vi "all signals list_search worksheet.vi"() -> ()   [LabVIEW 2020]
panel:
  out "path not found":bool
  in  "signal/tag name":string="RX_deltatime"
  out "full path name":string
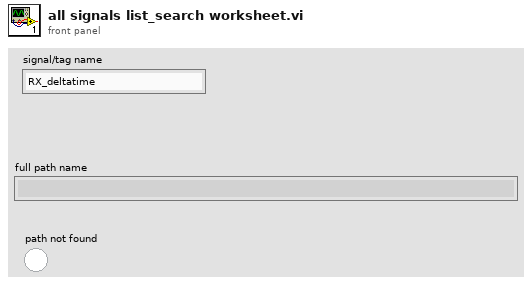
[diagram p1: front panel]
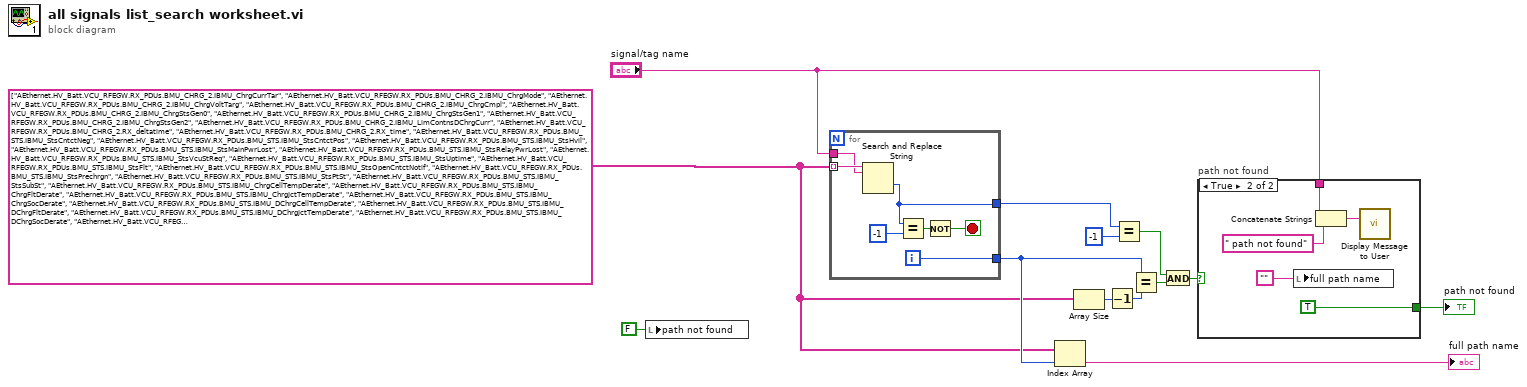
[diagram p0: block diagram]
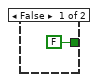
[diagram p2: hidden frame]
diagram:
  w1 = string[] ["AEthernet.HV_Batt.VCU_RFEGW.RX_PDUs.BMU_CHRG_2.IBMU_ChrgCurrTar", "AEthernet.HV_Batt.VCU_RFEGW.RX_PDUs.BMU_CHRG_2.IBMU_ChrgMode", "AEthernet.HV_Batt.VCU_RFEGW.RX_PDUs.BMU_CHRG_2.IBMU_ChrgVoltTarg", "AEthernet.HV_Batt.VCU_RFEGW.RX_PDUs.BMU_CHRG_2.IBMU_ChrgCmpl", "AEthernet.HV_Batt.VCU_RFEGW.RX_PDUs.BMU_CHRG_2.IBMU_ChrgStsGen0", "AEthernet.HV_Batt.VCU_RFEGW.RX_PDUs.BMU_CHRG_2.IBMU_ChrgStsGen1", "AEthernet.HV_Batt.VCU_RFEGW.RX_PDUs.BMU_CHRG_2.IBMU_ChrgStsGen2", "AEthernet.HV_Batt.VCU_RFEGW.RX_PDUs.BMU_CHRG_2.IBMU_LimContnsDChrgCurr", "AEthernet.HV_Batt.VCU_RFEGW.RX_PDUs.BMU_CHRG_2.RX_deltatime", "AEthernet.HV_Batt.VCU_RFEGW.RX_PDUs.BMU_CHRG_2.RX_time", "AEthernet.HV_Batt.VCU_RFEGW.RX_PDUs.BMU_STS.IBMU_StsCntctNeg", "AEthernet.HV_Batt.VCU_RFEGW.RX_PDUs.BMU_STS.IBMU_StsCntctPos", "AEthernet.HV_Batt.VCU_RFEGW.RX_PDUs.BMU_STS.IBMU_StsHvil", "AEthernet.HV_Batt.VCU_RFEGW.RX_PDUs.BMU_STS.IBMU_StsMainPwrLost", "AEthernet.HV_Batt.VCU_RFEGW.RX_PDUs.BMU_STS.IBMU_StsRelayPwrLost", "AEthernet.HV_Batt.VCU_RFEGW.RX_PDUs.BMU_STS.IBMU_StsVcuStReq", "AEthernet.HV_Batt.VCU_RFEGW.RX_PDUs.BMU_STS.IBMU_StsUptime", "AEthernet.HV_Batt.VCU_RFEGW.RX_PDUs.BMU_STS.IBMU_StsFlt", "AEthernet.HV_Batt.VCU_RFEGW.RX_PDUs.BMU_STS.IBMU_StsOpenCntctNotif", "AEthernet.HV_Batt.VCU_RFEGW.RX_PDUs.BMU_STS.IBMU_StsPrechrgn", "AEthernet.HV_Batt.VCU_RFEGW.RX_PDUs.BMU_STS.IBMU_StsPtSt", "AEthernet.HV_Batt.VCU_RFEGW.RX_PDUs.BMU_STS.IBMU_StsSubSt", "AEthernet.HV_Batt.VCU_RFEGW.RX_PDUs.BMU_STS.IBMU_ChrgCellTempDerate", "AEthernet.HV_Batt.VCU_RFEGW.RX_PDUs.BMU_STS.IBMU_ChrgFltDerate", "AEthernet.HV_Batt.VCU_RFEGW.RX_PDUs.BMU_STS.IBMU_ChrgJctTempDerate", "AEthernet.HV_Batt.VCU_RFEGW.RX_PDUs.BMU_STS.IBMU_ChrgSocDerate", "AEthernet.HV_Batt.VCU_RFEGW.RX_PDUs.BMU_STS.IBMU_DChrgCellTempDerate", "AEthernet.HV_Batt.VCU_RFEGW.RX_PDUs.BMU_STS.IBMU_DChrgFltDerate", "AEthernet.HV_Batt.VCU_RFEGW.RX_PDUs.BMU_STS.IBMU_DChrgJctTempDerate", "AEthernet.HV_Batt.VCU_RFEGW.RX_PDUs.BMU_STS.IBMU_DChrgSocDerate", "AEthernet.HV_Batt.VCU_RFEGW.RX_PDUs.BMU_STS.RX_deltatime", "AEthernet.HV_Batt.VCU_RFEGW.RX_PDUs.BMU_STS.RX_time", "AEthernet.HV_Batt.TCU.RX_PDUs.BMU_CHRG_2.IBMU_ChrgCurrTar", "AEthernet.HV_Batt.TCU.RX_PDUs.BMU_CHRG_2.IBMU_ChrgMode", "AEthernet.HV_Batt.TCU.RX_PDUs.BMU_CHRG_2.IBMU_ChrgVoltTarg", "AEthernet.HV_Batt.TCU.RX_PDUs.BMU_CHRG_2.IBMU_ChrgCmpl", "AEthernet.HV_Batt.TCU.RX_PDUs.BMU_CHRG_2.IBMU_ChrgStsGen0", "AEthernet.HV_Batt.TCU.RX_PDUs.BMU_CHRG_2.IBMU_ChrgStsGen1", "AEthernet.HV_Batt.TCU.RX_PDUs.BMU_CHRG_2.IBMU_ChrgStsGen2", "AEthernet.HV_Batt.TCU.RX_PDUs.BMU_CHRG_2.IBMU_LimContnsDChrgCurr", "AEthernet.HV_Batt.TCU.RX_PDUs.BMU_CHRG_2.RX_deltatime", "AEthernet.HV_Batt.TCU.RX_PDUs.BMU_CHRG_2.RX_time", "AEthernet.HV_Batt.TCU.RX_PDUs.BMU_CHRG_3.IBMU_LimMaxChrgCurr", "AEthernet.HV_Batt.TCU.RX_PDUs.BMU_CHRG_3.IBMU_LimMaxChrgPwr", "AEthernet.HV_Batt.TCU.RX_PDUs.BMU_CHRG_3.IBMU_LimMaxChrgVolt", "AEthernet.HV_Batt.TCU.RX_PDUs.BMU_CHRG_3.IBMU_LimMinChrgCurr", "AEthernet.HV_Batt.TCU.RX_PDUs.BMU_CHRG_3.RX_deltatime", "AEthernet.HV_Batt.TCU.RX_PDUs.BMU_CHRG_3.RX_time", "AEthernet.HV_Batt.TCU.RX_PDUs.BMU_DIAG_RESP.IDiagRspRes1", "AEthernet.HV_Batt.TCU.RX_PDUs.BMU_DIAG_RESP.IDiagRspRes2", "AEthernet.HV_Batt.TCU.RX_PDUs.BMU_DIAG_RESP.IDiagRspRes3", "AEthernet.HV_Batt.TCU.RX_PDUs.BMU_DIAG_RESP.IDiagRspRes4", "AEthernet.HV_Batt.TCU.RX_PDUs.BMU_DIAG_RESP.IDiagRspRes5", "AEthernet.HV_Batt.TCU.RX_PDUs.BMU_DIAG_RESP.IDiagRspRes6", "AEthernet.HV_Batt.TCU.RX_PDUs.BMU_DIAG_RESP.IDiagRspRes7", "AEthernet.HV_Batt.TCU.RX_PDUs.BMU_DIAG_RESP.IDiagRspRoutId", "AEthernet.HV_Batt.TCU.RX_PDUs.BMU_DIAG_RESP.IDiagRspSts", "AEthernet.HV_Batt.TCU.RX_PDUs.BMU_DIAG_RESP.RX_deltatime", "AEthernet.HV_Batt.TCU.RX_PDUs.BMU_DIAG_RESP.RX_time", "AEthernet.HV_Batt.TCU.RX_PDUs.BMU_DbgGen_1.IBMU_DbgGen_B0", "AEthernet.HV_Batt.TCU.RX_PDUs.BMU_DbgGen_1.IBMU_DbgGen_B1", "AEthernet.HV_Batt.TCU.RX_PDUs.BMU_DbgGen_1.IBMU_DbgGen_B2", "AEthernet.HV_Batt.TCU.RX_PDUs.BMU_DbgGen_1.IBMU_DbgGen_B3", "AEthernet.HV_Batt.TCU.RX_PDUs.BMU_DbgGen_1.IBMU_DbgGen_B4", "AEthernet.HV_Batt.TCU.RX_PDUs.BMU_DbgGen_1.IBMU_DbgGen_B5", "AEthernet.HV_Batt.TCU.RX_PDUs.BMU_DbgGen_1.IBMU_DbgGen_B6", "AEthernet.HV_Batt.TCU.RX_PDUs.BMU_DbgGen_1.IBMU_DbgGen_B7", "AEthernet.HV_Batt.TCU.RX_PDUs.BMU_DbgGen_1.IBMU_DbgGen_B8", "AEthernet.HV_Batt.TCU.RX_PDUs.BMU_DbgGen_1.IBMU_DbgGen_B9", "AEthernet.HV_Batt.TCU.RX_PDUs.BMU_DbgGen_1.IBMU_DbgGen_L0", "AEthernet.HV_Batt.TCU.RX_PDUs.BMU_DbgGen_1.IBMU_DbgGen_L1", "AEthernet.HV_Batt.TCU.RX_PDUs.BMU_DbgGen_1.IBMU_DbgGen_L2", "AEthernet.HV_Batt.TCU.RX_PDUs.BMU_DbgGen_1.IBMU_DbgGen_L3", "AEthernet.HV_Batt.TCU.RX_PDUs.BMU_DbgGen_1.IBMU_DbgGen_S0", "AEthernet.HV_Batt.TCU.RX_PDUs.BMU_DbgGen_1.IBMU_DbgGen_S1", "AEthernet.HV_Batt.TCU.RX_PDUs.BMU_DbgGen_1.IBMU_DbgGen_S2", "AEthernet.HV_Batt.TCU.RX_PDUs.BMU_DbgGen_1.IBMU_DbgGen_S3", "AEthernet.HV_Batt.TCU.RX_PDUs.BMU_DbgGen_1.IBMU_DbgGen_S4", "AEthernet.HV_Batt.TCU.RX_PDUs.BMU_DbgGen_1.IBMU_DbgGen_S5", "AEthernet.HV_Batt.TCU.RX_PDUs.BMU_DbgGen_1.IBMU_DbgGen_S6", "AEthernet.HV_Batt.TCU.RX_PDUs.BMU_DbgGen_1.IBMU_DbgGen_S7", "AEthernet.HV_Batt.TCU.RX_PDUs.BMU_DbgGen_1.IBMU_DbgGen_S8", "AEthernet.HV_Batt.TCU.RX_PDUs.BMU_DbgGen_1.IBMU_DbgGen_S9", "AEthernet.HV_Batt.TCU.RX_PDUs.BMU_DbgGen_1.IBMU_DbgGen_W00", "AEthernet.HV_Batt.TCU.RX_PDUs.BMU_DbgGen_1.IBMU_DbgGen_W01", "AEthernet.HV_Batt.TCU.RX_PDUs.BMU_DbgGen_1.IBMU_DbgGen_W02", "AEthernet.HV_Batt.TCU.RX_PDUs.BMU_DbgGen_1.IBMU_DbgGen_W03", "AEthernet.HV_Batt.TCU.RX_PDUs.BMU_DbgGen_1.IBMU_DbgGen_W04", "AEthernet.HV_Batt.TCU.RX_PDUs.BMU_DbgGen_1.IBMU_DbgGen_W05", "AEthernet.HV_Batt.TCU.RX_PDUs.BMU_DbgGen_1.IBMU_DbgGen_W06", "AEthernet.HV_Batt.TCU.RX_PDUs.BMU_DbgGen_1.IBMU_DbgGen_W07", "AEthernet.HV_Batt.TCU.RX_PDUs.BMU_DbgGen_1.IBMU_DbgGen_W08", "AEthernet.HV_Batt.TCU.RX_PDUs.BMU_DbgGen_1.IBMU_DbgGen_W09", "AEthernet.HV_Batt.TCU.RX_PDUs.BMU_DbgGen_1.IBMU_DbgGen_W10", "AEthernet.HV_Batt.TCU.RX_PDUs.BMU_DbgGen_1.IBMU_DbgGen_W11", "AEthernet.HV_Batt.TCU.RX_PDUs.BMU_DbgGen_1.IBMU_DbgGen_W12", "AEthernet.HV_Batt.TCU.RX_PDUs.BMU_DbgGen_1.IBMU_DbgGen_W13", "AEthernet.HV_Batt.TCU.RX_PDUs.BMU_DbgGen_1.IBMU_DbgGen_W14", "AEthernet.HV_Batt.TCU.RX_PDUs.BMU_DbgGen_1.IBMU_DbgGen_W15", "AEthernet.HV_Batt.TCU.RX_PDUs.BMU_DbgGen_1.RX_deltatime", "AEthernet.HV_Batt.TCU.RX_PDUs.BMU_DbgGen_1.RX_time", "AEthernet.HV_Batt.TCU.RX_PDUs.BMU_DbgGen_2.IBMU_DbgIsoSampleVneg", "AEthernet.HV_Batt.TCU.RX_PDUs.BMU_DbgGen_2.IBMU_DbgIsoSampleVpos", "AEthernet.HV_Batt.TCU.RX_PDUs.BMU_DbgGen_2.IBMU_DbgIsoSampleVsum", "AEthernet.HV_Batt.TCU.RX_PDUs.BMU_DbgGen_2.IBMU_DbgGen_W16", "AEthernet.HV_Batt.TCU.RX_PDUs.BMU_DbgGen_2.IBMU_DbgGen_W17", "AEthernet.HV_Batt.TCU.RX_PDUs.BMU_DbgGen_2.IBMU_DbgGen_W18", "AEthernet.HV_Batt.TCU.RX_PDUs.BMU_DbgGen_2.IBMU_DbgGen_W19", "AEthernet.HV_Batt.TCU.RX_PDUs.BMU_DbgGen_2.IBMU_DbgPktRetryCnt", "AEthernet.HV_Batt.TCU.RX_PDUs.BMU_DbgGen_2.RX_deltatime", "AEthernet.HV_Batt.TCU.RX_PDUs.BMU_DbgGen_2.RX_time", "AEthernet.HV_Batt.TCU.RX_PDUs.BMU_DbgVers.IBMU_DbgHw", "AEthernet.HV_Batt.TCU.RX_PDUs.BMU_DbgVers.IBMU_DbgSwMajor", "AEthernet.HV_Batt.TCU.RX_PDUs.BMU_DbgVers.IBMU_DbgSwMicro", "AEthernet.HV_Batt.TCU.RX_PDUs.BMU_DbgVers.IBMU_DbgSwMinor", "AEthernet.HV_Batt.TCU.RX_PDUs.BMU_DbgVers.IBMU_DbgFpgaMajor", "AEthernet.HV_Batt.TCU.RX_PDUs.BMU_DbgVers.IBMU_DbgFpgaMinor", "AEthernet.HV_Batt.TCU.RX_PDUs.BMU_DbgVers.IBMU_StatsPkSrlNum", "AEthernet.HV_Batt.TCU.RX_PDUs.BMU_DbgVers.IBMU_DbgTsuMaxMajor", "AEthernet.HV_Batt.TCU.RX_PDUs.BMU_DbgVers.IBMU_DbgTsuMaxMicro", "AEthernet.HV_Batt.TCU.RX_PDUs.BMU_DbgVers.IBMU_DbgTsuMaxMinor", "AEthernet.HV_Batt.TCU.RX_PDUs.BMU_DbgVers.IBMU_DbgTsuMaxRels", "AEthernet.HV_Batt.TCU.RX_PDUs.BMU_DbgVers.IBMU_DbgTsuMinMajor", "AEthernet.HV_Batt.TCU.RX_PDUs.BMU_DbgVers.IBMU_DbgTsuMinMicro", "AEthernet.HV_Batt.TCU.RX_PDUs.BMU_DbgVers.IBMU_DbgTsuMinMinor", "AEthernet.HV_Batt.TCU.RX_PDUs.BMU_DbgVers.IBMU_DbgTsuMinRels", "AEthernet.HV_Batt.TCU.RX_PDUs.BMU_DbgVers.RX_deltatime", "AEthernet.HV_Batt.TCU.RX_PDUs.BMU_DbgVers.RX_time", "AEthernet.HV_Batt.TCU.RX_PDUs.BMU_FLT_1.IBMU_FltAcb", "AEthernet.HV_Batt.TCU.RX_PDUs.BMU_FLT_1.IBMU_FltBlkVoltOver", "AEthernet.HV_Batt.TCU.RX_PDUs.BMU_FLT_1.IBMU_FltBlkVoltUnder", "AEthernet.HV_Batt.TCU.RX_PDUs.BMU_FLT_1.IBMU_FltConds", "AEthernet.HV_Batt.TCU.RX_PDUs.BMU_FLT_1.IBMU_FltHvil", "AEthernet.HV_Batt.TCU.RX_PDUs.BMU_FLT_1.IBMU_FltIso", "AEthernet.HV_Batt.TCU.RX_PDUs.BMU_FLT_1.IBMU_FltModCnt", "AEthernet.HV_Batt.TCU.RX_PDUs.BMU_FLT_1.IBMU_FltPkCurrOver", "AEthernet.HV_Batt.TCU.RX_PDUs.BMU_FLT_1.IBMU_FltPkCurrUnder", "AEthernet.HV_Batt.TCU.RX_PDUs.BMU_FLT_1.IBMU_FltPkVoltOver", "AEthernet.HV_Batt.TCU.RX_PDUs.BMU_FLT_1.IBMU_FltPkVoltUnder", "AEthernet.HV_Batt.TCU.RX_PDUs.BMU_FLT_1.IBMU_FltPrechrg", "AEthernet.HV_Batt.TCU.RX_PDUs.BMU_FLT_1.IBMU_FltStSenClsd", "AEthernet.HV_Batt.TCU.RX_PDUs.BMU_FLT_1.IBMU_FltTempCellOver", "AEthernet.HV_Batt.TCU.RX_PDUs.BMU_FLT_1.IBMU_FltTempCellUnder", "AEthernet.HV_Batt.TCU.RX_PDUs.BMU_FLT_1.IBMU_FltTempInterconOver", "AEthernet.HV_Batt.TCU.RX_PDUs.BMU_FLT_1.IBMU_FltBlkVoltDelta", "AEthernet.HV_Batt.TCU.RX_PDUs.BMU_FLT_1.IBMU_FltStSenOpen", "AEthernet.HV_Batt.TCU.RX_PDUs.BMU_FLT_1.IBMU_StsFltHist1", "AEthernet.HV_Batt.TCU.RX_PDUs.BMU_FLT_1.IBMU_StsFltHist2", "AEthernet.HV_Batt.TCU.RX_PDUs.BMU_FLT_1.IBMU_StsFltHist3", "AEthernet.HV_Batt.TCU.RX_PDUs.BMU_FLT_1.IBMU_DbgRstSrc", "AEthernet.HV_Batt.TCU.RX_PDUs.BMU_FLT_1.IBMU_FltCntctHlth", "AEthernet.HV_Batt.TCU.RX_PDUs.BMU_FLT_1.IBMU_FltCrash", "AEthernet.HV_Batt.TCU.RX_PDUs.BMU_FLT_1.IBMU_FltPOver", "AEthernet.HV_Batt.TCU.RX_PDUs.BMU_FLT_1.IBMU_FltPyro", "AEthernet.HV_Batt.TCU.RX_PDUs.BMU_FLT_1.IBMU_FltShunt", "AEthernet.HV_Batt.TCU.RX_PDUs.BMU_FLT_1.IBMU_FltSpi", "AEthernet.HV_Batt.TCU.RX_PDUs.BMU_FLT_1.RX_deltatime", "AEthernet.HV_Batt.TCU.RX_PDUs.BMU_FLT_1.RX_time", "AEthernet.HV_Batt.TCU.RX_PDUs.BMU_FLT_2.IBMU_HsFltLogEstopTrckrSt", "AEthernet.HV_Batt.TCU.RX_PDUs.BMU_FLT_2.IBMU_HsFltLogPyroFired", "AEthernet.HV_Batt.TCU.RX_PDUs.BMU_FLT_2.IBMU_HsFltLogPyroStsBad", "AEthernet.HV_Batt.TCU.RX_PDUs.BMU_FLT_2.IBMU_HsFltLogRawEstop", "AEthernet.HV_Batt.TCU.RX_PDUs.BMU_FLT_2.IBMU_HsFltLogRawCurr", "AEthernet.HV_Batt.TCU.RX_PDUs.BMU_FLT_2.IBMU_HsFltLogReserved1", "AEthernet.HV_Batt.TCU.RX_PDUs.BMU_FLT_2.IBMU_HsFltLogReserved2", "AEthernet.HV_Batt.TCU.RX_PDUs.BMU_FLT_2.RX_deltatime", "AEthernet.HV_Batt.TCU.RX_PDUs.BMU_FLT_2.RX_time", "AEthernet.HV_Batt.TCU.RX_PDUs.BMU_MODBLKVOLT.IBMU_ModBlkVolt_M00B00", "AEthernet.HV_Batt.TCU.RX_PDUs.BMU_MODBLKVOLT.IBMU_ModBlkVolt_M00B01", "AEthernet.HV_Batt.TCU.RX_PDUs.BMU_MODBLKVOLT.IBMU_ModBlkVolt_M00B02", "AEthernet.HV_Batt.TCU.RX_PDUs.BMU_MODBLKVOLT.IBMU_ModBlkVolt_M00B03", "AEthernet.HV_Batt.TCU.RX_PDUs.BMU_MODBLKVOLT.IBMU_ModBlkVolt_M00B04", "AEthernet.HV_Batt.TCU.RX_PDUs.BMU_MODBLKVOLT.IBMU_ModBlkVolt_M00B05", "AEthernet.HV_Batt.TCU.RX_PDUs.BMU_MODBLKVOLT.IBMU_ModBlkVolt_M00B06", "AEthernet.HV_Batt.TCU.RX_PDUs.BMU_MODBLKVOLT.IBMU_ModBlkVolt_M00B07", "AEthernet.HV_Batt.TCU.RX_PDUs.BMU_MODBLKVOLT.IBMU_ModBlkVolt_M00B08", "AEthernet.HV_Batt.TCU.RX_PDUs.BMU_MODBLKVOLT.IBMU_ModBlkVolt_M00B09", "AEthernet.HV_Batt.TCU.RX_PDUs.BMU_MODBLKVOLT.IBMU_ModBlkVolt_M01B00", "AEthernet.HV_Batt.TCU.RX_PDUs.BMU_MODBLKVOLT.IBMU_ModBlkVolt_M01B01", "AEthernet.HV_Batt.TCU.RX_PDUs.BMU_MODBLKVOLT.IBMU_ModBlkVolt_M01B02", "AEthernet.HV_Batt.TCU.RX_PDUs.BMU_MODBLKVOLT.IBMU_ModBlkVolt_M01B03", "AEthernet.HV_Batt.TCU.RX_PDUs.BMU_MODBLKVOLT.IBMU_ModBlkVolt_M01B04", "AEthernet.HV_Batt.TCU.RX_PDUs.BMU_MODBLKVOLT.IBMU_ModBlkVolt_M01B05", "AEthernet.HV_Batt.TCU.RX_PDUs.BMU_MODBLKVOLT.IBMU_ModBlkVolt_M01B06", "AEthernet.HV_Batt.TCU.RX_PDUs.BMU_MODBLKVOLT.IBMU_ModBlkVolt_M01B07", "AEthernet.HV_Batt.TCU.RX_PDUs.BMU_MODBLKVOLT.IBMU_ModBlkVolt_M01B08", "AEthernet.HV_Batt.TCU.RX_PDUs.BMU_MODBLKVOLT.IBMU_ModBlkVolt_M01B09", "AEthernet.HV_Batt.TCU.RX_PDUs.BMU_MODBLKVOLT.IBMU_ModBlkVolt_M02B00", "AEthernet.HV_Batt.TCU.RX_PDUs.BMU_MODBLKVOLT.IBMU_ModBlkVolt_M02B01", "AEthernet.HV_Batt.TCU.RX_PDUs.BMU_MODBLKVOLT.IBMU_ModBlkVolt_M02B02", "AEthernet.HV_Batt.TCU.RX_PDUs.BMU_MODBLKVOLT.IBMU_ModBlkVolt_M02B03", "AEthernet.HV_Batt.TCU.RX_PDUs.BMU_MODBLKVOLT.IBMU_ModBlkVolt_M02B04", "AEthernet.HV_Batt.TCU.RX_PDUs.BMU_MODBLKVOLT.IBMU_ModBlkVolt_M02B05", "AEthernet.HV_Batt.TCU.RX_PDUs.BMU_MODBLKVOLT.IBMU_ModBlkVolt_M02B06", "AEthernet.HV_Batt.TCU.RX_PDUs.BMU_MODBLKVOLT.IBMU_ModBlkVolt_M02B07", "AEthernet.HV_Batt.TCU.RX_PDUs.BMU_MODBLKVOLT.IBMU_ModBlkVolt_M02B08", "AEthernet.HV_Batt.TCU.RX_PDUs.BMU_MODBLKVOLT.IBMU_ModBlkVolt_M02B09", "AEthernet.HV_Batt.TCU.RX_PDUs.BMU_MODBLKVOLT.IBMU_ModBlkVolt_M03B00", "AEthernet.HV_Batt.TCU.RX_PDUs.BMU_MODBLKVOLT.IBMU_ModBlkVolt_M03B01", "AEthernet.HV_Batt.TCU.RX_PDUs.BMU_MODBLKVOLT.IBMU_ModBlkVolt_M03B02", "AEthernet.HV_Batt.TCU.RX_PDUs.BMU_MODBLKVOLT.IBMU_ModBlkVolt_M03B03", "AEthernet.HV_Batt.TCU.RX_PDUs.BMU_MODBLKVOLT.IBMU_ModBlkVolt_M03B04", "AEthernet.HV_Batt.TCU.RX_PDUs.BMU_MODBLKVOLT.IBMU_ModBlkVolt_M03B05", "AEthernet.HV_Batt.TCU.RX_PDUs.BMU_MODBLKVOLT.IBMU_ModBlkVolt_M03B06", "AEthernet.HV_Batt.TCU.RX_PDUs.BMU_MODBLKVOLT.IBMU_ModBlkVolt_M03B07", "AEthernet.HV_Batt.TCU.RX_PDUs.BMU_MODBLKVOLT.IBMU_ModBlkVolt_M03B08", "AEthernet.HV_Batt.TCU.RX_PDUs.BMU_MODBLKVOLT.IBMU_ModBlkVolt_M03B09", "AEthernet.HV_Batt.TCU.RX_PDUs.BMU_MODBLKVOLT.IBMU_ModBlkVolt_M04B00", "AEthernet.HV_Batt.TCU.RX_PDUs.BMU_MODBLKVOLT.IBMU_ModBlkVolt_M04B01", "AEthernet.HV_Batt.TCU.RX_PDUs.BMU_MODBLKVOLT.IBMU_ModBlkVolt_M04B02", "AEthernet.HV_Batt.TCU.RX_PDUs.BMU_MODBLKVOLT.IBMU_ModBlkVolt_M04B03", "AEthernet.HV_Batt.TCU.RX_PDUs.BMU_MODBLKVOLT.IBMU_ModBlkVolt_M04B04", "AEthernet.HV_Batt.TCU.RX_PDUs.BMU_MODBLKVOLT.IBMU_ModBlkVolt_M04B05", "AEthernet.HV_Batt.TCU.RX_PDUs.BMU_MODBLKVOLT.IBMU_ModBlkVolt_M04B06", "AEthernet.HV_Batt.TCU.RX_PDUs.BMU_MODBLKVOLT.IBMU_ModBlkVolt_M04B07", "AEthernet.HV_Batt.TCU.RX_PDUs.BMU_MODBLKVOLT.IBMU_ModBlkVolt_M04B08", "AEthernet.HV_Batt.TCU.RX_PDUs.BMU_MODBLKVOLT.IBMU_ModBlkVolt_M04B09", "AEthernet.HV_Batt.TCU.RX_PDUs.BMU_MODBLKVOLT.IBMU_ModBlkVolt_M05B00", "AEthernet.HV_Batt.TCU.RX_PDUs.BMU_MODBLKVOLT.IBMU_ModBlkVolt_M05B01", "AEthernet.HV_Batt.TCU.RX_PDUs.BMU_MODBLKVOLT.IBMU_ModBlkVolt_M05B02", "AEthernet.HV_Batt.TCU.RX_PDUs.BMU_MODBLKVOLT.IBMU_ModBlkVolt_M05B03", "AEthernet.HV_Batt.TCU.RX_PDUs.BMU_MODBLKVOLT.IBMU_ModBlkVolt_M05B04", "AEthernet.HV_Batt.TCU.RX_PDUs.BMU_MODBLKVOLT.IBMU_ModBlkVolt_M05B05", "AEthernet.HV_Batt.TCU.RX_PDUs.BMU_MODBLKVOLT.IBMU_ModBlkVolt_M05B06", "AEthernet.HV_Batt.TCU.RX_PDUs.BMU_MODBLKVOLT.IBMU_ModBlkVolt_M05B07", "AEthernet.HV_Batt.TCU.RX_PDUs.BMU_MODBLKVOLT.IBMU_ModBlkVolt_M05B08", "AEthernet.HV_Batt.TCU.RX_PDUs.BMU_MODBLKVOLT.IBMU_ModBlkVolt_M05B09", "AEthernet.HV_Batt.TCU.RX_PDUs.BMU_MODBLKVOLT.IBMU_ModBlkVolt_M06B00", "AEthernet.HV_Batt.TCU.RX_PDUs.BMU_MODBLKVOLT.IBMU_ModBlkVolt_M06B01", "AEthernet.HV_Batt.TCU.RX_PDUs.BMU_MODBLKVOLT.IBMU_ModBlkVolt_M06B02", "AEthernet.HV_Batt.TCU.RX_PDUs.BMU_MODBLKVOLT.IBMU_ModBlkVolt_M06B03", "AEthernet.HV_Batt.TCU.RX_PDUs.BMU_MODBLKVOLT.IBMU_ModBlkVolt_M06B04", "AEthernet.HV_Batt.TCU.RX_PDUs.BMU_MODBLKVOLT.IBMU_ModBlkVolt_M06B05", "AEthernet.HV_Batt.TCU.RX_PDUs.BMU_MODBLKVOLT.IBMU_ModBlkVolt_M06B06", "AEthernet.HV_Batt.TCU.RX_PDUs.BMU_MODBLKVOLT.IBMU_ModBlkVolt_M06B07", "AEthernet.HV_Batt.TCU.RX_PDUs.BMU_MODBLKVOLT.IBMU_ModBlkVolt_M06B08", "AEthernet.HV_Batt.TCU.RX_PDUs.BMU_MODBLKVOLT.IBMU_ModBlkVolt_M06B09", "AEthernet.HV_Batt.TCU.RX_PDUs.BMU_MODBLKVOLT.IBMU_ModBlkVolt_M07B00", "AEthernet.HV_Batt.TCU.RX_PDUs.BMU_MODBLKVOLT.IBMU_ModBlkVolt_M07B01", "AEthernet.HV_Batt.TCU.RX_PDUs.BMU_MODBLKVOLT.IBMU_ModBlkVolt_M07B02", "AEthernet.HV_Batt.TCU.RX_PDUs.BMU_MODBLKVOLT.IBMU_ModBlkVolt_M07B03", "AEthernet.HV_Batt.TCU.RX_PDUs.BMU_MODBLKVOLT.IBMU_ModBlkVolt_M07B04", "AEthernet.HV_Batt.TCU.RX_PDUs.BMU_MODBLKVOLT.IBMU_ModBlkVolt_M07B05", "AEthernet.HV_Batt.TCU.RX_PDUs.BMU_MODBLKVOLT.IBMU_ModBlkVolt_M07B06", "AEthernet.HV_Batt.TCU.RX_PDUs.BMU_MODBLKVOLT.IBMU_ModBlkVolt_M07B07", "AEthernet.HV_Batt.TCU.RX_PDUs.BMU_MODBLKVOLT.IBMU_ModBlkVolt_M07B08", "AEthernet.HV_Batt.TCU.RX_PDUs.BMU_MODBLKVOLT.IBMU_ModBlkVolt_M07B09", "AEthernet.HV_Batt.TCU.RX_PDUs.BMU_MODBLKVOLT.IBMU_ModBlkVolt_M08B00", "AEthernet.HV_Batt.TCU.RX_PDUs.BMU_MODBLKVOLT.IBMU_ModBlkVolt_M08B01", "AEthernet.HV_Batt.TCU.RX_PDUs.BMU_MODBLKVOLT.IBMU_ModBlkVolt_M08B02", "AEthernet.HV_Batt.TCU.RX_PDUs.BMU_MODBLKVOLT.IBMU_ModBlkVolt_M08B03", "AEthernet.HV_Batt.TCU.RX_PDUs.BMU_MODBLKVOLT.IBMU_ModBlkVolt_M08B04", "AEthernet.HV_Batt.TCU.RX_PDUs.BMU_MODBLKVOLT.IBMU_ModBlkVolt_M08B05", "AEthernet.HV_Batt.TCU.RX_PDUs.BMU_MODBLKVOLT.IBMU_ModBlkVolt_M08B06", "AEthernet.HV_Batt.TCU.RX_PDUs.BMU_MODBLKVOLT.IBMU_ModBlkVolt_M08B07", "AEthernet.HV_Batt.TCU.RX_PDUs.BMU_MODBLKVOLT.IBMU_ModBlkVolt_M08B08", "AEthernet.HV_Batt.TCU.RX_PDUs.BMU_MODBLKVOLT.IBMU_ModBlkVolt_M08B09", "AEthernet.HV_Batt.TCU.RX_PDUs.BMU_MODBLKVOLT.IBMU_ModBlkVolt_M09B00", "AEthernet.HV_Batt.TCU.RX_PDUs.BMU_MODBLKVOLT.IBMU_ModBlkVolt_M09B01", "AEthernet.HV_Batt.TCU.RX_PDUs.BMU_MODBLKVOLT.IBMU_ModBlkVolt_M09B02", "AEthernet.HV_Batt.TCU.RX_PDUs.BMU_MODBLKVOLT.IBMU_ModBlkVolt_M09B03", "AEthernet.HV_Batt.TCU.RX_PDUs.BMU_MODBLKVOLT.IBMU_ModBlkVolt_M09B04", "AEthernet.HV_Batt.TCU.RX_PDUs.BMU_MODBLKVOLT.IBMU_ModBlkVolt_M09B05", "AEthernet.HV_Batt.TCU.RX_PDUs.BMU_MODBLKVOLT.IBMU_ModBlkVolt_M09B06", "AEthernet.HV_Batt.TCU.RX_PDUs.BMU_MODBLKVOLT.IBMU_ModBlkVolt_M09B07", "AEthernet.HV_Batt.TCU.RX_PDUs.BMU_MODBLKVOLT.IBMU_ModBlkVolt_M09B08", "AEthernet.HV_Batt.TCU.RX_PDUs.BMU_MODBLKVOLT.IBMU_ModBlkVolt_M09B09", "AEthernet.HV_Batt.TCU.RX_PDUs.BMU_MODBLKVOLT.IBMU_ModBlkVolt_M10B00", "AEthernet.HV_Batt.TCU.RX_PDUs.BMU_MODBLKVOLT.IBMU_ModBlkVolt_M10B01", "AEthernet.HV_Batt.TCU.RX_PDUs.BMU_MODBLKVOLT.IBMU_ModBlkVolt_M10B02", "AEthernet.HV_Batt.TCU.RX_PDUs.BMU_MODBLKVOLT.IBMU_ModBlkVolt_M10B03", "AEthernet.HV_Batt.TCU.RX_PDUs.BMU_MODBLKVOLT.IBMU_ModBlkVolt_M10B04", "AEthernet.HV_Batt.TCU.RX_PDUs.BMU_MODBLKVOLT.IBMU_ModBlkVolt_M10B05", "AEthernet.HV_Batt.TCU.RX_PDUs.BMU_MODBLKVOLT.IBMU_ModBlkVolt_M10B06", "AEthernet.HV_Batt.TCU.RX_PDUs.BMU_MODBLKVOLT.IBMU_ModBlkVolt_M10B07", "AEthernet.HV_Batt.TCU.RX_PDUs.BMU_MODBLKVOLT.IBMU_ModBlkVolt_M10B08", "AEthernet.HV_Batt.TCU.RX_PDUs.BMU_MODBLKVOLT.IBMU_ModBlkVolt_M10B09", "AEthernet.HV_Batt.TCU.RX_PDUs.BMU_MODBLKVOLT.IBMU_ModBlkVolt_M11B00", "AEthernet.HV_Batt.TCU.RX_PDUs.BMU_MODBLKVOLT.IBMU_ModBlkVolt_M11B01", "AEthernet.HV_Batt.TCU.RX_PDUs.BMU_MODBLKVOLT.IBMU_ModBlkVolt_M11B02", "AEthernet.HV_Batt.TCU.RX_PDUs.BMU_MODBLKVOLT.IBMU_ModBlkVolt_M11B03", "AEthernet.HV_Batt.TCU.RX_PDUs.BMU_MODBLKVOLT.IBMU_ModBlkVolt_M11B04", "AEthernet.HV_Batt.TCU.RX_PDUs.BMU_MODBLKVOLT.IBMU_ModBlkVolt_M11B05", "AEthernet.HV_Batt.TCU.RX_PDUs.BMU_MODBLKVOLT.IBMU_ModBlkVolt_M11B06", "AEthernet.HV_Batt.TCU.RX_PDUs.BMU_MODBLKVOLT.IBMU_ModBlkVolt_M11B07", "AEthernet.HV_Batt.TCU.RX_PDUs.BMU_MODBLKVOLT.IBMU_ModBlkVolt_M11B08", "AEthernet.HV_Batt.TCU.RX_PDUs.BMU_MODBLKVOLT.IBMU_ModBlkVolt_M11B09", "AEthernet.HV_Batt.TCU.RX_PDUs.BMU_MODBLKVOLT.IBMU_ModBlkVolt_M12B00", "AEthernet.HV_Batt.TCU.RX_PDUs.BMU_MODBLKVOLT.IBMU_ModBlkVolt_M12B01", "AEthernet.HV_Batt.TCU.RX_PDUs.BMU_MODBLKVOLT.IBMU_ModBlkVolt_M12B02", "AEthernet.HV_Batt.TCU.RX_PDUs.BMU_MODBLKVOLT.IBMU_ModBlkVolt_M12B03", "AEthernet.HV_Batt.TCU.RX_PDUs.BMU_MODBLKVOLT.IBMU_ModBlkVolt_M12B04", "AEthernet.HV_Batt.TCU.RX_PDUs.BMU_MODBLKVOLT.IBMU_ModBlkVolt_M12B05", "AEthernet.HV_Batt.TCU.RX_PDUs.BMU_MODBLKVOLT.IBMU_ModBlkVolt_M12B06", "AEthernet.HV_Batt.TCU.RX_PDUs.BMU_MODBLKVOLT.IBMU_ModBlkVolt_M12B07", "AEthernet.HV_Batt.TCU.RX_PDUs.BMU_MODBLKVOLT.IBMU_ModBlkVolt_M12B08", "AEthernet.HV_Batt.TCU.RX_PDUs.BMU_MODBLKVOLT.IBMU_ModBlkVolt_M12B09", "AEthernet.HV_Batt.TCU.RX_PDUs.BMU_MODBLKVOLT.IBMU_ModBlkVolt_M13B00", "AEthernet.HV_Batt.TCU.RX_PDUs.BMU_MODBLKVOLT.IBMU_ModBlkVolt_M13B01", "AEthernet.HV_Batt.TCU.RX_PDUs.BMU_MODBLKVOLT.IBMU_ModBlkVolt_M13B02", "AEthernet.HV_Batt.TCU.RX_PDUs.BMU_MODBLKVOLT.IBMU_ModBlkVolt_M13B03", "AEthernet.HV_Batt.TCU.RX_PDUs.BMU_MODBLKVOLT.IBMU_ModBlkVolt_M13B04", "AEthernet.HV_Batt.TCU.RX_PDUs.BMU_MODBLKVOLT.IBMU_ModBlkVolt_M13B05", "AEthernet.HV_Batt.TCU.RX_PDUs.BMU_MODBLKVOLT.IBMU_ModBlkVolt_M13B06", "AEthernet.HV_Batt.TCU.RX_PDUs.BMU_MODBLKVOLT.IBMU_ModBlkVolt_M13B07", "AEthernet.HV_Batt.TCU.RX_PDUs.BMU_MODBLKVOLT.IBMU_ModBlkVolt_M13B08", "AEthernet.HV_Batt.TCU.RX_PDUs.BMU_MODBLKVOLT.IBMU_ModBlkVolt_M13B09", "AEthernet.HV_Batt.TCU.RX_PDUs.BMU_MODBLKVOLT.IBMU_ModBlkVolt_M14B00", "AEthernet.HV_Batt.TCU.RX_PDUs.BMU_MODBLKVOLT.IBMU_ModBlkVolt_M14B01", "AEthernet.HV_Batt.TCU.RX_PDUs.BMU_MODBLKVOLT.IBMU_ModBlkVolt_M14B02", "AEthernet.HV_Batt.TCU.RX_PDUs.BMU_MODBLKVOLT.IBMU_ModBlkVolt_M14B03", "AEthernet.HV_Batt.TCU.RX_PDUs.BMU_MODBLKVOLT.IBMU_ModBlkVolt_M14B04", "AEthernet.HV_Batt.TCU.RX_PDUs.BMU_MODBLKVOLT.IBMU_ModBlkVolt_M14B05", "AEthernet.HV_Batt.TCU.RX_PDUs.BMU_MODBLKVOLT.IBMU_ModBlkVolt_M14B06", "AEthernet.HV_Batt.TCU.RX_PDUs.BMU_MODBLKVOLT.IBMU_ModBlkVolt_M14B07", "AEthernet.HV_Batt.TCU.RX_PDUs.BMU_MODBLKVOLT.IBMU_ModBlkVolt_M14B08", "AEthernet.HV_Batt.TCU.RX_PDUs.BMU_MODBLKVOLT.IBMU_ModBlkVolt_M14B09", "AEthernet.HV_Batt.TCU.RX_PDUs.BMU_MODBLKVOLT.IBMU_ModBlkVolt_M15B00", "AEthernet.HV_Batt.TCU.RX_PDUs.BMU_MODBLKVOLT.IBMU_ModBlkVolt_M15B01", "AEthernet.HV_Batt.TCU.RX_PDUs.BMU_MODBLKVOLT.IBMU_ModBlkVolt_M15B02", "AEthernet.HV_Batt.TCU.RX_PDUs.BMU_MODBLKVOLT.IBMU_ModBlkVolt_M15B03", "AEthernet.HV_Batt.TCU.RX_PDUs.BMU_MODBLKVOLT.IBMU_ModBlkVolt_M15B04", "AEthernet.HV_Batt.TCU.RX_PDUs.BMU_MODBLKVOLT.IBMU_ModBlkVolt_M15B05", "AEthernet.HV_Batt.TCU.RX_PDUs.BMU_MODBLKVOLT.IBMU_ModBlkVolt_M15B06", "AEthernet.HV_Batt.TCU.RX_PDUs.BMU_MODBLKVOLT.IBMU_ModBlkVolt_M15B07", "AEthernet.HV_Batt.TCU.RX_PDUs.BMU_MODBLKVOLT.IBMU_ModBlkVolt_M15B08", "AEthernet.HV_Batt.TCU.RX_PDUs.BMU_MODBLKVOLT.IBMU_ModBlkVolt_M15B09", "AEthernet.HV_Batt.TCU.RX_PDUs.BMU_MODBLKVOLT.IBMU_ModBlkVolt_M16B00", "AEthernet.HV_Batt.TCU.RX_PDUs.BMU_MODBLKVOLT.IBMU_ModBlkVolt_M16B01", "AEthernet.HV_Batt.TCU.RX_PDUs.BMU_MODBLKVOLT.IBMU_ModBlkVolt_M16B02", "AEthernet.HV_Batt.TCU.RX_PDUs.BMU_MODBLKVOLT.IBMU_ModBlkVolt_M16B03", "AEthernet.HV_Batt.TCU.RX_PDUs.BMU_MODBLKVOLT.IBMU_ModBlkVolt_M16B04", "AEthernet.HV_Batt.TCU.RX_PDUs.BMU_MODBLKVOLT.IBMU_ModBlkVolt_M16B05", "AEthernet.HV_Batt.TCU.RX_PDUs.BMU_MODBLKVOLT.IBMU_ModBlkVolt_M16B06", "AEthernet.HV_Batt.TCU.RX_PDUs.BMU_MODBLKVOLT.IBMU_ModBlkVolt_M16B07", "AEthernet.HV_Batt.TCU.RX_PDUs.BMU_MODBLKVOLT.IBMU_ModBlkVolt_M16B08", "AEthernet.HV_Batt.TCU.RX_PDUs.BMU_MODBLKVOLT.IBMU_ModBlkVolt_M16B09", "AEthernet.HV_Batt.TCU.RX_PDUs.BMU_MODBLKVOLT.IBMU_ModBlkVolt_M17B00", "AEthernet.HV_Batt.TCU.RX_PDUs.BMU_MODBLKVOLT.IBMU_ModBlkVolt_M17B01", "AEthernet.HV_Batt.TCU.RX_PDUs.BMU_MODBLKVOLT.IBMU_ModBlkVolt_M17B02", "AEthernet.HV_Batt.TCU.RX_PDUs.BMU_MODBLKVOLT.IBMU_ModBlkVolt_M17B03", "AEthernet.HV_Batt.TCU.RX_PDUs.BMU_MODBLKVOLT.IBMU_ModBlkVolt_M17B04", "AEthernet.HV_Batt.TCU.RX_PDUs.BMU_MODBLKVOLT.IBMU_ModBlkVolt_M17B05", "AEthernet.HV_Batt.TCU.RX_PDUs.BMU_MODBLKVOLT.IBMU_ModBlkVolt_M17B06", "AEthernet.HV_Batt.TCU.RX_PDUs.BMU_MODBLKVOLT.IBMU_ModBlkVolt_M17B07", "AEthernet.HV_Batt.TCU.RX_PDUs.BMU_MODBLKVOLT.IBMU_ModBlkVolt_M17B08", "AEthernet.HV_Batt.TCU.RX_PDUs.BMU_MODBLKVOLT.IBMU_ModBlkVolt_M17B09", "AEthernet.HV_Batt.TCU.RX_PDUs.BMU_MODBLKVOLT.IBMU_ModBlkVolt_M18B00", "AEthernet.HV_Batt.TCU.RX_PDUs.BMU_MODBLKVOLT.IBMU_ModBlkVolt_M18B01", "AEthernet.HV_Batt.TCU.RX_PDUs.BMU_MODBLKVOLT.IBMU_ModBlkVolt_M18B02", "AEthernet.HV_Batt.TCU.RX_PDUs.BMU_MODBLKVOLT.IBMU_ModBlkVolt_M18B03", "AEthernet.HV_Batt.TCU.RX_PDUs.BMU_MODBLKVOLT.IBMU_ModBlkVolt_M18B04", "AEthernet.HV_Batt.TCU.RX_PDUs.BMU_MODBLKVOLT.IBMU_ModBlkVolt_M18B05", "AEthernet.HV_Batt.TCU.RX_PDUs.BMU_MODBLKVOLT.IBMU_ModBlkVolt_M18B06", "AEthernet.HV_Batt.TCU.RX_PDUs.BMU_MODBLKVOLT.IBMU_ModBlkVolt_M18B07", "AEthernet.HV_Batt.TCU.RX_PDUs.BMU_MODBLKVOLT.IBMU_ModBlkVolt_M18B08", "AEthernet.HV_Batt.TCU.RX_PDUs.BMU_MODBLKVOLT.IBMU_ModBlkVolt_M18B09", "AEthernet.HV_Batt.TCU.RX_PDUs.BMU_MODBLKVOLT.IBMU_ModBlkVolt_M19B00", "AEthernet.HV_Batt.TCU.RX_PDUs.BMU_MODBLKVOLT.IBMU_ModBlkVolt_M19B01", "AEthernet.HV_Batt.TCU.RX_PDUs.BMU_MODBLKVOLT.IBMU_ModBlkVolt_M19B02", "AEthernet.HV_Batt.TCU.RX_PDUs.BMU_MODBLKVOLT.IBMU_ModBlkVolt_M19B03", "AEthernet.HV_Batt.TCU.RX_PDUs.BMU_MODBLKVOLT.IBMU_ModBlkVolt_M19B04", "AEthernet.HV_Batt.TCU.RX_PDUs.BMU_MODBLKVOLT.IBMU_ModBlkVolt_M19B05", "AEthernet.HV_Batt.TCU.RX_PDUs.BMU_MODBLKVOLT.IBMU_ModBlkVolt_M19B06", "AEthernet.HV_Batt.TCU.RX_PDUs.BMU_MODBLKVOLT.IBMU_ModBlkVolt_M19B07", "AEthernet.HV_Batt.TCU.RX_PDUs.BMU_MODBLKVOLT.IBMU_ModBlkVolt_M19B08", "AEthernet.HV_Batt.TCU.RX_PDUs.BMU_MODBLKVOLT.IBMU_ModBlkVolt_M19B09", "AEthernet.HV_Batt.TCU.RX_PDUs.BMU_MODBLKVOLT.IBMU_ModBlkVolt_M20B00", "AEthernet.HV_Batt.TCU.RX_PDUs.BMU_MODBLKVOLT.IBMU_ModBlkVolt_M20B01", "AEthernet.HV_Batt.TCU.RX_PDUs.BMU_MODBLKVOLT.IBMU_ModBlkVolt_M20B02", "AEthernet.HV_Batt.TCU.RX_PDUs.BMU_MODBLKVOLT.IBMU_ModBlkVolt_M20B03", "AEthernet.HV_Batt.TCU.RX_PDUs.BMU_MODBLKVOLT.IBMU_ModBlkVolt_M20B04", "AEthernet.HV_Batt.TCU.RX_PDUs.BMU_MODBLKVOLT.IBMU_ModBlkVolt_M20B05", "AEthernet.HV_Batt.TCU.RX_PDUs.BMU_MODBLKVOLT.IBMU_ModBlkVolt_M20B06", "AEthernet.HV_Batt.TCU.RX_PDUs.BMU_MODBLKVOLT.IBMU_ModBlkVolt_M20B07", "AEthernet.HV_Batt.TCU.RX_PDUs.BMU_MODBLKVOLT.IBMU_ModBlkVolt_M20B08", "AEthernet.HV_Batt.TCU.RX_PDUs.BMU_MODBLKVOLT.IBMU_ModBlkVolt_M20B09", "AEthernet.HV_Batt.TCU.RX_PDUs.BMU_MODBLKVOLT.IBMU_ModBlkVolt_M21B00", "AEthernet.HV_Batt.TCU.RX_PDUs.BMU_MODBLKVOLT.IBMU_ModBlkVolt_M21B01", "AEthernet.HV_Batt.TCU.RX_PDUs.BMU_MODBLKVOLT.IBMU_ModBlkVolt_M21B02", "AEthernet.HV_Batt.TCU.RX_PDUs.BMU_MODBLKVOLT.IBMU_ModBlkVolt_M21B03", "AEthernet.HV_Batt.TCU.RX_PDUs.BMU_MODBLKVOLT.IBMU_ModBlkVolt_M21B04", "AEthernet.HV_Batt.TCU.RX_PDUs.BMU_MODBLKVOLT.IBMU_ModBlkVolt_M21B05", "AEthernet.HV_Batt.TCU.RX_PDUs.BMU_MODBLKVOLT.IBMU_ModBlkVolt_M21B06", "AEthernet.HV_Batt.TCU.RX_PDUs.BMU_MODBLKVOLT.IBMU_ModBlkVolt_M21B07", "AEthernet.HV_Batt.TCU.RX_PDUs.BMU_MODBLKVOLT.IBMU_ModBlkVolt_M21B08", "AEthernet.HV_Batt.TCU.RX_PDUs.BMU_MODBLKVOLT.IBMU_ModBlkVolt_M21B09", "AEthernet.HV_Batt.TCU.RX_PDUs.BMU_MODBLKVOLT.IBMU_ModBlkVolt_M22B00", "AEthernet.HV_Batt.TCU.RX_PDUs.BMU_MODBLKVOLT.IBMU_ModBlkVolt_M22B01", "AEthernet.HV_Batt.TCU.RX_PDUs.BMU_MODBLKVOLT.IBMU_ModBlkVolt_M22B02", "AEthernet.HV_Batt.TCU.RX_PDUs.BMU_MODBLKVOLT.IBMU_ModBlkVolt_M22B03", "AEthernet.HV_Batt.TCU.RX_PDUs.BMU_MODBLKVOLT.IBMU_ModBlkVolt_M22B04", "AEthernet.HV_Batt.TCU.RX_PDUs.BMU_MODBLKVOLT.IBMU_ModBlkVolt_M22B05", "AEthernet.HV_Batt.TCU.RX_PDUs.BMU_MODBLKVOLT.IBMU_ModBlkVolt_M22B06", "AEthernet.HV_Batt.TCU.RX_PDUs.BMU_MODBLKVOLT.IBMU_ModBlkVolt_M22B07", "AEthernet.HV_Batt.TCU.RX_PDUs.BMU_MODBLKVOLT.IBMU_ModBlkVolt_M22B08", "AEthernet.HV_Batt.TCU.RX_PDUs.BMU_MODBLKVOLT.IBMU_ModBlkVolt_M22B09", "AEthernet.HV_Batt.TCU.RX_PDUs.BMU_MODBLKVOLT.IBMU_ModBlkVolt_M23B00", "AEthernet.HV_Batt.TCU.RX_PDUs.BMU_MODBLKVOLT.IBMU_ModBlkVolt_M23B01", "AEthernet.HV_Batt.TCU.RX_PDUs.BMU_MODBLKVOLT.IBMU_ModBlkVolt_M23B02", "AEthernet.HV_Batt.TCU.RX_PDUs.BMU_MODBLKVOLT.IBMU_ModBlkVolt_M23B03", "AEthernet.HV_Batt.TCU.RX_PDUs.BMU_MODBLKVOLT.IBMU_ModBlkVolt_M23B04", "AEthernet.HV_Batt.TCU.RX_PDUs.BMU_MODBLKVOLT.IBMU_ModBlkVolt_M23B05", "AEthernet.HV_Batt.TCU.RX_PDUs.BMU_MODBLKVOLT.IBMU_ModBlkVolt_M23B06", "AEthernet.HV_Batt.TCU.RX_PDUs.BMU_MODBLKVOLT.IBMU_ModBlkVolt_M23B07", "AEthernet.HV_Batt.TCU.RX_PDUs.BMU_MODBLKVOLT.IBMU_ModBlkVolt_M23B08", "AEthernet.HV_Batt.TCU.RX_PDUs.BMU_MODBLKVOLT.IBMU_ModBlkVolt_M23B09", "AEthernet.HV_Batt.TCU.RX_PDUs.BMU_MODBLKVOLT.IBMU_ModBlkVolt_M24B00", "AEthernet.HV_Batt.TCU.RX_PDUs.BMU_MODBLKVOLT.IBMU_ModBlkVolt_M24B01", "AEthernet.HV_Batt.TCU.RX_PDUs.BMU_MODBLKVOLT.IBMU_ModBlkVolt_M24B02", "AEthernet.HV_Batt.TCU.RX_PDUs.BMU_MODBLKVOLT.IBMU_ModBlkVolt_M24B03", "AEthernet.HV_Batt.TCU.RX_PDUs.BMU_MODBLKVOLT.IBMU_ModBlkVolt_M24B04", "AEthernet.HV_Batt.TCU.RX_PDUs.BMU_MODBLKVOLT.IBMU_ModBlkVolt_M24B05", "AEthernet.HV_Batt.TCU.RX_PDUs.BMU_MODBLKVOLT.IBMU_ModBlkVolt_M24B06", "AEthernet.HV_Batt.TCU.RX_PDUs.BMU_MODBLKVOLT.IBMU_ModBlkVolt_M24B07", "AEthernet.HV_Batt.TCU.RX_PDUs.BMU_MODBLKVOLT.IBMU_ModBlkVolt_M24B08", "AEthernet.HV_Batt.TCU.RX_PDUs.BMU_MODBLKVOLT.IBMU_ModBlkVolt_M24B09", "AEthernet.HV_Batt.TCU.RX_PDUs.BMU_MODBLKVOLT.IBMU_ModBlkVolt_M25B00", "AEthernet.HV_Batt.TCU.RX_PDUs.BMU_MODBLKVOLT.IBMU_ModBlkVolt_M25B01", "AEthernet.HV_Batt.TCU.RX_PDUs.BMU_MODBLKVOLT.IBMU_ModBlkVolt_M25B02", "AEthernet.HV_Batt.TCU.RX_PDUs.BMU_MODBLKVOLT.IBMU_ModBlkVolt_M25B03", "AEthernet.HV_Batt.TCU.RX_PDUs.BMU_MODBLKVOLT.IBMU_ModBlkVolt_M25B04", "AEthernet.HV_Batt.TCU.RX_PDUs.BMU_MODBLKVOLT.IBMU_ModBlkVolt_M25B05", "AEthernet.HV_Batt.TCU.RX_PDUs.BMU_MODBLKVOLT.IBMU_ModBlkVolt_M25B06", "AEthernet.HV_Batt.TCU.RX_PDUs.BMU_MODBLKVOLT.IBMU_ModBlkVolt_M25B07", "AEthernet.HV_Batt.TCU.RX_PDUs.BMU_MODBLKVOLT.IBMU_ModBlkVolt_M25B08", "AEthernet.HV_Batt.TCU.RX_PDUs.BMU_MODBLKVOLT.IBMU_ModBlkVolt_M25B09", "AEthernet.HV_Batt.TCU.RX_PDUs.BMU_MODBLKVOLT.IBMU_ModBlkVolt_M26B00", "AEthernet.HV_Batt.TCU.RX_PDUs.BMU_MODBLKVOLT.IBMU_ModBlkVolt_M26B01", "AEthernet.HV_Batt.TCU.RX_PDUs.BMU_MODBLKVOLT.IBMU_ModBlkVolt_M26B02", "AEthernet.HV_Batt.TCU.RX_PDUs.BMU_MODBLKVOLT.IBMU_ModBlkVolt_M26B03", "AEthernet.HV_Batt.TCU.RX_PDUs.BMU_MODBLKVOLT.IBMU_ModBlkVolt_M26B04", "AEthernet.HV_Batt.TCU.RX_PDUs.BMU_MODBLKVOLT.IBMU_ModBlkVolt_M26B05", "AEthernet.HV_Batt.TCU.RX_PDUs.BMU_MODBLKVOLT.IBMU_ModBlkVolt_M26B06", "AEthernet.HV_Batt.TCU.RX_PDUs.BMU_MODBLKVOLT.IBMU_ModBlkVolt_M26B07", "AEthernet.HV_Batt.TCU.RX_PDUs.BMU_MODBLKVOLT.IBMU_ModBlkVolt_M26B08", "AEthernet.HV_Batt.TCU.RX_PDUs.BMU_MODBLKVOLT.IBMU_ModBlkVolt_M26B09", "AEthernet.HV_Batt.TCU.RX_PDUs.BMU_MODBLKVOLT.IBMU_ModBlkVolt_M27B00", "AEthernet.HV_Batt.TCU.RX_PDUs.BMU_MODBLKVOLT.IBMU_ModBlkVolt_M27B01", "AEthernet.HV_Batt.TCU.RX_PDUs.BMU_MODBLKVOLT.IBMU_ModBlkVolt_M27B02", "AEthernet.HV_Batt.TCU.RX_PDUs.BMU_MODBLKVOLT.IBMU_ModBlkVolt_M27B03", "AEthernet.HV_Batt.TCU.RX_PDUs.BMU_MODBLKVOLT.IBMU_ModBlkVolt_M27B04", "AEthernet.HV_Batt.TCU.RX_PDUs.BMU_MODBLKVOLT.IBMU_ModBlkVolt_M27B05", "AEthernet.HV_Batt.TCU.RX_PDUs.BMU_MODBLKVOLT.IBMU_ModBlkVolt_M27B06", "AEthernet.HV_Batt.TCU.RX_PDUs.BMU_MODBLKVOLT.IBMU_ModBlkVolt_M27B07", "AEthernet.HV_Batt.TCU.RX_PDUs.BMU_MODBLKVOLT.IBMU_ModBlkVolt_M27B08", "AEthernet.HV_Batt.TCU.RX_PDUs.BMU_MODBLKVOLT.IBMU_ModBlkVolt_M27B09", "AEthernet.HV_Batt.TCU.RX_PDUs.BMU_MODBLKVOLT.IBMU_ModBlkVolt_M28B00", "AEthernet.HV_Batt.TCU.RX_PDUs.BMU_MODBLKVOLT.IBMU_ModBlkVolt_M28B01", "AEthernet.HV_Batt.TCU.RX_PDUs.BMU_MODBLKVOLT.IBMU_ModBlkVolt_M28B02", "AEthernet.HV_Batt.TCU.RX_PDUs.BMU_MODBLKVOLT.IBMU_ModBlkVolt_M28B03", "AEthernet.HV_Batt.TCU.RX_PDUs.BMU_MODBLKVOLT.IBMU_ModBlkVolt_M28B04", "AEthernet.HV_Batt.TCU.RX_PDUs.BMU_MODBLKVOLT.IBMU_ModBlkVolt_M28B05", "AEthernet.HV_Batt.TCU.RX_PDUs.BMU_MODBLKVOLT.IBMU_ModBlkVolt_M28B06", "AEthernet.HV_Batt.TCU.RX_PDUs.BMU_MODBLKVOLT.IBMU_ModBlkVolt_M28B07", "AEthernet.HV_Batt.TCU.RX_PDUs.BMU_MODBLKVOLT.IBMU_ModBlkVolt_M28B08", "AEthernet.HV_Batt.TCU.RX_PDUs.BMU_MODBLKVOLT.IBMU_ModBlkVolt_M28B09", "AEthernet.HV_Batt.TCU.RX_PDUs.BMU_MODBLKVOLT.IBMU_ModBlkVolt_M29B00", "AEthernet.HV_Batt.TCU.RX_PDUs.BMU_MODBLKVOLT.IBMU_ModBlkVolt_M29B01", "AEthernet.HV_Batt.TCU.RX_PDUs.BMU_MODBLKVOLT.IBMU_ModBlkVolt_M29B02", "AEthernet.HV_Batt.TCU.RX_PDUs.BMU_MODBLKVOLT.IBMU_ModBlkVolt_M29B03", "AEthernet.HV_Batt.TCU.RX_PDUs.BMU_MODBLKVOLT.IBMU_ModBlkVolt_M29B04", "AEthernet.HV_Batt.TCU.RX_PDUs.BMU_MODBLKVOLT.IBMU_ModBlkVolt_M29B05", "AEthernet.HV_Batt.TCU.RX_PDUs.BMU_MODBLKVOLT.IBMU_ModBlkVolt_M29B06", "AEthernet.HV_Batt.TCU.RX_PDUs.BMU_MODBLKVOLT.IBMU_ModBlkVolt_M29B07", "AEthernet.HV_Batt.TCU.RX_PDUs.BMU_MODBLKVOLT.IBMU_ModBlkVolt_M29B08", "AEthernet.HV_Batt.TCU.RX_PDUs.BMU_MODBLKVOLT.IBMU_ModBlkVolt_M29B09", "AEthernet.HV_Batt.TCU.RX_PDUs.BMU_MODBLKVOLT.IBMU_ModBlkVolt_M30B00", "AEthernet.HV_Batt.TCU.RX_PDUs.BMU_MODBLKVOLT.IBMU_ModBlkVolt_M30B01", "AEthernet.HV_Batt.TCU.RX_PDUs.BMU_MODBLKVOLT.IBMU_ModBlkVolt_M30B02", "AEthernet.HV_Batt.TCU.RX_PDUs.BMU_MODBLKVOLT.IBMU_ModBlkVolt_M30B03", "AEthernet.HV_Batt.TCU.RX_PDUs.BMU_MODBLKVOLT.IBMU_ModBlkVolt_M30B04", "AEthernet.HV_Batt.TCU.RX_PDUs.BMU_MODBLKVOLT.IBMU_ModBlkVolt_M30B05", "AEthernet.HV_Batt.TCU.RX_PDUs.BMU_MODBLKVOLT.IBMU_ModBlkVolt_M30B06", "AEthernet.HV_Batt.TCU.RX_PDUs.BMU_MODBLKVOLT.IBMU_ModBlkVolt_M30B07", "AEthernet.HV_Batt.TCU.RX_PDUs.BMU_MODBLKVOLT.IBMU_ModBlkVolt_M30B08", "AEthernet.HV_Batt.TCU.RX_PDUs.BMU_MODBLKVOLT.IBMU_ModBlkVolt_M30B09", "AEthernet.HV_Batt.TCU.RX_PDUs.BMU_MODBLKVOLT.IBMU_ModBlkVolt_M31B00", "AEthernet.HV_Batt.TCU.RX_PDUs.BMU_MODBLKVOLT.IBMU_ModBlkVolt_M31B01", "AEthernet.HV_Batt.TCU.RX_PDUs.BMU_MODBLKVOLT.IBMU_ModBlkVolt_M31B02", "AEthernet.HV_Batt.TCU.RX_PDUs.BMU_MODBLKVOLT.IBMU_ModBlkVolt_M31B03", "AEthernet.HV_Batt.TCU.RX_PDUs.BMU_MODBLKVOLT.IBMU_ModBlkVolt_M31B04", "AEthernet.HV_Batt.TCU.RX_PDUs.BMU_MODBLKVOLT.IBMU_ModBlkVolt_M31B05", "AEthernet.HV_Batt.TCU.RX_PDUs.BMU_MODBLKVOLT.IBMU_ModBlkVolt_M31B06", "AEthernet.HV_Batt.TCU.RX_PDUs.BMU_MODBLKVOLT.IBMU_ModBlkVolt_M31B07", "AEthernet.HV_Batt.TCU.RX_PDUs.BMU_MODBLKVOLT.IBMU_ModBlkVolt_M31B08", "AEthernet.HV_Batt.TCU.RX_PDUs.BMU_MODBLKVOLT.IBMU_ModBlkVolt_M31B09", "AEthernet.HV_Batt.TCU.RX_PDUs.BMU_MODBLKVOLT.IBMU_ModBlkVolt_M32B00", "AEthernet.HV_Batt.TCU.RX_PDUs.BMU_MODBLKVOLT.IBMU_ModBlkVolt_M32B01", "AEthernet.HV_Batt.TCU.RX_PDUs.BMU_MODBLKVOLT.IBMU_ModBlkVolt_M32B02", "AEthernet.HV_Batt.TCU.RX_PDUs.BMU_MODBLKVOLT.IBMU_ModBlkVolt_M32B03", "AEthernet.HV_Batt.TCU.RX_PDUs.BMU_MODBLKVOLT.IBMU_ModBlkVolt_M32B04", "AEthernet.HV_Batt.TCU.RX_PDUs.BMU_MODBLKVOLT.IBMU_ModBlkVolt_M32B05", "AEthernet.HV_Batt.TCU.RX_PDUs.BMU_MODBLKVOLT.IBMU_ModBlkVolt_M32B06", "AEthernet.HV_Batt.TCU.RX_PDUs.BMU_MODBLKVOLT.IBMU_ModBlkVolt_M32B07", "AEthernet.HV_Batt.TCU.RX_PDUs.BMU_MODBLKVOLT.IBMU_ModBlkVolt_M32B08", "AEthernet.HV_Batt.TCU.RX_PDUs.BMU_MODBLKVOLT.IBMU_ModBlkVolt_M32B09", "AEthernet.HV_Batt.TCU.RX_PDUs.BMU_MODBLKVOLT.IBMU_ModBlkVolt_M33B00", "AEthernet.HV_Batt.TCU.RX_PDUs.BMU_MODBLKVOLT.IBMU_ModBlkVolt_M33B01", "AEthernet.HV_Batt.TCU.RX_PDUs.BMU_MODBLKVOLT.IBMU_ModBlkVolt_M33B02", "AEthernet.HV_Batt.TCU.RX_PDUs.BMU_MODBLKVOLT.IBMU_ModBlkVolt_M33B03", "AEthernet.HV_Batt.TCU.RX_PDUs.BMU_MODBLKVOLT.IBMU_ModBlkVolt_M33B04", "AEthernet.HV_Batt.TCU.RX_PDUs.BMU_MODBLKVOLT.IBMU_ModBlkVolt_M33B05", "AEthernet.HV_Batt.TCU.RX_PDUs.BMU_MODBLKVOLT.IBMU_ModBlkVolt_M33B06", "AEthernet.HV_Batt.TCU.RX_PDUs.BMU_MODBLKVOLT.IBMU_ModBlkVolt_M33B07", "AEthernet.HV_Batt.TCU.RX_PDUs.BMU_MODBLKVOLT.IBMU_ModBlkVolt_M33B08", "AEthernet.HV_Batt.TCU.RX_PDUs.BMU_MODBLKVOLT.IBMU_ModBlkVolt_M33B09", "AEthernet.HV_Batt.TCU.RX_PDUs.BMU_MODBLKVOLT.IBMU_ModBlkVolt_M34B00", "AEthernet.HV_Batt.TCU.RX_PDUs.BMU_MODBLKVOLT.IBMU_ModBlkVolt_M34B01", "AEthernet.HV_Batt.TCU.RX_PDUs.BMU_MODBLKVOLT.IBMU_ModBlkVolt_M34B02", "AEthernet.HV_Batt.TCU.RX_PDUs.BMU_MODBLKVOLT.IBMU_ModBlkVolt_M34B03", "AEthernet.HV_Batt.TCU.RX_PDUs.BMU_MODBLKVOLT.IBMU_ModBlkVolt_M34B04", "AEthernet.HV_Batt.TCU.RX_PDUs.BMU_MODBLKVOLT.IBMU_ModBlkVolt_M34B05", "AEthernet.HV_Batt.TCU.RX_PDUs.BMU_MODBLKVOLT.IBMU_ModBlkVolt_M34B06", "AEthernet.HV_Batt.TCU.RX_PDUs.BMU_MODBLKVOLT.IBMU_ModBlkVolt_M34B07", "AEthernet.HV_Batt.TCU.RX_PDUs.BMU_MODBLKVOLT.IBMU_ModBlkVolt_M34B08", "AEthernet.HV_Batt.TCU.RX_PDUs.BMU_MODBLKVOLT.IBMU_ModBlkVolt_M34B09", "AEthernet.HV_Batt.TCU.RX_PDUs.BMU_MODBLKVOLT.IBMU_ModBlkVolt_M35B00", "AEthernet.HV_Batt.TCU.RX_PDUs.BMU_MODBLKVOLT.IBMU_ModBlkVolt_M35B01", "AEthernet.HV_Batt.TCU.RX_PDUs.BMU_MODBLKVOLT.IBMU_ModBlkVolt_M35B02", "AEthernet.HV_Batt.TCU.RX_PDUs.BMU_MODBLKVOLT.IBMU_ModBlkVolt_M35B03", "AEthernet.HV_Batt.TCU.RX_PDUs.BMU_MODBLKVOLT.IBMU_ModBlkVolt_M35B04", "AEthernet.HV_Batt.TCU.RX_PDUs.BMU_MODBLKVOLT.IBMU_ModBlkVolt_M35B05", "AEthernet.HV_Batt.TCU.RX_PDUs.BMU_MODBLKVOLT.IBMU_ModBlkVolt_M35B06", "AEthernet.HV_Batt.TCU.RX_PDUs.BMU_MODBLKVOLT.IBMU_ModBlkVolt_M35B07", "AEthernet.HV_Batt.TCU.RX_PDUs.BMU_MODBLKVOLT.IBMU_ModBlkVolt_M35B08", "AEthernet.HV_Batt.TCU.RX_PDUs.BMU_MODBLKVOLT.IBMU_ModBlkVolt_M35B09", "AEthernet.HV_Batt.TCU.RX_PDUs.BMU_MODBLKVOLT.IBMU_ModBlkVolt_M36B00", "AEthernet.HV_Batt.TCU.RX_PDUs.BMU_MODBLKVOLT.IBMU_ModBlkVolt_M36B01", "AEthernet.HV_Batt.TCU.RX_PDUs.BMU_MODBLKVOLT.IBMU_ModBlkVolt_M36B02", "AEthernet.HV_Batt.TCU.RX_PDUs.BMU_MODBLKVOLT.IBMU_ModBlkVolt_M36B03", "AEthernet.HV_Batt.TCU.RX_PDUs.BMU_MODBLKVOLT.IBMU_ModBlkVolt_M36B04", "AEthernet.HV_Batt.TCU.RX_PDUs.BMU_MODBLKVOLT.IBMU_ModBlkVolt_M36B05", "AEthernet.HV_Batt.TCU.RX_PDUs.BMU_MODBLKVOLT.IBMU_ModBlkVolt_M36B06", "AEthernet.HV_Batt.TCU.RX_PDUs.BMU_MODBLKVOLT.IBMU_ModBlkVolt_M36B07", "AEthernet.HV_Batt.TCU.RX_PDUs.BMU_MODBLKVOLT.IBMU_ModBlkVolt_M36B08", "AEthernet.HV_Batt.TCU.RX_PDUs.BMU_MODBLKVOLT.IBMU_ModBlkVolt_M36B09", "AEthernet.HV_Batt.TCU.RX_PDUs.BMU_MODBLKVOLT.IBMU_ModBlkVolt_M37B00", "AEthernet.HV_Batt.TCU.RX_PDUs.BMU_MODBLKVOLT.IBMU_ModBlkVolt_M37B01", "AEthernet.HV_Batt.TCU.RX_PDUs.BMU_MODBLKVOLT.IBMU_ModBlkVolt_M37B02", "AEthernet.HV_Batt.TCU.RX_PDUs.BMU_MODBLKVOLT.IBMU_ModBlkVolt_M37B03", "AEthernet.HV_Batt.TCU.RX_PDUs.BMU_MODBLKVOLT.IBMU_ModBlkVolt_M37B04", "AEthernet.HV_Batt.TCU.RX_PDUs.BMU_MODBLKVOLT.IBMU_ModBlkVolt_M37B05", "AEthernet.HV_Batt.TCU.RX_PDUs.BMU_MODBLKVOLT.IBMU_ModBlkVolt_M37B06", "AEthernet.HV_Batt.TCU.RX_PDUs.BMU_MODBLKVOLT.IBMU_ModBlkVolt_M37B07", "AEthernet.HV_Batt.TCU.RX_PDUs.BMU_MODBLKVOLT.IBMU_ModBlkVolt_M37B08", "AEthernet.HV_Batt.TCU.RX_PDUs.BMU_MODBLKVOLT.IBMU_ModBlkVolt_M37B09", "AEthernet.HV_Batt.TCU.RX_PDUs.BMU_MODBLKVOLT.IBMU_ModBlkVolt_M38B00", "AEthernet.HV_Batt.TCU.RX_PDUs.BMU_MODBLKVOLT.IBMU_ModBlkVolt_M38B01", "AEthernet.HV_Batt.TCU.RX_PDUs.BMU_MODBLKVOLT.IBMU_ModBlkVolt_M38B02", "AEthernet.HV_Batt.TCU.RX_PDUs.BMU_MODBLKVOLT.IBMU_ModBlkVolt_M38B03", "AEthernet.HV_Batt.TCU.RX_PDUs.BMU_MODBLKVOLT.IBMU_ModBlkVolt_M38B04", "AEthernet.HV_Batt.TCU.RX_PDUs.BMU_MODBLKVOLT.IBMU_ModBlkVolt_M38B05", "AEthernet.HV_Batt.TCU.RX_PDUs.BMU_MODBLKVOLT.IBMU_ModBlkVolt_M38B06", "AEthernet.HV_Batt.TCU.RX_PDUs.BMU_MODBLKVOLT.IBMU_ModBlkVolt_M38B07", "AEthernet.HV_Batt.TCU.RX_PDUs.BMU_MODBLKVOLT.IBMU_ModBlkVolt_M38B08", "AEthernet.HV_Batt.TCU.RX_PDUs.BMU_MODBLKVOLT.IBMU_ModBlkVolt_M38B09", "AEthernet.HV_Batt.TCU.RX_PDUs.BMU_MODBLKVOLT.IBMU_ModBlkVolt_M39B00", "AEthernet.HV_Batt.TCU.RX_PDUs.BMU_MODBLKVOLT.IBMU_ModBlkVolt_M39B01", "AEthernet.HV_Batt.TCU.RX_PDUs.BMU_MODBLKVOLT.IBMU_ModBlkVolt_M39B02", "AEthernet.HV_Batt.TCU.RX_PDUs.BMU_MODBLKVOLT.IBMU_ModBlkVolt_M39B03", "AEthernet.HV_Batt.TCU.RX_PDUs.BMU_MODBLKVOLT.IBMU_ModBlkVolt_M39B04", "AEthernet.HV_Batt.TCU.RX_PDUs.BMU_MODBLKVOLT.IBMU_ModBlkVolt_M39B05", "AEthernet.HV_Batt.TCU.RX_PDUs.BMU_MODBLKVOLT.IBMU_ModBlkVolt_M39B06", "AEthernet.HV_Batt.TCU.RX_PDUs.BMU_MODBLKVOLT.IBMU_ModBlkVolt_M39B07", "AEthernet.HV_Batt.TCU.RX_PDUs.BMU_MODBLKVOLT.IBMU_ModBlkVolt_M39B08", "AEthernet.HV_Batt.TCU.RX_PDUs.BMU_MODBLKVOLT.IBMU_ModBlkVolt_M39B09", "AEthernet.HV_Batt.TCU.RX_PDUs.BMU_MODBLKVOLT.IBMU_ModBlkVolt_M40B00", "AEthernet.HV_Batt.TCU.RX_PDUs.BMU_MODBLKVOLT.IBMU_ModBlkVolt_M40B01", "AEthernet.HV_Batt.TCU.RX_PDUs.BMU_MODBLKVOLT.IBMU_ModBlkVolt_M40B02", "AEthernet.HV_Batt.TCU.RX_PDUs.BMU_MODBLKVOLT.IBMU_ModBlkVolt_M40B03", "AEthernet.HV_Batt.TCU.RX_PDUs.BMU_MODBLKVOLT.IBMU_ModBlkVolt_M40B04", "AEthernet.HV_Batt.TCU.RX_PDUs.BMU_MODBLKVOLT.IBMU_ModBlkVolt_M40B05", "AEthernet.HV_Batt.TCU.RX_PDUs.BMU_MODBLKVOLT.IBMU_ModBlkVolt_M40B06", "AEthernet.HV_Batt.TCU.RX_PDUs.BMU_MODBLKVOLT.IBMU_ModBlkVolt_M40B07", "AEthernet.HV_Batt.TCU.RX_PDUs.BMU_MODBLKVOLT.IBMU_ModBlkVolt_M40B08", "AEthernet.HV_Batt.TCU.RX_PDUs.BMU_MODBLKVOLT.IBMU_ModBlkVolt_M40B09", "AEthernet.HV_Batt.TCU.RX_PDUs.BMU_MODBLKVOLT.IBMU_ModBlkVolt_M41B00", "AEthernet.HV_Batt.TCU.RX_PDUs.BMU_MODBLKVOLT.IBMU_ModBlkVolt_M41B01", "AEthernet.HV_Batt.TCU.RX_PDUs.BMU_MODBLKVOLT.IBMU_ModBlkVolt_M41B02", "AEthernet.HV_Batt.TCU.RX_PDUs.BMU_MODBLKVOLT.IBMU_ModBlkVolt_M41B03", "AEthernet.HV_Batt.TCU.RX_PDUs.BMU_MODBLKVOLT.IBMU_ModBlkVolt_M41B04", "AEthernet.HV_Batt.TCU.RX_PDUs.BMU_MODBLKVOLT.IBMU_ModBlkVolt_M41B05", "AEthernet.HV_Batt.TCU.RX_PDUs.BMU_MODBLKVOLT.IBMU_ModBlkVolt_M41B06", "AEthernet.HV_Batt.TCU.RX_PDUs.BMU_MODBLKVOLT.IBMU_ModBlkVolt_M41B07", "AEthernet.HV_Batt.TCU.RX_PDUs.BMU_MODBLKVOLT.IBMU_ModBlkVolt_M41B08", "AEthernet.HV_Batt.TCU.RX_PDUs.BMU_MODBLKVOLT.IBMU_ModBlkVolt_M41B09", "AEthernet.HV_Batt.TCU.RX_PDUs.BMU_MODBLKVOLT.IBMU_ModBlkVolt_M42B00", "AEthernet.HV_Batt.TCU.RX_PDUs.BMU_MODBLKVOLT.IBMU_ModBlkVolt_M42B01", "AEthernet.HV_Batt.TCU.RX_PDUs.BMU_MODBLKVOLT.IBMU_ModBlkVolt_M42B02", "AEthernet.HV_Batt.TCU.RX_PDUs.BMU_MODBLKVOLT.IBMU_ModBlkVolt_M42B03", "AEthernet.HV_Batt.TCU.RX_PDUs.BMU_MODBLKVOLT.IBMU_ModBlkVolt_M42B04", "AEthernet.HV_Batt.TCU.RX_PDUs.BMU_MODBLKVOLT.IBMU_ModBlkVolt_M42B05", "AEthernet.HV_Batt.TCU.RX_PDUs.BMU_MODBLKVOLT.IBMU_ModBlkVolt_M42B06", "AEthernet.HV_Batt.TCU.RX_PDUs.BMU_MODBLKVOLT.IBMU_ModBlkVolt_M42B07", "AEthernet.HV_Batt.TCU.RX_PDUs.BMU_MODBLKVOLT.IBMU_ModBlkVolt_M42B08", "AEthernet.HV_Batt.TCU.RX_PDUs.BMU_MODBLKVOLT.IBMU_ModBlkVolt_M42B09", "AEthernet.HV_Batt.TCU.RX_PDUs.BMU_MODBLKVOLT.IBMU_ModBlkVolt_M43B00", "AEthernet.HV_Batt.TCU.RX_PDUs.BMU_MODBLKVOLT.IBMU_ModBlkVolt_M43B01", "AEthernet.HV_Batt.TCU.RX_PDUs.BMU_MODBLKVOLT.IBMU_ModBlkVolt_M43B02", "AEthernet.HV_Batt.TCU.RX_PDUs.BMU_MODBLKVOLT.IBMU_ModBlkVolt_M43B03", "AEthernet.HV_Batt.TCU.RX_PDUs.BMU_MODBLKVOLT.IBMU_ModBlkVolt_M43B04", "AEthernet.HV_Batt.TCU.RX_PDUs.BMU_MODBLKVOLT.IBMU_ModBlkVolt_M43B05", "AEthernet.HV_Batt.TCU.RX_PDUs.BMU_MODBLKVOLT.IBMU_ModBlkVolt_M43B06", "AEthernet.HV_Batt.TCU.RX_PDUs.BMU_MODBLKVOLT.IBMU_ModBlkVolt_M43B07", "AEthernet.HV_Batt.TCU.RX_PDUs.BMU_MODBLKVOLT.IBMU_ModBlkVolt_M43B08", "AEthernet.HV_Batt.TCU.RX_PDUs.BMU_MODBLKVOLT.IBMU_ModBlkVolt_M43B09", "AEthernet.HV_Batt.TCU.RX_PDUs.BMU_MODBLKVOLT.RX_deltatime", "AEthernet.HV_Batt.TCU.RX_PDUs.BMU_MODBLKVOLT.RX_time", "AEthernet.HV_Batt.TCU.RX_PDUs.BMU_MODCELLTEMP.IBMU_ModCellTemp_M00B00", "AEthernet.HV_Batt.TCU.RX_PDUs.BMU_MODCELLTEMP.IBMU_ModCellTemp_M00B01", "AEthernet.HV_Batt.TCU.RX_PDUs.BMU_MODCELLTEMP.IBMU_ModCellTemp_M01B00", "AEthernet.HV_Batt.TCU.RX_PDUs.BMU_MODCELLTEMP.IBMU_ModCellTemp_M01B01", "AEthernet.HV_Batt.TCU.RX_PDUs.BMU_MODCELLTEMP.IBMU_ModCellTemp_M02B00", "AEthernet.HV_Batt.TCU.RX_PDUs.BMU_MODCELLTEMP.IBMU_ModCellTemp_M02B01", "AEthernet.HV_Batt.TCU.RX_PDUs.BMU_MODCELLTEMP.IBMU_ModCellTemp_M03B00", "AEthernet.HV_Batt.TCU.RX_PDUs.BMU_MODCELLTEMP.IBMU_ModCellTemp_M03B01", "AEthernet.HV_Batt.TCU.RX_PDUs.BMU_MODCELLTEMP.IBMU_ModCellTemp_M04B00", "AEthernet.HV_Batt.TCU.RX_PDUs.BMU_MODCELLTEMP.IBMU_ModCellTemp_M04B01", "AEthernet.HV_Batt.TCU.RX_PDUs.BMU_MODCELLTEMP.IBMU_ModCellTemp_M05B00", "AEthernet.HV_Batt.TCU.RX_PDUs.BMU_MODCELLTEMP.IBMU_ModCellTemp_M05B01", "AEthernet.HV_Batt.TCU.RX_PDUs.BMU_MODCELLTEMP.IBMU_ModCellTemp_M06B00", "AEthernet.HV_Batt.TCU.RX_PDUs.BMU_MODCELLTEMP.IBMU_ModCellTemp_M06B01", "AEthernet.HV_Batt.TCU.RX_PDUs.BMU_MODCELLTEMP.IBMU_ModCellTemp_M07B00", "AEthernet.HV_Batt.TCU.RX_PDUs.BMU_MODCELLTEMP.IBMU_ModCellTemp_M07B01", "AEthernet.HV_Batt.TCU.RX_PDUs.BMU_MODCELLTEMP.IBMU_ModCellTemp_M08B00", "AEthernet.HV_Batt.TCU.RX_PDUs.BMU_MODCELLTEMP.IBMU_ModCellTemp_M08B01", "AEthernet.HV_Batt.TCU.RX_PDUs.BMU_MODCELLTEMP.IBMU_ModCellTemp_M09B00", "AEthernet.HV_Batt.TCU.RX_PDUs.BMU_MODCELLTEMP.IBMU_ModCellTemp_M09B01", "AEthernet.HV_Batt.TCU.RX_PDUs.BMU_MODCELLTEMP.IBMU_ModCellTemp_M10B00", "AEthernet.HV_Batt.TCU.RX_PDUs.BMU_MODCELLTEMP.IBMU_ModCellTemp_M10B01", "AEthernet.HV_Batt.TCU.RX_PDUs.BMU_MODCELLTEMP.IBMU_ModCellTemp_M11B00", "AEthernet.HV_Batt.TCU.RX_PDUs.BMU_MODCELLTEMP.IBMU_ModCellTemp_M11B01", "AEthernet.HV_Batt.TCU.RX_PDUs.BMU_MODCELLTEMP.IBMU_ModCellTemp_M12B00", "AEthernet.HV_Batt.TCU.RX_PDUs.BMU_MODCELLTEMP.IBMU_ModCellTemp_M12B01", "AEthernet.HV_Batt.TCU.RX_PDUs.BMU_MODCELLTEMP.IBMU_ModCellTemp_M13B00", "AEthernet.HV_Batt.TCU.RX_PDUs.BMU_MODCELLTEMP.IBMU_ModCellTemp_M13B01", "AEthernet.HV_Batt.TCU.RX_PDUs.BMU_MODCELLTEMP.IBMU_ModCellTemp_M14B00", "AEthernet.HV_Batt.TCU.RX_PDUs.BMU_MODCELLTEMP.IBMU_ModCellTemp_M14B01", "AEthernet.HV_Batt.TCU.RX_PDUs.BMU_MODCELLTEMP.IBMU_ModCellTemp_M15B00", "AEthernet.HV_Batt.TCU.RX_PDUs.BMU_MODCELLTEMP.IBMU_ModCellTemp_M15B01", "AEthernet.HV_Batt.TCU.RX_PDUs.BMU_MODCELLTEMP.IBMU_ModCellTemp_M16B00", "AEthernet.HV_Batt.TCU.RX_PDUs.BMU_MODCELLTEMP.IBMU_ModCellTemp_M16B01", "AEthernet.HV_Batt.TCU.RX_PDUs.BMU_MODCELLTEMP.IBMU_ModCellTemp_M17B00", "AEthernet.HV_Batt.TCU.RX_PDUs.BMU_MODCELLTEMP.IBMU_ModCellTemp_M17B01", "AEthernet.HV_Batt.TCU.RX_PDUs.BMU_MODCELLTEMP.IBMU_ModCellTemp_M18B00", "AEthernet.HV_Batt.TCU.RX_PDUs.BMU_MODCELLTEMP.IBMU_ModCellTemp_M18B01", "AEthernet.HV_Batt.TCU.RX_PDUs.BMU_MODCELLTEMP.IBMU_ModCellTemp_M19B00", "AEthernet.HV_Batt.TCU.RX_PDUs.BMU_MODCELLTEMP.IBMU_ModCellTemp_M19B01", "AEthernet.HV_Batt.TCU.RX_PDUs.BMU_MODCELLTEMP.IBMU_ModCellTemp_M20B00", "AEthernet.HV_Batt.TCU.RX_PDUs.BMU_MODCELLTEMP.IBMU_ModCellTemp_M20B01", "AEthernet.HV_Batt.TCU.RX_PDUs.BMU_MODCELLTEMP.IBMU_ModCellTemp_M21B00", "AEthernet.HV_Batt.TCU.RX_PDUs.BMU_MODCELLTEMP.IBMU_ModCellTemp_M21B01", "AEthernet.HV_Batt.TCU.RX_PDUs.BMU_MODCELLTEMP.IBMU_ModCellTemp_M22B00", "AEthernet.HV_Batt.TCU.RX_PDUs.BMU_MODCELLTEMP.IBMU_ModCellTemp_M22B01", "AEthernet.HV_Batt.TCU.RX_PDUs.BMU_MODCELLTEMP.IBMU_ModCellTemp_M23B00", "AEthernet.HV_Batt.TCU.RX_PDUs.BMU_MODCELLTEMP.IBMU_ModCellTemp_M23B01", "AEthernet.HV_Batt.TCU.RX_PDUs.BMU_MODCELLTEMP.IBMU_ModCellTemp_M24B00", "AEthernet.HV_Batt.TCU.RX_PDUs.BMU_MODCELLTEMP.IBMU_ModCellTemp_M24B01", "AEthernet.HV_Batt.TCU.RX_PDUs.BMU_MODCELLTEMP.IBMU_ModCellTemp_M25B00", "AEthernet.HV_Batt.TCU.RX_PDUs.BMU_MODCELLTEMP.IBMU_ModCellTemp_M25B01", "AEthernet.HV_Batt.TCU.RX_PDUs.BMU_MODCELLTEMP.IBMU_ModCellTemp_M26B00", "AEthernet.HV_Batt.TCU.RX_PDUs.BMU_MODCELLTEMP.IBMU_ModCellTemp_M26B01", "AEthernet.HV_Batt.TCU.RX_PDUs.BMU_MODCELLTEMP.IBMU_ModCellTemp_M27B00", "AEthernet.HV_Batt.TCU.RX_PDUs.BMU_MODCELLTEMP.IBMU_ModCellTemp_M27B01", "AEthernet.HV_Batt.TCU.RX_PDUs.BMU_MODCELLTEMP.IBMU_ModCellTemp_M28B00", "AEthernet.HV_Batt.TCU.RX_PDUs.BMU_MODCELLTEMP.IBMU_ModCellTemp_M28B01", "AEthernet.HV_Batt.TCU.RX_PDUs.BMU_MODCELLTEMP.IBMU_ModCellTemp_M29B00", "AEthernet.HV_Batt.TCU.RX_PDUs.BMU_MODCELLTEMP.IBMU_ModCellTemp_M29B01", "AEthernet.HV_Batt.TCU.RX_PDUs.BMU_MODCELLTEMP.IBMU_ModCellTemp_M30B00", "AEthernet.HV_Batt.TCU.RX_PDUs.BMU_MODCELLTEMP.IBMU_ModCellTemp_M30B01", "AEthernet.HV_Batt.TCU.RX_PDUs.BMU_MODCELLTEMP.IBMU_ModCellTemp_M31B00", "AEthernet.HV_Batt.TCU.RX_PDUs.BMU_MODCELLTEMP.IBMU_ModCellTemp_M31B01", "AEthernet.HV_Batt.TCU.RX_PDUs.BMU_MODCELLTEMP.IBMU_ModCellTemp_M32B00", "AEthernet.HV_Batt.TCU.RX_PDUs.BMU_MODCELLTEMP.IBMU_ModCellTemp_M32B01", "AEthernet.HV_Batt.TCU.RX_PDUs.BMU_MODCELLTEMP.IBMU_ModCellTemp_M33B00", "AEthernet.HV_Batt.TCU.RX_PDUs.BMU_MODCELLTEMP.IBMU_ModCellTemp_M33B01", "AEthernet.HV_Batt.TCU.RX_PDUs.BMU_MODCELLTEMP.IBMU_ModCellTemp_M34B00", "AEthernet.HV_Batt.TCU.RX_PDUs.BMU_MODCELLTEMP.IBMU_ModCellTemp_M34B01", "AEthernet.HV_Batt.TCU.RX_PDUs.BMU_MODCELLTEMP.IBMU_ModCellTemp_M35B00", "AEthernet.HV_Batt.TCU.RX_PDUs.BMU_MODCELLTEMP.IBMU_ModCellTemp_M35B01", "AEthernet.HV_Batt.TCU.RX_PDUs.BMU_MODCELLTEMP.IBMU_ModCellTemp_M36B00", "AEthernet.HV_Batt.TCU.RX_PDUs.BMU_MODCELLTEMP.IBMU_ModCellTemp_M36B01", "AEthernet.HV_Batt.TCU.RX_PDUs.BMU_MODCELLTEMP.IBMU_ModCellTemp_M37B00", "AEthernet.HV_Batt.TCU.RX_PDUs.BMU_MODCELLTEMP.IBMU_ModCellTemp_M37B01", "AEthernet.HV_Batt.TCU.RX_PDUs.BMU_MODCELLTEMP.IBMU_ModCellTemp_M38B00", "AEthernet.HV_Batt.TCU.RX_PDUs.BMU_MODCELLTEMP.IBMU_ModCellTemp_M38B01", "AEthernet.HV_Batt.TCU.RX_PDUs.BMU_MODCELLTEMP.IBMU_ModCellTemp_M39B00", "AEthernet.HV_Batt.TCU.RX_PDUs.BMU_MODCELLTEMP.IBMU_ModCellTemp_M39B01", "AEthernet.HV_Batt.TCU.RX_PDUs.BMU_MODCELLTEMP.IBMU_ModCellTemp_M40B00", "AEthernet.HV_Batt.TCU.RX_PDUs.BMU_MODCELLTEMP.IBMU_ModCellTemp_M40B01", "AEthernet.HV_Batt.TCU.RX_PDUs.BMU_MODCELLTEMP.IBMU_ModCellTemp_M41B00", "AEthernet.HV_Batt.TCU.RX_PDUs.BMU_MODCELLTEMP.IBMU_ModCellTemp_M41B01", "AEthernet.HV_Batt.TCU.RX_PDUs.BMU_MODCELLTEMP.IBMU_ModCellTemp_M42B00", "AEthernet.HV_Batt.TCU.RX_PDUs.BMU_MODCELLTEMP.IBMU_ModCellTemp_M42B01", "AEthernet.HV_Batt.TCU.RX_PDUs.BMU_MODCELLTEMP.IBMU_ModCellTemp_M43B00", "AEthernet.HV_Batt.TCU.RX_PDUs.BMU_MODCELLTEMP.IBMU_ModCellTemp_M43B01", "AEthernet.HV_Batt.TCU.RX_PDUs.BMU_MODCELLTEMP.RX_deltatime", "AEthernet.HV_Batt.TCU.RX_PDUs.BMU_MODCELLTEMP.RX_time", "AEthernet.HV_Batt.TCU.RX_PDUs.BMU_MODJCTTEMP.IBMU_ModJctTemp_M00B00", "AEthernet.HV_Batt.TCU.RX_PDUs.BMU_MODJCTTEMP.IBMU_ModJctTemp_M00B01", "AEthernet.HV_Batt.TCU.RX_PDUs.BMU_MODJCTTEMP.IBMU_ModJctTemp_M01B00", "AEthernet.HV_Batt.TCU.RX_PDUs.BMU_MODJCTTEMP.IBMU_ModJctTemp_M01B01", "AEthernet.HV_Batt.TCU.RX_PDUs.BMU_MODJCTTEMP.IBMU_ModJctTemp_M02B00", "AEthernet.HV_Batt.TCU.RX_PDUs.BMU_MODJCTTEMP.IBMU_ModJctTemp_M02B01", "AEthernet.HV_Batt.TCU.RX_PDUs.BMU_MODJCTTEMP.IBMU_ModJctTemp_M03B00", "AEthernet.HV_Batt.TCU.RX_PDUs.BMU_MODJCTTEMP.IBMU_ModJctTemp_M03B01", "AEthernet.HV_Batt.TCU.RX_PDUs.BMU_MODJCTTEMP.IBMU_ModJctTemp_M04B00", "AEthernet.HV_Batt.TCU.RX_PDUs.BMU_MODJCTTEMP.IBMU_ModJctTemp_M04B01", "AEthernet.HV_Batt.TCU.RX_PDUs.BMU_MODJCTTEMP.IBMU_ModJctTemp_M05B00", "AEthernet.HV_Batt.TCU.RX_PDUs.BMU_MODJCTTEMP.IBMU_ModJctTemp_M05B01", "AEthernet.HV_Batt.TCU.RX_PDUs.BMU_MODJCTTEMP.IBMU_ModJctTemp_M06B00", "AEthernet.HV_Batt.TCU.RX_PDUs.BMU_MODJCTTEMP.IBMU_ModJctTemp_M06B01", "AEthernet.HV_Batt.TCU.RX_PDUs.BMU_MODJCTTEMP.IBMU_ModJctTemp_M07B00", "AEthernet.HV_Batt.TCU.RX_PDUs.BMU_MODJCTTEMP.IBMU_ModJctTemp_M07B01", "AEthernet.HV_Batt.TCU.RX_PDUs.BMU_MODJCTTEMP.IBMU_ModJctTemp_M08B00", "AEthernet.HV_Batt.TCU.RX_PDUs.BMU_MODJCTTEMP.IBMU_ModJctTemp_M08B01", "AEthernet.HV_Batt.TCU.RX_PDUs.BMU_MODJCTTEMP.IBMU_ModJctTemp_M09B00", "AEthernet.HV_Batt.TCU.RX_PDUs.BMU_MODJCTTEMP.IBMU_ModJctTemp_M09B01", "AEthernet.HV_Batt.TCU.RX_PDUs.BMU_MODJCTTEMP.IBMU_ModJctTemp_M10B00", "AEthernet.HV_Batt.TCU.RX_PDUs.BMU_MODJCTTEMP.IBMU_ModJctTemp_M10B01", "AEthernet.HV_Batt.TCU.RX_PDUs.BMU_MODJCTTEMP.IBMU_ModJctTemp_M11B00", "AEthernet.HV_Batt.TCU.RX_PDUs.BMU_MODJCTTEMP.IBMU_ModJctTemp_M11B01", "AEthernet.HV_Batt.TCU.RX_PDUs.BMU_MODJCTTEMP.IBMU_ModJctTemp_M12B00", "AEthernet.HV_Batt.TCU.RX_PDUs.BMU_MODJCTTEMP.IBMU_ModJctTemp_M12B01", "AEthernet.HV_Batt.TCU.RX_PDUs.BMU_MODJCTTEMP.IBMU_ModJctTemp_M13B00", "AEthernet.HV_Batt.TCU.RX_PDUs.BMU_MODJCTTEMP.IBMU_ModJctTemp_M13B01", "AEthernet.HV_Batt.TCU.RX_PDUs.BMU_MODJCTTEMP.IBMU_ModJctTemp_M14B00", "AEthernet.HV_Batt.TCU.RX_PDUs.BMU_MODJCTTEMP.IBMU_ModJctTemp_M14B01", "AEthernet.HV_Batt.TCU.RX_PDUs.BMU_MODJCTTEMP.IBMU_ModJctTemp_M15B00", "AEthernet.HV_Batt.TCU.RX_PDUs.BMU_MODJCTTEMP.IBMU_ModJctTemp_M15B01", "AEthernet.HV_Batt.TCU.RX_PDUs.BMU_MODJCTTEMP.IBMU_ModJctTemp_M16B00", "AEthernet.HV_Batt.TCU.RX_PDUs.BMU_MODJCTTEMP.IBMU_ModJctTemp_M16B01", "AEthernet.HV_Batt.TCU.RX_PDUs.BMU_MODJCTTEMP.IBMU_ModJctTemp_M17B00", "AEthernet.HV_Batt.TCU.RX_PDUs.BMU_MODJCTTEMP.IBMU_ModJctTemp_M17B01", "AEthernet.HV_Batt.TCU.RX_PDUs.BMU_MODJCTTEMP.IBMU_ModJctTemp_M18B00", "AEthernet.HV_Batt.TCU.RX_PDUs.BMU_MODJCTTEMP.IBMU_ModJctTemp_M18B01", "AEthernet.HV_Batt.TCU.RX_PDUs.BMU_MODJCTTEMP.IBMU_ModJctTemp_M19B00", "AEthernet.HV_Batt.TCU.RX_PDUs.BMU_MODJCTTEMP.IBMU_ModJctTemp_M19B01", "AEthernet.HV_Batt.TCU.RX_PDUs.BMU_MODJCTTEMP.IBMU_ModJctTemp_M20B00", "AEthernet.HV_Batt.TCU.RX_PDUs.BMU_MODJCTTEMP.IBMU_ModJctTemp_M20B01", "AEthernet.HV_Batt.TCU.RX_PDUs.BMU_MODJCTTEMP.IBMU_ModJctTemp_M21B00", "AEthernet.HV_Batt.TCU.RX_PDUs.BMU_MODJCTTEMP.IBMU_ModJctTemp_M21B01", "AEthernet.HV_Batt.TCU.RX_PDUs.BMU_MODJCTTEMP.IBMU_ModJctTemp_M22B00", "AEthernet.HV_Batt.TCU.RX_PDUs.BMU_MODJCTTEMP.IBMU_ModJctTemp_M22B01", "AEthernet.HV_Batt.TCU.RX_PDUs.BMU_MODJCTTEMP.IBMU_ModJctTemp_M23B00", "AEthernet.HV_Batt.TCU.RX_PDUs.BMU_MODJCTTEMP.IBMU_ModJctTemp_M23B01", "AEthernet.HV_Batt.TCU.RX_PDUs.BMU_MODJCTTEMP.IBMU_ModJctTemp_M24B00", "AEthernet.HV_Batt.TCU.RX_PDUs.BMU_MODJCTTEMP.IBMU_ModJctTemp_M24B01", "AEthernet.HV_Batt.TCU.RX_PDUs.BMU_MODJCTTEMP.IBMU_ModJctTemp_M25B00", "AEthernet.HV_Batt.TCU.RX_PDUs.BMU_MODJCTTEMP.IBMU_ModJctTemp_M25B01", "AEthernet.HV_Batt.TCU.RX_PDUs.BMU_MODJCTTEMP.IBMU_ModJctTemp_M26B00", "AEthernet.HV_Batt.TCU.RX_PDUs.BMU_MODJCTTEMP.IBMU_ModJctTemp_M26B01", "AEthernet.HV_Batt.TCU.RX_PDUs.BMU_MODJCTTEMP.IBMU_ModJctTemp_M27B00", "AEthernet.HV_Batt.TCU.RX_PDUs.BMU_MODJCTTEMP.IBMU_ModJctTemp_M27B01", "AEthernet.HV_Batt.TCU.RX_PDUs.BMU_MODJCTTEMP.IBMU_ModJctTemp_M28B00", "AEthernet.HV_Batt.TCU.RX_PDUs.BMU_MODJCTTEMP.IBMU_ModJctTemp_M28B01", "AEthernet.HV_Batt.TCU.RX_PDUs.BMU_MODJCTTEMP.IBMU_ModJctTemp_M29B00", "AEthernet.HV_Batt.TCU.RX_PDUs.BMU_MODJCTTEMP.IBMU_ModJctTemp_M29B01", "AEthernet.HV_Batt.TCU.RX_PDUs.BMU_MODJCTTEMP.IBMU_ModJctTemp_M30B00", "AEthernet.HV_Batt.TCU.RX_PDUs.BMU_MODJCTTEMP.IBMU_ModJctTemp_M30B01", "AEthernet.HV_Batt.TCU.RX_PDUs.BMU_MODJCTTEMP.IBMU_ModJctTemp_M31B00", "AEthernet.HV_Batt.TCU.RX_PDUs.BMU_MODJCTTEMP.IBMU_ModJctTemp_M31B01", "AEthernet.HV_Batt.TCU.RX_PDUs.BMU_MODJCTTEMP.IBMU_ModJctTemp_M32B00", "AEthernet.HV_Batt.TCU.RX_PDUs.BMU_MODJCTTEMP.IBMU_ModJctTemp_M32B01", "AEthernet.HV_Batt.TCU.RX_PDUs.BMU_MODJCTTEMP.IBMU_ModJctTemp_M33B00", "AEthernet.HV_Batt.TCU.RX_PDUs.BMU_MODJCTTEMP.IBMU_ModJctTemp_M33B01", "AEthernet.HV_Batt.TCU.RX_PDUs.BMU_MODJCTTEMP.IBMU_ModJctTemp_M34B00", "AEthernet.HV_Batt.TCU.RX_PDUs.BMU_MODJCTTEMP.IBMU_ModJctTemp_M34B01", "AEthernet.HV_Batt.TCU.RX_PDUs.BMU_MODJCTTEMP.IBMU_ModJctTemp_M35B00", "AEthernet.HV_Batt.TCU.RX_PDUs.BMU_MODJCTTEMP.IBMU_ModJctTemp_M35B01", "AEthernet.HV_Batt.TCU.RX_PDUs.BMU_MODJCTTEMP.IBMU_ModJctTemp_M36B00", "AEthernet.HV_Batt.TCU.RX_PDUs.BMU_MODJCTTEMP.IBMU_ModJctTemp_M36B01", "AEthernet.HV_Batt.TCU.RX_PDUs.BMU_MODJCTTEMP.IBMU_ModJctTemp_M37B00", "AEthernet.HV_Batt.TCU.RX_PDUs.BMU_MODJCTTEMP.IBMU_ModJctTemp_M37B01", "AEthernet.HV_Batt.TCU.RX_PDUs.BMU_MODJCTTEMP.IBMU_ModJctTemp_M38B00", "AEthernet.HV_Batt.TCU.RX_PDUs.BMU_MODJCTTEMP.IBMU_ModJctTemp_M38B01", "AEthernet.HV_Batt.TCU.RX_PDUs.BMU_MODJCTTEMP.IBMU_ModJctTemp_M39B00", "AEthernet.HV_Batt.TCU.RX_PDUs.BMU_MODJCTTEMP.IBMU_ModJctTemp_M39B01", "AEthernet.HV_Batt.TCU.RX_PDUs.BMU_MODJCTTEMP.IBMU_ModJctTemp_M40B00", "AEthernet.HV_Batt.TCU.RX_PDUs.BMU_MODJCTTEMP.IBMU_ModJctTemp_M40B01", "AEthernet.HV_Batt.TCU.RX_PDUs.BMU_MODJCTTEMP.IBMU_ModJctTemp_M41B00", "AEthernet.HV_Batt.TCU.RX_PDUs.BMU_MODJCTTEMP.IBMU_ModJctTemp_M41B01", "AEthernet.HV_Batt.TCU.RX_PDUs.BMU_MODJCTTEMP.IBMU_ModJctTemp_M42B00", "AEthernet.HV_Batt.TCU.RX_PDUs.BMU_MODJCTTEMP.IBMU_ModJctTemp_M42B01", "AEthernet.HV_Batt.TCU.RX_PDUs.BMU_MODJCTTEMP.IBMU_ModJctTemp_M43B00", "AEthernet.HV_Batt.TCU.RX_PDUs.BMU_MODJCTTEMP.IBMU_ModJctTemp_M43B01", "AEthernet.HV_Batt.TCU.RX_PDUs.BMU_MODJCTTEMP.RX_deltatime", "AEthernet.HV_Batt.TCU.RX_PDUs.BMU_MODJCTTEMP.RX_time", "AEthernet.HV_Batt.TCU.RX_PDUs.BMU_STS.IBMU_StsCntctNeg", "AEthernet.HV_Batt.TCU.RX_PDUs.BMU_STS.IBMU_StsCntctPos", "AEthernet.HV_Batt.TCU.RX_PDUs.BMU_STS.IBMU_StsHvil", "AEthernet.HV_Batt.TCU.RX_PDUs.BMU_STS.IBMU_StsMainPwrLost", "AEthernet.HV_Batt.TCU.RX_PDUs.BMU_STS.IBMU_StsRelayPwrLost", "AEthernet.HV_Batt.TCU.RX_PDUs.BMU_STS.IBMU_StsVcuStReq", "AEthernet.HV_Batt.TCU.RX_PDUs.BMU_STS.IBMU_StsUptime", "AEthernet.HV_Batt.TCU.RX_PDUs.BMU_STS.IBMU_StsFlt", "AEthernet.HV_Batt.TCU.RX_PDUs.BMU_STS.IBMU_StsOpenCntctNotif", "AEthernet.HV_Batt.TCU.RX_PDUs.BMU_STS.IBMU_StsPrechrgn", "AEthernet.HV_Batt.TCU.RX_PDUs.BMU_STS.IBMU_StsPtSt", "AEthernet.HV_Batt.TCU.RX_PDUs.BMU_STS.IBMU_StsSubSt", "AEthernet.HV_Batt.TCU.RX_PDUs.BMU_STS.IBMU_ChrgCellTempDerate", "AEthernet.HV_Batt.TCU.RX_PDUs.BMU_STS.IBMU_ChrgFltDerate", "AEthernet.HV_Batt.TCU.RX_PDUs.BMU_STS.IBMU_ChrgJctTempDerate", "AEthernet.HV_Batt.TCU.RX_PDUs.BMU_STS.IBMU_ChrgSocDerate", "AEthernet.HV_Batt.TCU.RX_PDUs.BMU_STS.IBMU_DChrgCellTempDerate", "AEthernet.HV_Batt.TCU.RX_PDUs.BMU_STS.IBMU_DChrgFltDerate", "AEthernet.HV_Batt.TCU.RX_PDUs.BMU_STS.IBMU_DChrgJctTempDerate", "AEthernet.HV_Batt.TCU.RX_PDUs.BMU_STS.IBMU_DChrgSocDerate", "AEthernet.HV_Batt.TCU.RX_PDUs.BMU_STS.RX_deltatime", "AEthernet.HV_Batt.TCU.RX_PDUs.BMU_STS.RX_time", "AEthernet.HV_Batt.TCU.RX_PDUs.BMU_WNTY.IBMU_WntyCntctStressCnt1", "AEthernet.HV_Batt.TCU.RX_PDUs.BMU_WNTY.IBMU_WntyCntctStressCnt2", "AEthernet.HV_Batt.TCU.RX_PDUs.BMU_WNTY.IBMU_WntyMaxCurr", "AEthernet.HV_Batt.TCU.RX_PDUs.BMU_WNTY.IBMU_WntyMaxVbatt", "AEthernet.HV_Batt.TCU.RX_PDUs.BMU_WNTY.IBMU_WntyMinCurr", "AEthernet.HV_Batt.TCU.RX_PDUs.BMU_WNTY.IBMU_WntyMinVbatt", "AEthernet.HV_Batt.TCU.RX_PDUs.BMU_WNTY.IBMU_WntyTotAhChrg", "AEthernet.HV_Batt.TCU.RX_PDUs.BMU_WNTY.IBMU_WntyTotAhDChrg", "AEthernet.HV_Batt.TCU.RX_PDUs.BMU_WNTY.IBMU_WntyTotAhRgn", "AEthernet.HV_Batt.TCU.RX_PDUs.BMU_WNTY.IBMU_WntyTotTiNRuntwo", "AEthernet.HV_Batt.TCU.RX_PDUs.BMU_WNTY.IBMU_WntyTotTiOn", "AEthernet.HV_Batt.TCU.RX_PDUs.BMU_WNTY.IBMU_WntyCntctStressCnt3", "AEthernet.HV_Batt.TCU.RX_PDUs.BMU_WNTY.IBMU_WntyCntctStressCnt4", "AEthernet.HV_Batt.TCU.RX_PDUs.BMU_WNTY.RX_deltatime", "AEthernet.HV_Batt.TCU.RX_PDUs.BMU_WNTY.RX_time", "AEthernet.HV_Batt.MPB.RX_PDUs.BMU_CHRG_2.IBMU_ChrgCurrTar", "AEthernet.HV_Batt.MPB.RX_PDUs.BMU_CHRG_2.IBMU_ChrgMode", "AEthernet.HV_Batt.MPB.RX_PDUs.BMU_CHRG_2.IBMU_ChrgVoltTarg", "AEthernet.HV_Batt.MPB.RX_PDUs.BMU_CHRG_2.IBMU_ChrgCmpl", "AEthernet.HV_Batt.MPB.RX_PDUs.BMU_CHRG_2.IBMU_ChrgStsGen0", "AEthernet.HV_Batt.MPB.RX_PDUs.BMU_CHRG_2.IBMU_ChrgStsGen1", "AEthernet.HV_Batt.MPB.RX_PDUs.BMU_CHRG_2.IBMU_ChrgStsGen2", "AEthernet.HV_Batt.MPB.RX_PDUs.BMU_CHRG_2.IBMU_LimContnsDChrgCurr", "AEthernet.HV_Batt.MPB.RX_PDUs.BMU_CHRG_2.RX_deltatime", "AEthernet.HV_Batt.MPB.RX_PDUs.BMU_CHRG_2.RX_time", "AEthernet.HV_Batt.MPB.RX_PDUs.BMU_CHRG_3.IBMU_LimMaxChrgCurr", "AEthernet.HV_Batt.MPB.RX_PDUs.BMU_CHRG_3.IBMU_LimMaxChrgPwr", "AEthernet.HV_Batt.MPB.RX_PDUs.BMU_CHRG_3.IBMU_LimMaxChrgVolt", "AEthernet.HV_Batt.MPB.RX_PDUs.BMU_CHRG_3.IBMU_LimMinChrgCurr", "AEthernet.HV_Batt.MPB.RX_PDUs.BMU_CHRG_3.RX_deltatime", "AEthernet.HV_Batt.MPB.RX_PDUs.BMU_CHRG_3.RX_time", "AEthernet.HV_Batt.BMU.RX_PDUs.BMU_DIAG_REQ.IDiagReqParam1", "AEthernet.HV_Batt.BMU.RX_PDUs.BMU_DIAG_REQ.IDiagReqParam2", "AEthernet.HV_Batt.BMU.RX_PDUs.BMU_DIAG_REQ.IDiagReqParam3", "AEthernet.HV_Batt.BMU.RX_PDUs.BMU_DIAG_REQ.IDiagReqParam4", "AEthernet.HV_Batt.BMU.RX_PDUs.BMU_DIAG_REQ.IDiagReqParam5", "AEthernet.HV_Batt.BMU.RX_PDUs.BMU_DIAG_REQ.IDiagReqParam6", "AEthernet.HV_Batt.BMU.RX_PDUs.BMU_DIAG_REQ.IDiagReqParam7", "AEthernet.HV_Batt.BMU.RX_PDUs.BMU_DIAG_REQ.IDiagReqParam8", "AEthernet.HV_Batt.BMU.RX_PDUs.BMU_DIAG_REQ.IDiagReqRoutId", "AEthernet.HV_Batt.BMU.RX_PDUs.BMU_DIAG_REQ.RX_deltatime", "AEthernet.HV_Batt.BMU.RX_PDUs.BMU_DIAG_REQ.RX_time", "AEthernet.HV_Batt.BMU.RX_PDUs.BMU_DbgVCU.IVCU_BmuDbgB0", "AEthernet.HV_Batt.BMU.RX_PDUs.BMU_DbgVCU.IVCU_BmuDbgB1", "AEthernet.HV_Batt.BMU.RX_PDUs.BMU_DbgVCU.IVCU_BmuDbgW0", "AEthernet.HV_Batt.BMU.RX_PDUs.BMU_DbgVCU.IVCU_BmuDbgW1", "AEthernet.HV_Batt.BMU.RX_PDUs.BMU_DbgVCU.RX_deltatime", "AEthernet.HV_Batt.BMU.RX_PDUs.BMU_DbgVCU.RX_time", "AEthernet.HV_Batt.BMU.RX_PDUs.BMU_REQ_1.IHVBatt_ChrgCurrFb", "AEthernet.HV_Batt.BMU.RX_PDUs.BMU_REQ_1.IHVBatt_ChrgVoltgFb", "AEthernet.HV_Batt.BMU.RX_PDUs.BMU_REQ_1.RX_deltatime", "AEthernet.HV_Batt.BMU.RX_PDUs.BMU_REQ_1.RX_time", "AEthernet.HV_Batt.BMU.RX_PDUs.MPB_EVSECHRG_1.IMPB_EVSEChrgProfEntryLen", "AEthernet.HV_Batt.BMU.RX_PDUs.MPB_EVSECHRG_1.IMPB_EVSEChrgProfPwr0", "AEthernet.HV_Batt.BMU.RX_PDUs.MPB_EVSECHRG_1.IMPB_EVSEChrgProfPwr1", "AEthernet.HV_Batt.BMU.RX_PDUs.MPB_EVSECHRG_1.IMPB_EVSEChrgProfPwr2", "AEthernet.HV_Batt.BMU.RX_PDUs.MPB_EVSECHRG_1.IMPB_EVSEChrgProfPwr3", "AEthernet.HV_Batt.BMU.RX_PDUs.MPB_EVSECHRG_1.IMPB_EVSEChrgProfPwr4", "AEthernet.HV_Batt.BMU.RX_PDUs.MPB_EVSECHRG_1.IMPB_EVSEChrgProfPwr5", "AEthernet.HV_Batt.BMU.RX_PDUs.MPB_EVSECHRG_1.IMPB_EVSEChrgProfPwr6", "AEthernet.HV_Batt.BMU.RX_PDUs.MPB_EVSECHRG_1.IMPB_EVSEChrgProfPwr7", "AEthernet.HV_Batt.BMU.RX_PDUs.MPB_EVSECHRG_1.IMPB_EVSECurrRglnTolr", "AEthernet.HV_Batt.BMU.RX_PDUs.MPB_EVSECHRG_1.IMPB_EVSECurrRglnTolrOpt", "AEthernet.HV_Batt.BMU.RX_PDUs.MPB_EVSECHRG_1.IMPB_EVSEEgyReq", "AEthernet.HV_Batt.BMU.RX_PDUs.MPB_EVSECHRG_1.IMPB_EVSEEgyReqOpt", "AEthernet.HV_Batt.BMU.RX_PDUs.MPB_EVSECHRG_1.IMPB_EVSEPeakCurrRip", "AEthernet.HV_Batt.BMU.RX_PDUs.MPB_EVSECHRG_1.RX_deltatime", "AEthernet.HV_Batt.BMU.RX_PDUs.MPB_EVSECHRG_1.RX_time", "AEthernet.HV_Batt.BMU.RX_PDUs.MPB_EVSECHRG_2.IMPB_EVSEChrgProfTi0", "AEthernet.HV_Batt.BMU.RX_PDUs.MPB_EVSECHRG_2.IMPB_EVSEChrgProfTi1", "AEthernet.HV_Batt.BMU.RX_PDUs.MPB_EVSECHRG_2.IMPB_EVSEChrgProfTi2", "AEthernet.HV_Batt.BMU.RX_PDUs.MPB_EVSECHRG_2.IMPB_EVSEChrgProfTi3", "AEthernet.HV_Batt.BMU.RX_PDUs.MPB_EVSECHRG_2.IMPB_EVSEChrgProfTi4", "AEthernet.HV_Batt.BMU.RX_PDUs.MPB_EVSECHRG_2.IMPB_EVSEChrgProfTi5", "AEthernet.HV_Batt.BMU.RX_PDUs.MPB_EVSECHRG_2.IMPB_EVSEChrgProfTi6", "AEthernet.HV_Batt.BMU.RX_PDUs.MPB_EVSECHRG_2.IMPB_EVSEChrgProfTi7", "AEthernet.HV_Batt.BMU.RX_PDUs.MPB_EVSECHRG_2.RX_deltatime", "AEthernet.HV_Batt.BMU.RX_PDUs.MPB_EVSECHRG_2.RX_time", "AEthernet.HV_Batt.BMU.RX_PDUs.MPB_EVSECHRG_3.IMPB_ChrgStsGen0", "AEthernet.HV_Batt.BMU.RX_PDUs.MPB_EVSECHRG_3.IMPB_ChrgStsGen1", "AEthernet.HV_Batt.BMU.RX_PDUs.MPB_EVSECHRG_3.IMPB_ChrgStsGen2", "AEthernet.HV_Batt.BMU.RX_PDUs.MPB_EVSECHRG_3.IMPB_EVSEIsoSts", "AEthernet.HV_Batt.BMU.RX_PDUs.MPB_EVSECHRG_3.IMPB_EVSEIsoStsOpt", "AEthernet.HV_Batt.BMU.RX_PDUs.MPB_EVSECHRG_3.IMPB_EVSELimChrgCurr", "AEthernet.HV_Batt.BMU.RX_PDUs.MPB_EVSECHRG_3.IMPB_EVSELimChrgVolt", "AEthernet.HV_Batt.BMU.RX_PDUs.MPB_EVSECHRG_3.IMPB_EVSEStsFlg", "AEthernet.HV_Batt.BMU.RX_PDUs.MPB_EVSECHRG_3.IMPB_ChrgMod", "AEthernet.HV_Batt.BMU.RX_PDUs.MPB_EVSECHRG_3.RX_deltatime", "AEthernet.HV_Batt.BMU.RX_PDUs.MPB_EVSECHRG_3.RX_time", "AEthernet.HV_Batt.BMU.RX_PDUs.MPB_EVSECHRG_4.IMPB_EVSELimMaxChrgCurr", "AEthernet.HV_Batt.BMU.RX_PDUs.MPB_EVSECHRG_4.IMPB_EVSELimMaxChrgCurrOpt", "AEthernet.HV_Batt.BMU.RX_PDUs.MPB_EVSECHRG_4.IMPB_EVSELimMaxChrgPwr", "AEthernet.HV_Batt.BMU.RX_PDUs.MPB_EVSECHRG_4.IMPB_EVSELimMaxChrgPwrOpt", "AEthernet.HV_Batt.BMU.RX_PDUs.MPB_EVSECHRG_4.IMPB_EVSELimMaxChrgVolt", "AEthernet.HV_Batt.BMU.RX_PDUs.MPB_EVSECHRG_4.IMPB_EVSELimMaxChrgVoltOpt", "AEthernet.HV_Batt.BMU.RX_PDUs.MPB_EVSECHRG_4.IMPB_EVSELimMinChrgCurr", "AEthernet.HV_Batt.BMU.RX_PDUs.MPB_EVSECHRG_4.IMPB_EVSELimMinChrgVolt", "AEthernet.HV_Batt.BMU.RX_PDUs.MPB_EVSECHRG_4.IMPB_EVSENomVolt", "AEthernet.HV_Batt.BMU.RX_PDUs.MPB_EVSECHRG_4.RX_deltatime", "AEthernet.HV_Batt.BMU.RX_PDUs.MPB_EVSECHRG_4.RX_time", "AEthernet.HV_Batt.BMU.RX_PDUs.VCU_TO_BMU.IVCU_BattCoolFlowRate", "AEthernet.HV_Batt.BMU.RX_PDUs.VCU_TO_BMU.IVCU_BattTempCoolIn", "AEthernet.HV_Batt.BMU.RX_PDUs.VCU_TO_BMU.IVCU_VehUseModCurr", "AEthernet.HV_Batt.BMU.RX_PDUs.VCU_TO_BMU.IVCU_VehUseModNxt", "AEthernet.HV_Batt.BMU.RX_PDUs.VCU_TO_BMU.IVCU_EgyCnsBfrChrg", "AEthernet.HV_Batt.BMU.RX_PDUs.VCU_TO_BMU.RX_deltatime", "AEthernet.HV_Batt.BMU.RX_PDUs.VCU_TO_BMU.RX_time", "AEthernet.HV_Batt.BCM.RX_PDUs.BMU_CHRG_2.IBMU_ChrgCurrTar", "AEthernet.HV_Batt.BCM.RX_PDUs.BMU_CHRG_2.IBMU_ChrgMode", "AEthernet.HV_Batt.BCM.RX_PDUs.BMU_CHRG_2.IBMU_ChrgVoltTarg", "AEthernet.HV_Batt.BCM.RX_PDUs.BMU_CHRG_2.IBMU_ChrgCmpl", "AEthernet.HV_Batt.BCM.RX_PDUs.BMU_CHRG_2.IBMU_ChrgStsGen0", "AEthernet.HV_Batt.BCM.RX_PDUs.BMU_CHRG_2.IBMU_ChrgStsGen1", "AEthernet.HV_Batt.BCM.RX_PDUs.BMU_CHRG_2.IBMU_ChrgStsGen2", "AEthernet.HV_Batt.BCM.RX_PDUs.BMU_CHRG_2.IBMU_LimContnsDChrgCurr", "AEthernet.HV_Batt.BCM.RX_PDUs.BMU_CHRG_2.RX_deltatime", "AEthernet.HV_Batt.BCM.RX_PDUs.BMU_CHRG_2.RX_time", "AEthernet.InfoT_Chassis.VCU_RFEGW.RX_PDUs.BMU_ALGO.IBMU_AlgoPkCpEst", "AEthernet.InfoT_Chassis.VCU_RFEGW.RX_PDUs.BMU_ALGO.IBMU_AlgoPkSocCoulombCnt", "AEthernet.InfoT_Chassis.VCU_RFEGW.RX_PDUs.BMU_ALGO.IBMU_AlgoPkSocMax", "AEthernet.InfoT_Chassis.VCU_RFEGW.RX_PDUs.BMU_ALGO.IBMU_AlgoPkSocMin", "AEthernet.InfoT_Chassis.VCU_RFEGW.RX_PDUs.BMU_ALGO.IBMU_AlgoPkSocEkf", "AEthernet.InfoT_Chassis.VCU_RFEGW.RX_PDUs.BMU_ALGO.IBMU_AlgoCalR0", "AEthernet.InfoT_Chassis.VCU_RFEGW.RX_PDUs.BMU_ALGO.IBMU_AlgoEstR0", "AEthernet.InfoT_Chassis.VCU_RFEGW.RX_PDUs.BMU_ALGO.IBMU_AlgoEstVoltErr", "AEthernet.InfoT_Chassis.VCU_RFEGW.RX_PDUs.BMU_ALGO.IBMU_AlgoPkSocTrue", "AEthernet.InfoT_Chassis.VCU_RFEGW.RX_PDUs.BMU_ALGO.IBMU_AlgoPkSoh", "AEthernet.InfoT_Chassis.VCU_RFEGW.RX_PDUs.BMU_ALGO.IBMU_AlgoPkSoe", "AEthernet.InfoT_Chassis.VCU_RFEGW.RX_PDUs.BMU_ALGO.IBMU_AlgoRemngChrgTiBulk", "AEthernet.InfoT_Chassis.VCU_RFEGW.RX_PDUs.BMU_ALGO.IBMU_AlgoRemngChrgTi", "AEthernet.InfoT_Chassis.VCU_RFEGW.RX_PDUs.BMU_ALGO.IBMU_AlgoPkEgy", "AEthernet.InfoT_Chassis.VCU_RFEGW.RX_PDUs.BMU_ALGO.IBMU_AlgoPkSoc", "AEthernet.InfoT_Chassis.VCU_RFEGW.RX_PDUs.BMU_ALGO.IBMU_AlgoRemngEgy", "AEthernet.InfoT_Chassis.VCU_RFEGW.RX_PDUs.BMU_ALGO.IBMU_ChrgAllwDChrg", "AEthernet.InfoT_Chassis.VCU_RFEGW.RX_PDUs.BMU_ALGO.RX_deltatime", "AEthernet.InfoT_Chassis.VCU_RFEGW.RX_PDUs.BMU_ALGO.RX_time", "AEthernet.InfoT_Chassis.TCU.RX_PDUs.BMU_ALGO.IBMU_AlgoPkCpEst", "AEthernet.InfoT_Chassis.TCU.RX_PDUs.BMU_ALGO.IBMU_AlgoPkSocCoulombCnt", "AEthernet.InfoT_Chassis.TCU.RX_PDUs.BMU_ALGO.IBMU_AlgoPkSocMax", "AEthernet.InfoT_Chassis.TCU.RX_PDUs.BMU_ALGO.IBMU_AlgoPkSocMin", "AEthernet.InfoT_Chassis.TCU.RX_PDUs.BMU_ALGO.IBMU_AlgoPkSocEkf", "AEthernet.InfoT_Chassis.TCU.RX_PDUs.BMU_ALGO.IBMU_AlgoCalR0", "AEthernet.InfoT_Chassis.TCU.RX_PDUs.BMU_ALGO.IBMU_AlgoEstR0", "AEthernet.InfoT_Chassis.TCU.RX_PDUs.BMU_ALGO.IBMU_AlgoEstVoltErr", "AEthernet.InfoT_Chassis.TCU.RX_PDUs.BMU_ALGO.IBMU_AlgoPkSocTrue", "AEthernet.InfoT_Chassis.TCU.RX_PDUs.BMU_ALGO.IBMU_AlgoPkSoh", "AEthernet.InfoT_Chassis.TCU.RX_PDUs.BMU_ALGO.IBMU_AlgoPkSoe", "AEthernet.InfoT_Chassis.TCU.RX_PDUs.BMU_ALGO.IBMU_AlgoRemngChrgTiBulk", "AEthernet.InfoT_Chassis.TCU.RX_PDUs.BMU_ALGO.IBMU_AlgoRemngChrgTi", "AEthernet.InfoT_Chassis.TCU.RX_PDUs.BMU_ALGO.IBMU_AlgoPkEgy", "AEthernet.InfoT_Chassis.TCU.RX_PDUs.BMU_ALGO.IBMU_AlgoPkSoc", "AEthernet.InfoT_Chassis.TCU.RX_PDUs.BMU_ALGO.IBMU_AlgoRemngEgy", "AEthernet.InfoT_Chassis.TCU.RX_PDUs.BMU_ALGO.IBMU_ChrgAllwDChrg", "AEthernet.InfoT_Chassis.TCU.RX_PDUs.BMU_ALGO.RX_deltatime", "AEthernet.InfoT_Chassis.TCU.RX_PDUs.BMU_ALGO.RX_time", "AEthernet.InfoT_Chassis.MPB.RX_PDUs.BMU_ALGO.IBMU_AlgoPkCpEst", "AEthernet.InfoT_Chassis.MPB.RX_PDUs.BMU_ALGO.IBMU_AlgoPkSocCoulombCnt", "AEthernet.InfoT_Chassis.MPB.RX_PDUs.BMU_ALGO.IBMU_AlgoPkSocMax", "AEthernet.InfoT_Chassis.MPB.RX_PDUs.BMU_ALGO.IBMU_AlgoPkSocMin", "AEthernet.InfoT_Chassis.MPB.RX_PDUs.BMU_ALGO.IBMU_AlgoPkSocEkf", "AEthernet.InfoT_Chassis.MPB.RX_PDUs.BMU_ALGO.IBMU_AlgoCalR0", "AEthernet.InfoT_Chassis.MPB.RX_PDUs.BMU_ALGO.IBMU_AlgoEstR0", "AEthernet.InfoT_Chassis.MPB.RX_PDUs.BMU_ALGO.IBMU_AlgoEstVoltErr", "AEthernet.InfoT_Chassis.MPB.RX_PDUs.BMU_ALGO.IBMU_AlgoPkSocTrue", "AEthernet.InfoT_Chassis.MPB.RX_PDUs.BMU_ALGO.IBMU_AlgoPkSoh", "AEthernet.InfoT_Chassis.MPB.RX_PDUs.BMU_ALGO.IBMU_AlgoPkSoe", "AEthernet.InfoT_Chassis.MPB.RX_PDUs.BMU_ALGO.IBMU_AlgoRemngChrgTiBulk", "AEthernet.InfoT_Chassis.MPB.RX_PDUs.BMU_ALGO.IBMU_AlgoRemngChrgTi", "AEthernet.InfoT_Chassis.MPB.RX_PDUs.BMU_ALGO.IBMU_AlgoPkEgy", "AEthernet.InfoT_Chassis.MPB.RX_PDUs.BMU_ALGO.IBMU_AlgoPkSoc", "AEthernet.InfoT_Chassis.MPB.RX_PDUs.BMU_ALGO.IBMU_AlgoRemngEgy", "AEthernet.InfoT_Chassis.MPB.RX_PDUs.BMU_ALGO.IBMU_ChrgAllwDChrg", "AEthernet.InfoT_Chassis.MPB.RX_PDUs.BMU_ALGO.RX_deltatime", "AEthernet.InfoT_Chassis.MPB.RX_PDUs.BMU_ALGO.RX_time", "AEthernet.InfoT_Chassis.ICC.RX_PDUs.BMU_ALGO.IBMU_AlgoPkCpEst", "AEthernet.InfoT_Chassis.ICC.RX_PDUs.BMU_ALGO.IBMU_AlgoPkSocCoulombCnt", "AEthernet.InfoT_Chassis.ICC.RX_PDUs.BMU_ALGO.IBMU_AlgoPkSocMax", "AEthernet.InfoT_Chassis.ICC.RX_PDUs.BMU_ALGO.IBMU_AlgoPkSocMin", "AEthernet.InfoT_Chassis.ICC.RX_PDUs.BMU_ALGO.IBMU_AlgoPkSocEkf", "AEthernet.InfoT_Chassis.ICC.RX_PDUs.BMU_ALGO.IBMU_AlgoCalR0", "AEthernet.InfoT_Chassis.ICC.RX_PDUs.BMU_ALGO.IBMU_AlgoEstR0", "AEthernet.InfoT_Chassis.ICC.RX_PDUs.BMU_ALGO.IBMU_AlgoEstVoltErr", "AEthernet.InfoT_Chassis.ICC.RX_PDUs.BMU_ALGO.IBMU_AlgoPkSocTrue", "AEthernet.InfoT_Chassis.ICC.RX_PDUs.BMU_ALGO.IBMU_AlgoPkSoh", "AEthernet.InfoT_Chassis.ICC.RX_PDUs.BMU_ALGO.IBMU_AlgoPkSoe", "AEthernet.InfoT_Chassis.ICC.RX_PDUs.BMU_ALGO.IBMU_AlgoRemngChrgTiBulk", "AEthernet.InfoT_Chassis.ICC.RX_PDUs.BMU_ALGO.IBMU_AlgoRemngChrgTi", "AEthernet.InfoT_Chassis.ICC.RX_PDUs.BMU_ALGO.IBMU_AlgoPkEgy", "AEthernet.InfoT_Chassis.ICC.RX_PDUs.BMU_ALGO.IBMU_AlgoPkSoc", "AEthernet.InfoT_Chassis.ICC.RX_PDUs.BMU_ALGO.IBMU_AlgoRemngEgy", "AEthernet.InfoT_Chassis.ICC.RX_PDUs.BMU_ALGO.IBMU_ChrgAllwDChrg", "AEthernet.InfoT_Chassis.ICC.RX_PDUs.BMU_ALGO.RX_deltatime", "AEthernet.InfoT_Chassis.ICC.RX_PDUs.BMU_ALGO.RX_time", "AEthernet.InfoT_Chassis.CCC.RX_PDUs.BMU_ALGO.IBMU_AlgoPkCpEst", "AEthernet.InfoT_Chassis.CCC.RX_PDUs.BMU_ALGO.IBMU_AlgoPkSocCoulombCnt", "AEthernet.InfoT_Chassis.CCC.RX_PDUs.BMU_ALGO.IBMU_AlgoPkSocMax", "AEthernet.InfoT_Chassis.CCC.RX_PDUs.BMU_ALGO.IBMU_AlgoPkSocMin", "AEthernet.InfoT_Chassis.CCC.RX_PDUs.BMU_ALGO.IBMU_AlgoPkSocEkf", "AEthernet.InfoT_Chassis.CCC.RX_PDUs.BMU_ALGO.IBMU_AlgoCalR0", "AEthernet.InfoT_Chassis.CCC.RX_PDUs.BMU_ALGO.IBMU_AlgoEstR0", "AEthernet.InfoT_Chassis.CCC.RX_PDUs.BMU_ALGO.IBMU_AlgoEstVoltErr", "AEthernet.InfoT_Chassis.CCC.RX_PDUs.BMU_ALGO.IBMU_AlgoPkSocTrue", "AEthernet.InfoT_Chassis.CCC.RX_PDUs.BMU_ALGO.IBMU_AlgoPkSoh", "AEthernet.InfoT_Chassis.CCC.RX_PDUs.BMU_ALGO.IBMU_AlgoPkSoe", "AEthernet.InfoT_Chassis.CCC.RX_PDUs.BMU_ALGO.IBMU_AlgoRemngChrgTiBulk", "AEthernet.InfoT_Chassis.CCC.RX_PDUs.BMU_ALGO.IBMU_AlgoRemngChrgTi", "AEthernet.InfoT_Chassis.CCC.RX_PDUs.BMU_ALGO.IBMU_AlgoPkEgy", "AEthernet.InfoT_Chassis.CCC.RX_PDUs.BMU_ALGO.IBMU_AlgoPkSoc", "AEthernet.InfoT_Chassis.CCC.RX_PDUs.BMU_ALGO.IBMU_AlgoRemngEgy", "AEthernet.InfoT_Chassis.CCC.RX_PDUs.BMU_ALGO.IBMU_ChrgAllwDChrg", "AEthernet.InfoT_Chassis.CCC.RX_PDUs.BMU_ALGO.RX_deltatime", "AEthernet.InfoT_Chassis.CCC.RX_PDUs.BMU_ALGO.RX_time", "AEthernet.InfoT_Chassis.BMU.RX_PDUs.CCC_CHRG.ICCC_ChrgTarSoe", "AEthernet.InfoT_Chassis.BMU.RX_PDUs.CCC_CHRG.ICCC_ChrgCmd", "AEthernet.InfoT_Chassis.BMU.RX_PDUs.CCC_CHRG.RX_deltatime", "AEthernet.InfoT_Chassis.BMU.RX_PDUs.CCC_CHRG.RX_time", "AEthernet.InfoT_Chassis.BMU.RX_PDUs.PM_VEHPWRST.IVSM_VehPwrSt", "AEthernet.InfoT_Chassis.BMU.RX_PDUs.PM_VEHPWRST.IVSM_LoPwrModActv", "AEthernet.InfoT_Chassis.BMU.RX_PDUs.PM_VEHPWRST.RX_deltatime", "AEthernet.InfoT_Chassis.BMU.RX_PDUs.PM_VEHPWRST.RX_time", "AEthernet.InfoT_Chassis.BMU.RX_PDUs.TCU_MobileAppReq_ChrgCntl.ITCU_ChrgCntlReq", "AEthernet.InfoT_Chassis.BMU.RX_PDUs.TCU_MobileAppReq_ChrgCntl.ITCU_ChrgLimSet", "AEthernet.InfoT_Chassis.BMU.RX_PDUs.TCU_MobileAppReq_ChrgCntl.RX_deltatime", "AEthernet.InfoT_Chassis.BMU.RX_PDUs.TCU_MobileAppReq_ChrgCntl.RX_time", "AEthernet.InfoT_Chassis.BMU.RX_PDUs.VCU_ODO.IOdometer", "AEthernet.InfoT_Chassis.BMU.RX_PDUs.VCU_ODO.RX_deltatime", "AEthernet.InfoT_Chassis.BMU.RX_PDUs.VCU_ODO.RX_time", "AEthernet.InfoT_Chassis.BMU.RX_PDUs.VCU_to_ICC.IVCU_CrpModSt", "AEthernet.InfoT_Chassis.BMU.RX_PDUs.VCU_to_ICC.IVCU_DrvMod", "AEthernet.InfoT_Chassis.BMU.RX_PDUs.VCU_to_ICC.IVCU_RgnBrkgOnOffSt", "AEthernet.InfoT_Chassis.BMU.RX_PDUs.VCU_to_ICC.IHvacDemistResp", "AEthernet.InfoT_Chassis.BMU.RX_PDUs.VCU_to_ICC.IVehRngTotAvl", "AEthernet.InfoT_Chassis.BMU.RX_PDUs.VCU_to_ICC.IVCU_WheelDriveModeResp", "AEthernet.InfoT_Chassis.BMU.RX_PDUs.VCU_to_ICC.IVCU_ChrgSts", "AEthernet.InfoT_Chassis.BMU.RX_PDUs.VCU_to_ICC.IVCU_CooltLvlCab", "AEthernet.InfoT_Chassis.BMU.RX_PDUs.VCU_to_ICC.IVCU_CooltLvlPt", "AEthernet.InfoT_Chassis.BMU.RX_PDUs.VCU_to_ICC.IVCU_VehRngChrgdInSession", "AEthernet.InfoT_Chassis.BMU.RX_PDUs.VCU_to_ICC.IVCU_WshrFldLvl", "AEthernet.InfoT_Chassis.BMU.RX_PDUs.VCU_to_ICC.IVCU_VehChrgRateKph", "AEthernet.InfoT_Chassis.BMU.RX_PDUs.VCU_to_ICC.RX_deltatime", "AEthernet.InfoT_Chassis.BMU.RX_PDUs.VCU_to_ICC.RX_time", "AEthernet.InfoT_Powertrain.VCU_RFEGW.RX_PDUs.BMU_LIM_1.IBMU_LimMaxDChrgPwr", "AEthernet.InfoT_Powertrain.VCU_RFEGW.RX_PDUs.BMU_LIM_1.IBMU_LimMaxRgnPwr", "AEthernet.InfoT_Powertrain.VCU_RFEGW.RX_PDUs.BMU_LIM_1.IBMU_LimMaxDChrgCurr", "AEthernet.InfoT_Powertrain.VCU_RFEGW.RX_PDUs.BMU_LIM_1.IBMU_LimMaxRgnCurr", "AEthernet.InfoT_Powertrain.VCU_RFEGW.RX_PDUs.BMU_LIM_1.IBMU_LimCurrTempMax", "AEthernet.InfoT_Powertrain.VCU_RFEGW.RX_PDUs.BMU_LIM_1.IBMU_LimCurrTempMin", "AEthernet.InfoT_Powertrain.VCU_RFEGW.RX_PDUs.BMU_LIM_1.IBMU_LimNxtTempMax", "AEthernet.InfoT_Powertrain.VCU_RFEGW.RX_PDUs.BMU_LIM_1.IBMU_LimNxtTempMin", "AEthernet.InfoT_Powertrain.VCU_RFEGW.RX_PDUs.BMU_LIM_1.RX_deltatime", "AEthernet.InfoT_Powertrain.VCU_RFEGW.RX_PDUs.BMU_LIM_1.RX_time", "AEthernet.InfoT_Powertrain.VCU_RFEGW.RX_PDUs.BMU_STATS_1.IBMU_StatsPkHum", "AEthernet.InfoT_Powertrain.VCU_RFEGW.RX_PDUs.BMU_STATS_1.IBMU_StatsPkTempCellMaxBlk", "AEthernet.InfoT_Powertrain.VCU_RFEGW.RX_PDUs.BMU_STATS_1.IBMU_StatsPkTempCellMaxMod", "AEthernet.InfoT_Powertrain.VCU_RFEGW.RX_PDUs.BMU_STATS_1.IBMU_StatsPkTempCellMinBlk", "AEthernet.InfoT_Powertrain.VCU_RFEGW.RX_PDUs.BMU_STATS_1.IBMU_StatsPkTempCellMinMod", "AEthernet.InfoT_Powertrain.VCU_RFEGW.RX_PDUs.BMU_STATS_1.IBMU_StatsTempCellDelta", "AEthernet.InfoT_Powertrain.VCU_RFEGW.RX_PDUs.BMU_STATS_1.IBMU_StatsTempCoolIn", "AEthernet.InfoT_Powertrain.VCU_RFEGW.RX_PDUs.BMU_STATS_1.IBMU_StatsPkBlkVoltDelta", "AEthernet.InfoT_Powertrain.VCU_RFEGW.RX_PDUs.BMU_STATS_1.IBMU_StatsHvTemp1", "AEthernet.InfoT_Powertrain.VCU_RFEGW.RX_PDUs.BMU_STATS_1.IBMU_StatsHvTemp2", "AEthernet.InfoT_Powertrain.VCU_RFEGW.RX_PDUs.BMU_STATS_1.IBMU_StatsHvTemp3", "AEthernet.InfoT_Powertrain.VCU_RFEGW.RX_PDUs.BMU_STATS_1.IBMU_StatsHvTemp4", "AEthernet.InfoT_Powertrain.VCU_RFEGW.RX_PDUs.BMU_STATS_1.IBMU_StatsHvTemp5", "AEthernet.InfoT_Powertrain.VCU_RFEGW.RX_PDUs.BMU_STATS_1.IBMU_StatsHvTemp6", "AEthernet.InfoT_Powertrain.VCU_RFEGW.RX_PDUs.BMU_STATS_1.IBMU_StatsHvTemp7", "AEthernet.InfoT_Powertrain.VCU_RFEGW.RX_PDUs.BMU_STATS_1.IBMU_StatsHvTemp8", "AEthernet.InfoT_Powertrain.VCU_RFEGW.RX_PDUs.BMU_STATS_1.IBMU_StatsHvTemp9", "AEthernet.InfoT_Powertrain.VCU_RFEGW.RX_PDUs.BMU_STATS_1.IBMU_StatsHvTemp10", "AEthernet.InfoT_Powertrain.VCU_RFEGW.RX_PDUs.BMU_STATS_1.IBMU_StatsHvTemp11", "AEthernet.InfoT_Powertrain.VCU_RFEGW.RX_PDUs.BMU_STATS_1.IBMU_StatsHvTemp12", "AEthernet.InfoT_Powertrain.VCU_RFEGW.RX_PDUs.BMU_STATS_1.IBMU_StatsHvTemp13", "AEthernet.InfoT_Powertrain.VCU_RFEGW.RX_PDUs.BMU_STATS_1.IBMU_StatsHvTemp14", "AEthernet.InfoT_Powertrain.VCU_RFEGW.RX_PDUs.BMU_STATS_1.IBMU_StatsPkAmbTemp", "AEthernet.InfoT_Powertrain.VCU_RFEGW.RX_PDUs.BMU_STATS_1.IBMU_StatsPkDewPointTemp", "AEthernet.InfoT_Powertrain.VCU_RFEGW.RX_PDUs.BMU_STATS_1.IBMU_StatsPkTempInterconMax", "AEthernet.InfoT_Powertrain.VCU_RFEGW.RX_PDUs.BMU_STATS_1.IBMU_StatsPkTempInterconMin", "AEthernet.InfoT_Powertrain.VCU_RFEGW.RX_PDUs.BMU_STATS_1.IBMU_StatsPkTempCellMax", "AEthernet.InfoT_Powertrain.VCU_RFEGW.RX_PDUs.BMU_STATS_1.IBMU_StatsPkTempCellMin", "AEthernet.InfoT_Powertrain.VCU_RFEGW.RX_PDUs.BMU_STATS_1.IBMU_StatsTempCellMax", "AEthernet.InfoT_Powertrain.VCU_RFEGW.RX_PDUs.BMU_STATS_1.IBMU_StatsTempCellMin", "AEthernet.InfoT_Powertrain.VCU_RFEGW.RX_PDUs.BMU_STATS_1.IBMU_StatsPkBlkVoltMax0", "AEthernet.InfoT_Powertrain.VCU_RFEGW.RX_PDUs.BMU_STATS_1.IBMU_StatsPkBlkVoltMax0Blk", "AEthernet.InfoT_Powertrain.VCU_RFEGW.RX_PDUs.BMU_STATS_1.IBMU_StatsPkBlkVoltMax0Mod", "AEthernet.InfoT_Powertrain.VCU_RFEGW.RX_PDUs.BMU_STATS_1.IBMU_StatsPkBlkVoltMax1", "AEthernet.InfoT_Powertrain.VCU_RFEGW.RX_PDUs.BMU_STATS_1.IBMU_StatsPkBlkVoltMax1Blk", "AEthernet.InfoT_Powertrain.VCU_RFEGW.RX_PDUs.BMU_STATS_1.IBMU_StatsPkBlkVoltMax1Mod", "AEthernet.InfoT_Powertrain.VCU_RFEGW.RX_PDUs.BMU_STATS_1.IBMU_StatsPkBlkVoltMax2", "AEthernet.InfoT_Powertrain.VCU_RFEGW.RX_PDUs.BMU_STATS_1.IBMU_StatsPkBlkVoltMax2Blk", "AEthernet.InfoT_Powertrain.VCU_RFEGW.RX_PDUs.BMU_STATS_1.IBMU_StatsPkBlkVoltMax2Mod", "AEthernet.InfoT_Powertrain.VCU_RFEGW.RX_PDUs.BMU_STATS_1.IBMU_StatsPkBlkVoltMax3", "AEthernet.InfoT_Powertrain.VCU_RFEGW.RX_PDUs.BMU_STATS_1.IBMU_StatsPkBlkVoltMax3Blk", "AEthernet.InfoT_Powertrain.VCU_RFEGW.RX_PDUs.BMU_STATS_1.IBMU_StatsPkBlkVoltMax3Mod", "AEthernet.InfoT_Powertrain.VCU_RFEGW.RX_PDUs.BMU_STATS_1.IBMU_StatsPkBlkVoltMin0", "AEthernet.InfoT_Powertrain.VCU_RFEGW.RX_PDUs.BMU_STATS_1.IBMU_StatsPkBlkVoltMin0Blk", "AEthernet.InfoT_Powertrain.VCU_RFEGW.RX_PDUs.BMU_STATS_1.IBMU_StatsPkBlkVoltMin0Mod", "AEthernet.InfoT_Powertrain.VCU_RFEGW.RX_PDUs.BMU_STATS_1.IBMU_StatsPkBlkVoltMin1", "AEthernet.InfoT_Powertrain.VCU_RFEGW.RX_PDUs.BMU_STATS_1.IBMU_StatsPkBlkVoltMin1Blk", "AEthernet.InfoT_Powertrain.VCU_RFEGW.RX_PDUs.BMU_STATS_1.IBMU_StatsPkBlkVoltMin1Mod", "AEthernet.InfoT_Powertrain.VCU_RFEGW.RX_PDUs.BMU_STATS_1.IBMU_StatsPkBlkVoltMin2", "AEthernet.InfoT_Powertrain.VCU_RFEGW.RX_PDUs.BMU_STATS_1.IBMU_StatsPkBlkVoltMin2Blk", "AEthernet.InfoT_Powertrain.VCU_RFEGW.RX_PDUs.BMU_STATS_1.IBMU_StatsPkBlkVoltMin2Mod", "AEthernet.InfoT_Powertrain.VCU_RFEGW.RX_PDUs.BMU_STATS_1.IBMU_StatsPkBlkVoltMin3", "AEthernet.InfoT_Powertrain.VCU_RFEGW.RX_PDUs.BMU_STATS_1.IBMU_StatsPkBlkVoltMin3Blk", "AEthernet.InfoT_Powertrain.VCU_RFEGW.RX_PDUs.BMU_STATS_1.IBMU_StatsPkBlkVoltMin3Mod", "AEthernet.InfoT_Powertrain.VCU_RFEGW.RX_PDUs.BMU_STATS_1.IBMU_StatsPkP", "AEthernet.InfoT_Powertrain.VCU_RFEGW.RX_PDUs.BMU_STATS_1.RX_deltatime", "AEthernet.InfoT_Powertrain.VCU_RFEGW.RX_PDUs.BMU_STATS_1.RX_time", "AEthernet.InfoT_Powertrain.VCU_RFEGW.RX_PDUs.BMU_STATS_2.IBMU_StatsPkCurr", "AEthernet.InfoT_Powertrain.VCU_RFEGW.RX_PDUs.BMU_STATS_2.IBMU_StatsPkVbatt", "AEthernet.InfoT_Powertrain.VCU_RFEGW.RX_PDUs.BMU_STATS_2.IBMU_StatsPkVout", "AEthernet.InfoT_Powertrain.VCU_RFEGW.RX_PDUs.BMU_STATS_2.IBMU_StatsPkVbattsum", "AEthernet.InfoT_Powertrain.VCU_RFEGW.RX_PDUs.BMU_STATS_2.IBMU_StatsPkCurrUnsyncd", "AEthernet.InfoT_Powertrain.VCU_RFEGW.RX_PDUs.BMU_STATS_2.IBMU_StatsPkIso", "AEthernet.InfoT_Powertrain.VCU_RFEGW.RX_PDUs.BMU_STATS_2.IBMU_StatsPkPwr", "AEthernet.InfoT_Powertrain.VCU_RFEGW.RX_PDUs.BMU_STATS_2.RX_deltatime", "AEthernet.InfoT_Powertrain.VCU_RFEGW.RX_PDUs.BMU_STATS_2.RX_time", "AEthernet.InfoT_Powertrain.TCU.RX_PDUs.BMU_FLTRPT.IBMU_FltRptBlkVoltOver", "AEthernet.InfoT_Powertrain.TCU.RX_PDUs.BMU_FLTRPT.IBMU_FltRptBlkVoltUnder", "AEthernet.InfoT_Powertrain.TCU.RX_PDUs.BMU_FLTRPT.IBMU_FltRptHvil", "AEthernet.InfoT_Powertrain.TCU.RX_PDUs.BMU_FLTRPT.IBMU_FltRptIso", "AEthernet.InfoT_Powertrain.TCU.RX_PDUs.BMU_FLTRPT.IBMU_FltRptPkCurrOver", "AEthernet.InfoT_Powertrain.TCU.RX_PDUs.BMU_FLTRPT.IBMU_FltRptPkCurrUnder", "AEthernet.InfoT_Powertrain.TCU.RX_PDUs.BMU_FLTRPT.IBMU_FltRptPrechrg", "AEthernet.InfoT_Powertrain.TCU.RX_PDUs.BMU_FLTRPT.IBMU_FltRptStSenClsd", "AEthernet.InfoT_Powertrain.TCU.RX_PDUs.BMU_FLTRPT.IBMU_FltRptTempCellOver", "AEthernet.InfoT_Powertrain.TCU.RX_PDUs.BMU_FLTRPT.IBMU_FltRptTempCellUnder", "AEthernet.InfoT_Powertrain.TCU.RX_PDUs.BMU_FLTRPT.IBMU_FltRptTempInterconOver", "AEthernet.InfoT_Powertrain.TCU.RX_PDUs.BMU_FLTRPT.IBMU_FltRptBlkVoltDelta", "AEthernet.InfoT_Powertrain.TCU.RX_PDUs.BMU_FLTRPT.IBMU_FltRptStSenOpen", "AEthernet.InfoT_Powertrain.TCU.RX_PDUs.BMU_FLTRPT.IBMU_FltRptCrash", "AEthernet.InfoT_Powertrain.TCU.RX_PDUs.BMU_FLTRPT.IBMU_FltRptPyro", "AEthernet.InfoT_Powertrain.TCU.RX_PDUs.BMU_FLTRPT.RX_deltatime", "AEthernet.InfoT_Powertrain.TCU.RX_PDUs.BMU_FLTRPT.RX_time", "AEthernet.InfoT_Powertrain.TCU.RX_PDUs.BMU_LIM_1.IBMU_LimMaxDChrgPwr", "AEthernet.InfoT_Powertrain.TCU.RX_PDUs.BMU_LIM_1.IBMU_LimMaxRgnPwr", "AEthernet.InfoT_Powertrain.TCU.RX_PDUs.BMU_LIM_1.IBMU_LimMaxDChrgCurr", "AEthernet.InfoT_Powertrain.TCU.RX_PDUs.BMU_LIM_1.IBMU_LimMaxRgnCurr", "AEthernet.InfoT_Powertrain.TCU.RX_PDUs.BMU_LIM_1.IBMU_LimCurrTempMax", "AEthernet.InfoT_Powertrain.TCU.RX_PDUs.BMU_LIM_1.IBMU_LimCurrTempMin", "AEthernet.InfoT_Powertrain.TCU.RX_PDUs.BMU_LIM_1.IBMU_LimNxtTempMax", "AEthernet.InfoT_Powertrain.TCU.RX_PDUs.BMU_LIM_1.IBMU_LimNxtTempMin", "AEthernet.InfoT_Powertrain.TCU.RX_PDUs.BMU_LIM_1.RX_deltatime", "AEthernet.InfoT_Powertrain.TCU.RX_PDUs.BMU_LIM_1.RX_time", "AEthernet.InfoT_Powertrain.TCU.RX_PDUs.BMU_STATS_1.IBMU_StatsPkHum", "AEthernet.InfoT_Powertrain.TCU.RX_PDUs.BMU_STATS_1.IBMU_StatsPkTempCellMaxBlk", "AEthernet.InfoT_Powertrain.TCU.RX_PDUs.BMU_STATS_1.IBMU_StatsPkTempCellMaxMod", "AEthernet.InfoT_Powertrain.TCU.RX_PDUs.BMU_STATS_1.IBMU_StatsPkTempCellMinBlk", "AEthernet.InfoT_Powertrain.TCU.RX_PDUs.BMU_STATS_1.IBMU_StatsPkTempCellMinMod", "AEthernet.InfoT_Powertrain.TCU.RX_PDUs.BMU_STATS_1.IBMU_StatsTempCellDelta", "AEthernet.InfoT_Powertrain.TCU.RX_PDUs.BMU_STATS_1.IBMU_StatsTempCoolIn", "AEthernet.InfoT_Powertrain.TCU.RX_PDUs.BMU_STATS_1.IBMU_StatsPkBlkVoltDelta", "AEthernet.InfoT_Powertrain.TCU.RX_PDUs.BMU_STATS_1.IBMU_StatsHvTemp1", "AEthernet.InfoT_Powertrain.TCU.RX_PDUs.BMU_STATS_1.IBMU_StatsHvTemp2", "AEthernet.InfoT_Powertrain.TCU.RX_PDUs.BMU_STATS_1.IBMU_StatsHvTemp3", "AEthernet.InfoT_Powertrain.TCU.RX_PDUs.BMU_STATS_1.IBMU_StatsHvTemp4", "AEthernet.InfoT_Powertrain.TCU.RX_PDUs.BMU_STATS_1.IBMU_StatsHvTemp5", "AEthernet.InfoT_Powertrain.TCU.RX_PDUs.BMU_STATS_1.IBMU_StatsHvTemp6", "AEthernet.InfoT_Powertrain.TCU.RX_PDUs.BMU_STATS_1.IBMU_StatsHvTemp7", "AEthernet.InfoT_Powertrain.TCU.RX_PDUs.BMU_STATS_1.IBMU_StatsHvTemp8", "AEthernet.InfoT_Powertrain.TCU.RX_PDUs.BMU_STATS_1.IBMU_StatsHvTemp9", "AEthernet.InfoT_Powertrain.TCU.RX_PDUs.BMU_STATS_1.IBMU_StatsHvTemp10", "AEthernet.InfoT_Powertrain.TCU.RX_PDUs.BMU_STATS_1.IBMU_StatsHvTemp11", "AEthernet.InfoT_Powertrain.TCU.RX_PDUs.BMU_STATS_1.IBMU_StatsHvTemp12", "AEthernet.InfoT_Powertrain.TCU.RX_PDUs.BMU_STATS_1.IBMU_StatsHvTemp13", "AEthernet.InfoT_Powertrain.TCU.RX_PDUs.BMU_STATS_1.IBMU_StatsHvTemp14", "AEthernet.InfoT_Powertrain.TCU.RX_PDUs.BMU_STATS_1.IBMU_StatsPkAmbTemp", "AEthernet.InfoT_Powertrain.TCU.RX_PDUs.BMU_STATS_1.IBMU_StatsPkDewPointTemp", "AEthernet.InfoT_Powertrain.TCU.RX_PDUs.BMU_STATS_1.IBMU_StatsPkTempInterconMax", "AEthernet.InfoT_Powertrain.TCU.RX_PDUs.BMU_STATS_1.IBMU_StatsPkTempInterconMin", "AEthernet.InfoT_Powertrain.TCU.RX_PDUs.BMU_STATS_1.IBMU_StatsPkTempCellMax", "AEthernet.InfoT_Powertrain.TCU.RX_PDUs.BMU_STATS_1.IBMU_StatsPkTempCellMin", "AEthernet.InfoT_Powertrain.TCU.RX_PDUs.BMU_STATS_1.IBMU_StatsTempCellMax", "AEthernet.InfoT_Powertrain.TCU.RX_PDUs.BMU_STATS_1.IBMU_StatsTempCellMin", "AEthernet.InfoT_Powertrain.TCU.RX_PDUs.BMU_STATS_1.IBMU_StatsPkBlkVoltMax0", "AEthernet.InfoT_Powertrain.TCU.RX_PDUs.BMU_STATS_1.IBMU_StatsPkBlkVoltMax0Blk", "AEthernet.InfoT_Powertrain.TCU.RX_PDUs.BMU_STATS_1.IBMU_StatsPkBlkVoltMax0Mod", "AEthernet.InfoT_Powertrain.TCU.RX_PDUs.BMU_STATS_1.IBMU_StatsPkBlkVoltMax1", "AEthernet.InfoT_Powertrain.TCU.RX_PDUs.BMU_STATS_1.IBMU_StatsPkBlkVoltMax1Blk", "AEthernet.InfoT_Powertrain.TCU.RX_PDUs.BMU_STATS_1.IBMU_StatsPkBlkVoltMax1Mod", "AEthernet.InfoT_Powertrain.TCU.RX_PDUs.BMU_STATS_1.IBMU_StatsPkBlkVoltMax2", "AEthernet.InfoT_Powertrain.TCU.RX_PDUs.BMU_STATS_1.IBMU_StatsPkBlkVoltMax2Blk", "AEthernet.InfoT_Powertrain.TCU.RX_PDUs.BMU_STATS_1.IBMU_StatsPkBlkVoltMax2Mod", "AEthernet.InfoT_Powertrain.TCU.RX_PDUs.BMU_STATS_1.IBMU_StatsPkBlkVoltMax3", "AEthernet.InfoT_Powertrain.TCU.RX_PDUs.BMU_STATS_1.IBMU_StatsPkBlkVoltMax3Blk", "AEthernet.InfoT_Powertrain.TCU.RX_PDUs.BMU_STATS_1.IBMU_StatsPkBlkVoltMax3Mod", "AEthernet.InfoT_Powertrain.TCU.RX_PDUs.BMU_STATS_1.IBMU_StatsPkBlkVoltMin0", "AEthernet.InfoT_Powertrain.TCU.RX_PDUs.BMU_STATS_1.IBMU_StatsPkBlkVoltMin0Blk", "AEthernet.InfoT_Powertrain.TCU.RX_PDUs.BMU_STATS_1.IBMU_StatsPkBlkVoltMin0Mod", "AEthernet.InfoT_Powertrain.TCU.RX_PDUs.BMU_STATS_1.IBMU_StatsPkBlkVoltMin1", "AEthernet.InfoT_Powertrain.TCU.RX_PDUs.BMU_STATS_1.IBMU_StatsPkBlkVoltMin1Blk", "AEthernet.InfoT_Powertrain.TCU.RX_PDUs.BMU_STATS_1.IBMU_StatsPkBlkVoltMin1Mod", "AEthernet.InfoT_Powertrain.TCU.RX_PDUs.BMU_STATS_1.IBMU_StatsPkBlkVoltMin2", "AEthernet.InfoT_Powertrain.TCU.RX_PDUs.BMU_STATS_1.IBMU_StatsPkBlkVoltMin2Blk", "AEthernet.InfoT_Powertrain.TCU.RX_PDUs.BMU_STATS_1.IBMU_StatsPkBlkVoltMin2Mod", "AEthernet.InfoT_Powertrain.TCU.RX_PDUs.BMU_STATS_1.IBMU_StatsPkBlkVoltMin3", "AEthernet.InfoT_Powertrain.TCU.RX_PDUs.BMU_STATS_1.IBMU_StatsPkBlkVoltMin3Blk", "AEthernet.InfoT_Powertrain.TCU.RX_PDUs.BMU_STATS_1.IBMU_StatsPkBlkVoltMin3Mod", "AEthernet.InfoT_Powertrain.TCU.RX_PDUs.BMU_STATS_1.IBMU_StatsPkP", "AEthernet.InfoT_Powertrain.TCU.RX_PDUs.BMU_STATS_1.RX_deltatime", "AEthernet.InfoT_Powertrain.TCU.RX_PDUs.BMU_STATS_1.RX_time", "AEthernet.InfoT_Powertrain.TCU.RX_PDUs.BMU_STATS_2.IBMU_StatsPkCurr", "AEthernet.InfoT_Powertrain.TCU.RX_PDUs.BMU_STATS_2.IBMU_StatsPkVbatt", "AEthernet.InfoT_Powertrain.TCU.RX_PDUs.BMU_STATS_2.IBMU_StatsPkVout", "AEthernet.InfoT_Powertrain.TCU.RX_PDUs.BMU_STATS_2.IBMU_StatsPkVbattsum", "AEthernet.InfoT_Powertrain.TCU.RX_PDUs.BMU_STATS_2.IBMU_StatsPkCurrUnsyncd", "AEthernet.InfoT_Powertrain.TCU.RX_PDUs.BMU_STATS_2.IBMU_StatsPkIso", "AEthernet.InfoT_Powertrain.TCU.RX_PDUs.BMU_STATS_2.IBMU_StatsPkPwr", "AEthernet.InfoT_Powertrain.TCU.RX_PDUs.BMU_STATS_2.RX_deltatime", "AEthernet.InfoT_Powertrain.TCU.RX_PDUs.BMU_STATS_2.RX_time", "AEthernet.InfoT_Powertrain.MCU_R.RX_PDUs.BMU_STATS_2.IBMU_StatsPkCurr", "AEthernet.InfoT_Powertrain.MCU_R.RX_PDUs.BMU_STATS_2.IBMU_StatsPkVbatt", "AEthernet.InfoT_Powertrain.MCU_R.RX_PDUs.BMU_STATS_2.IBMU_StatsPkVout", "AEthernet.InfoT_Powertrain.MCU_R.RX_PDUs.BMU_STATS_2.IBMU_StatsPkVbattsum", "AEthernet.InfoT_Powertrain.MCU_R.RX_PDUs.BMU_STATS_2.IBMU_StatsPkCurrUnsyncd", "AEthernet.InfoT_Powertrain.MCU_R.RX_PDUs.BMU_STATS_2.IBMU_StatsPkIso", "AEthernet.InfoT_Powertrain.MCU_R.RX_PDUs.BMU_STATS_2.IBMU_StatsPkPwr", "AEthernet.InfoT_Powertrain.MCU_R.RX_PDUs.BMU_STATS_2.RX_deltatime", "AEthernet.InfoT_Powertrain.MCU_R.RX_PDUs.BMU_STATS_2.RX_time", "AEthernet.InfoT_Powertrain.MCU_F.RX_PDUs.BMU_STATS_2.IBMU_StatsPkCurr", "AEthernet.InfoT_Powertrain.MCU_F.RX_PDUs.BMU_STATS_2.IBMU_StatsPkVbatt", "AEthernet.InfoT_Powertrain.MCU_F.RX_PDUs.BMU_STATS_2.IBMU_StatsPkVout", "AEthernet.InfoT_Powertrain.MCU_F.RX_PDUs.BMU_STATS_2.IBMU_StatsPkVbattsum", "AEthernet.InfoT_Powertrain.MCU_F.RX_PDUs.BMU_STATS_2.IBMU_StatsPkCurrUnsyncd", "AEthernet.InfoT_Powertrain.MCU_F.RX_PDUs.BMU_STATS_2.IBMU_StatsPkIso", "AEthernet.InfoT_Powertrain.MCU_F.RX_PDUs.BMU_STATS_2.IBMU_StatsPkPwr", "AEthernet.InfoT_Powertrain.MCU_F.RX_PDUs.BMU_STATS_2.RX_deltatime", "AEthernet.InfoT_Powertrain.MCU_F.RX_PDUs.BMU_STATS_2.RX_time", "AEthernet.InfoT_Powertrain.ICC.RX_PDUs.BMU_FLTRPT.IBMU_FltRptBlkVoltOver", "AEthernet.InfoT_Powertrain.ICC.RX_PDUs.BMU_FLTRPT.IBMU_FltRptBlkVoltUnder", "AEthernet.InfoT_Powertrain.ICC.RX_PDUs.BMU_FLTRPT.IBMU_FltRptHvil", "AEthernet.InfoT_Powertrain.ICC.RX_PDUs.BMU_FLTRPT.IBMU_FltRptIso", "AEthernet.InfoT_Powertrain.ICC.RX_PDUs.BMU_FLTRPT.IBMU_FltRptPkCurrOver", "AEthernet.InfoT_Powertrain.ICC.RX_PDUs.BMU_FLTRPT.IBMU_FltRptPkCurrUnder", "AEthernet.InfoT_Powertrain.ICC.RX_PDUs.BMU_FLTRPT.IBMU_FltRptPrechrg", "AEthernet.InfoT_Powertrain.ICC.RX_PDUs.BMU_FLTRPT.IBMU_FltRptStSenClsd", "AEthernet.InfoT_Powertrain.ICC.RX_PDUs.BMU_FLTRPT.IBMU_FltRptTempCellOver", "AEthernet.InfoT_Powertrain.ICC.RX_PDUs.BMU_FLTRPT.IBMU_FltRptTempCellUnder", "AEthernet.InfoT_Powertrain.ICC.RX_PDUs.BMU_FLTRPT.IBMU_FltRptTempInterconOver", "AEthernet.InfoT_Powertrain.ICC.RX_PDUs.BMU_FLTRPT.IBMU_FltRptBlkVoltDelta", "AEthernet.InfoT_Powertrain.ICC.RX_PDUs.BMU_FLTRPT.IBMU_FltRptStSenOpen", "AEthernet.InfoT_Powertrain.ICC.RX_PDUs.BMU_FLTRPT.IBMU_FltRptCrash", "AEthernet.InfoT_Powertrain.ICC.RX_PDUs.BMU_FLTRPT.IBMU_FltRptPyro", "AEthernet.InfoT_Powertrain.ICC.RX_PDUs.BMU_FLTRPT.RX_deltatime", "AEthernet.InfoT_Powertrain.ICC.RX_PDUs.BMU_FLTRPT.RX_time", "AEthernet.InfoT_Powertrain.ICC.RX_PDUs.BMU_LIM_1.IBMU_LimMaxDChrgPwr", "AEthernet.InfoT_Powertrain.ICC.RX_PDUs.BMU_LIM_1.IBMU_LimMaxRgnPwr", "AEthernet.InfoT_Powertrain.ICC.RX_PDUs.BMU_LIM_1.IBMU_LimMaxDChrgCurr", "AEthernet.InfoT_Powertrain.ICC.RX_PDUs.BMU_LIM_1.IBMU_LimMaxRgnCurr", "AEthernet.InfoT_Powertrain.ICC.RX_PDUs.BMU_LIM_1.IBMU_LimCurrTempMax", "AEthernet.InfoT_Powertrain.ICC.RX_PDUs.BMU_LIM_1.IBMU_LimCurrTempMin", "AEthernet.InfoT_Powertrain.ICC.RX_PDUs.BMU_LIM_1.IBMU_LimNxtTempMax", "AEthernet.InfoT_Powertrain.ICC.RX_PDUs.BMU_LIM_1.IBMU_LimNxtTempMin", "AEthernet.InfoT_Powertrain.ICC.RX_PDUs.BMU_LIM_1.RX_deltatime", "AEthernet.InfoT_Powertrain.ICC.RX_PDUs.BMU_LIM_1.RX_time", "AEthernet.InfoT_Powertrain.ICC.RX_PDUs.BMU_STATS_1.IBMU_StatsPkHum", "AEthernet.InfoT_Powertrain.ICC.RX_PDUs.BMU_STATS_1.IBMU_StatsPkTempCellMaxBlk", "AEthernet.InfoT_Powertrain.ICC.RX_PDUs.BMU_STATS_1.IBMU_StatsPkTempCellMaxMod", "AEthernet.InfoT_Powertrain.ICC.RX_PDUs.BMU_STATS_1.IBMU_StatsPkTempCellMinBlk", "AEthernet.InfoT_Powertrain.ICC.RX_PDUs.BMU_STATS_1.IBMU_StatsPkTempCellMinMod", "AEthernet.InfoT_Powertrain.ICC.RX_PDUs.BMU_STATS_1.IBMU_StatsTempCellDelta", "AEthernet.InfoT_Powertrain.ICC.RX_PDUs.BMU_STATS_1.IBMU_StatsTempCoolIn", "AEthernet.InfoT_Powertrain.ICC.RX_PDUs.BMU_STATS_1.IBMU_StatsPkBlkVoltDelta", "AEthernet.InfoT_Powertrain.ICC.RX_PDUs.BMU_STATS_1.IBMU_StatsHvTemp1", "AEthernet.InfoT_Powertrain.ICC.RX_PDUs.BMU_STATS_1.IBMU_StatsHvTemp2", "AEthernet.InfoT_Powertrain.ICC.RX_PDUs.BMU_STATS_1.IBMU_StatsHvTemp3", "AEthernet.InfoT_Powertrain.ICC.RX_PDUs.BMU_STATS_1.IBMU_StatsHvTemp4", "AEthernet.InfoT_Powertrain.ICC.RX_PDUs.BMU_STATS_1.IBMU_StatsHvTemp5", "AEthernet.InfoT_Powertrain.ICC.RX_PDUs.BMU_STATS_1.IBMU_StatsHvTemp6", "AEthernet.InfoT_Powertrain.ICC.RX_PDUs.BMU_STATS_1.IBMU_StatsHvTemp7", "AEthernet.InfoT_Powertrain.ICC.RX_PDUs.BMU_STATS_1.IBMU_StatsHvTemp8", "AEthernet.InfoT_Powertrain.ICC.RX_PDUs.BMU_STATS_1.IBMU_StatsHvTemp9", "AEthernet.InfoT_Powertrain.ICC.RX_PDUs.BMU_STATS_1.IBMU_StatsHvTemp10", "AEthernet.InfoT_Powertrain.ICC.RX_PDUs.BMU_STATS_1.IBMU_StatsHvTemp11", "AEthernet.InfoT_Powertrain.ICC.RX_PDUs.BMU_STATS_1.IBMU_StatsHvTemp12", "AEthernet.InfoT_Powertrain.ICC.RX_PDUs.BMU_STATS_1.IBMU_StatsHvTemp13", "AEthernet.InfoT_Powertrain.ICC.RX_PDUs.BMU_STATS_1.IBMU_StatsHvTemp14", "AEthernet.InfoT_Powertrain.ICC.RX_PDUs.BMU_STATS_1.IBMU_StatsPkAmbTemp", "AEthernet.InfoT_Powertrain.ICC.RX_PDUs.BMU_STATS_1.IBMU_StatsPkDewPointTemp", "AEthernet.InfoT_Powertrain.ICC.RX_PDUs.BMU_STATS_1.IBMU_StatsPkTempInterconMax", "AEthernet.InfoT_Powertrain.ICC.RX_PDUs.BMU_STATS_1.IBMU_StatsPkTempInterconMin", "AEthernet.InfoT_Powertrain.ICC.RX_PDUs.BMU_STATS_1.IBMU_StatsPkTempCellMax", "AEthernet.InfoT_Powertrain.ICC.RX_PDUs.BMU_STATS_1.IBMU_StatsPkTempCellMin", "AEthernet.InfoT_Powertrain.ICC.RX_PDUs.BMU_STATS_1.IBMU_StatsTempCellMax", "AEthernet.InfoT_Powertrain.ICC.RX_PDUs.BMU_STATS_1.IBMU_StatsTempCellMin", "AEthernet.InfoT_Powertrain.ICC.RX_PDUs.BMU_STATS_1.IBMU_StatsPkBlkVoltMax0", "AEthernet.InfoT_Powertrain.ICC.RX_PDUs.BMU_STATS_1.IBMU_StatsPkBlkVoltMax0Blk", "AEthernet.InfoT_Powertrain.ICC.RX_PDUs.BMU_STATS_1.IBMU_StatsPkBlkVoltMax0Mod", "AEthernet.InfoT_Powertrain.ICC.RX_PDUs.BMU_STATS_1.IBMU_StatsPkBlkVoltMax1", "AEthernet.InfoT_Powertrain.ICC.RX_PDUs.BMU_STATS_1.IBMU_StatsPkBlkVoltMax1Blk", "AEthernet.InfoT_Powertrain.ICC.RX_PDUs.BMU_STATS_1.IBMU_StatsPkBlkVoltMax1Mod", "AEthernet.InfoT_Powertrain.ICC.RX_PDUs.BMU_STATS_1.IBMU_StatsPkBlkVoltMax2", "AEthernet.InfoT_Powertrain.ICC.RX_PDUs.BMU_STATS_1.IBMU_StatsPkBlkVoltMax2Blk", "AEthernet.InfoT_Powertrain.ICC.RX_PDUs.BMU_STATS_1.IBMU_StatsPkBlkVoltMax2Mod", "AEthernet.InfoT_Powertrain.ICC.RX_PDUs.BMU_STATS_1.IBMU_StatsPkBlkVoltMax3", "AEthernet.InfoT_Powertrain.ICC.RX_PDUs.BMU_STATS_1.IBMU_StatsPkBlkVoltMax3Blk", "AEthernet.InfoT_Powertrain.ICC.RX_PDUs.BMU_STATS_1.IBMU_StatsPkBlkVoltMax3Mod", "AEthernet.InfoT_Powertrain.ICC.RX_PDUs.BMU_STATS_1.IBMU_StatsPkBlkVoltMin0", "AEthernet.InfoT_Powertrain.ICC.RX_PDUs.BMU_STATS_1.IBMU_StatsPkBlkVoltMin0Blk", "AEthernet.InfoT_Powertrain.ICC.RX_PDUs.BMU_STATS_1.IBMU_StatsPkBlkVoltMin0Mod", "AEthernet.InfoT_Powertrain.ICC.RX_PDUs.BMU_STATS_1.IBMU_StatsPkBlkVoltMin1", "AEthernet.InfoT_Powertrain.ICC.RX_PDUs.BMU_STATS_1.IBMU_StatsPkBlkVoltMin1Blk", "AEthernet.InfoT_Powertrain.ICC.RX_PDUs.BMU_STATS_1.IBMU_StatsPkBlkVoltMin1Mod", "AEthernet.InfoT_Powertrain.ICC.RX_PDUs.BMU_STATS_1.IBMU_StatsPkBlkVoltMin2", "AEthernet.InfoT_Powertrain.ICC.RX_PDUs.BMU_STATS_1.IBMU_StatsPkBlkVoltMin2Blk", "AEthernet.InfoT_Powertrain.ICC.RX_PDUs.BMU_STATS_1.IBMU_StatsPkBlkVoltMin2Mod", "AEthernet.InfoT_Powertrain.ICC.RX_PDUs.BMU_STATS_1.IBMU_StatsPkBlkVoltMin3", "AEthernet.InfoT_Powertrain.ICC.RX_PDUs.BMU_STATS_1.IBMU_StatsPkBlkVoltMin3Blk", "AEthernet.InfoT_Powertrain.ICC.RX_PDUs.BMU_STATS_1.IBMU_StatsPkBlkVoltMin3Mod", "AEthernet.InfoT_Powertrain.ICC.RX_PDUs.BMU_STATS_1.IBMU_StatsPkP", "AEthernet.InfoT_Powertrain.ICC.RX_PDUs.BMU_STATS_1.RX_deltatime", "AEthernet.InfoT_Powertrain.ICC.RX_PDUs.BMU_STATS_1.RX_time", "AEthernet.InfoT_Powertrain.ICC.RX_PDUs.BMU_STATS_2.IBMU_StatsPkCurr", "AEthernet.InfoT_Powertrain.ICC.RX_PDUs.BMU_STATS_2.IBMU_StatsPkVbatt", "AEthernet.InfoT_Powertrain.ICC.RX_PDUs.BMU_STATS_2.IBMU_StatsPkVout", "AEthernet.InfoT_Powertrain.ICC.RX_PDUs.BMU_STATS_2.IBMU_StatsPkVbattsum", "AEthernet.InfoT_Powertrain.ICC.RX_PDUs.BMU_STATS_2.IBMU_StatsPkCurrUnsyncd", "AEthernet.InfoT_Powertrain.ICC.RX_PDUs.BMU_STATS_2.IBMU_StatsPkIso", "AEthernet.InfoT_Powertrain.ICC.RX_PDUs.BMU_STATS_2.IBMU_StatsPkPwr", "AEthernet.InfoT_Powertrain.ICC.RX_PDUs.BMU_STATS_2.RX_deltatime", "AEthernet.InfoT_Powertrain.ICC.RX_PDUs.BMU_STATS_2.RX_time", "AEthernet.InfoT_Powertrain.CCC.RX_PDUs.BMU_FLTRPT.IBMU_FltRptBlkVoltOver", "AEthernet.InfoT_Powertrain.CCC.RX_PDUs.BMU_FLTRPT.IBMU_FltRptBlkVoltUnder", "AEthernet.InfoT_Powertrain.CCC.RX_PDUs.BMU_FLTRPT.IBMU_FltRptHvil", "AEthernet.InfoT_Powertrain.CCC.RX_PDUs.BMU_FLTRPT.IBMU_FltRptIso", "AEthernet.InfoT_Powertrain.CCC.RX_PDUs.BMU_FLTRPT.IBMU_FltRptPkCurrOver", "AEthernet.InfoT_Powertrain.CCC.RX_PDUs.BMU_FLTRPT.IBMU_FltRptPkCurrUnder", "AEthernet.InfoT_Powertrain.CCC.RX_PDUs.BMU_FLTRPT.IBMU_FltRptPrechrg", "AEthernet.InfoT_Powertrain.CCC.RX_PDUs.BMU_FLTRPT.IBMU_FltRptStSenClsd", "AEthernet.InfoT_Powertrain.CCC.RX_PDUs.BMU_FLTRPT.IBMU_FltRptTempCellOver", "AEthernet.InfoT_Powertrain.CCC.RX_PDUs.BMU_FLTRPT.IBMU_FltRptTempCellUnder", "AEthernet.InfoT_Powertrain.CCC.RX_PDUs.BMU_FLTRPT.IBMU_FltRptTempInterconOver", "AEthernet.InfoT_Powertrain.CCC.RX_PDUs.BMU_FLTRPT.IBMU_FltRptBlkVoltDelta", "AEthernet.InfoT_Powertrain.CCC.RX_PDUs.BMU_FLTRPT.IBMU_FltRptStSenOpen", "AEthernet.InfoT_Powertrain.CCC.RX_PDUs.BMU_FLTRPT.IBMU_FltRptCrash", "AEthernet.InfoT_Powertrain.CCC.RX_PDUs.BMU_FLTRPT.IBMU_FltRptPyro", "AEthernet.InfoT_Powertrain.CCC.RX_PDUs.BMU_FLTRPT.RX_deltatime", "AEthernet.InfoT_Powertrain.CCC.RX_PDUs.BMU_FLTRPT.RX_time", "AEthernet.InfoT_Powertrain.CCC.RX_PDUs.BMU_LIM_1.IBMU_LimMaxDChrgPwr", "AEthernet.InfoT_Powertrain.CCC.RX_PDUs.BMU_LIM_1.IBMU_LimMaxRgnPwr", "AEthernet.InfoT_Powertrain.CCC.RX_PDUs.BMU_LIM_1.IBMU_LimMaxDChrgCurr", "AEthernet.InfoT_Powertrain.CCC.RX_PDUs.BMU_LIM_1.IBMU_LimMaxRgnCurr", "AEthernet.InfoT_Powertrain.CCC.RX_PDUs.BMU_LIM_1.IBMU_LimCurrTempMax", "AEthernet.InfoT_Powertrain.CCC.RX_PDUs.BMU_LIM_1.IBMU_LimCurrTempMin", "AEthernet.InfoT_Powertrain.CCC.RX_PDUs.BMU_LIM_1.IBMU_LimNxtTempMax", "AEthernet.InfoT_Powertrain.CCC.RX_PDUs.BMU_LIM_1.IBMU_LimNxtTempMin", "AEthernet.InfoT_Powertrain.CCC.RX_PDUs.BMU_LIM_1.RX_deltatime", "AEthernet.InfoT_Powertrain.CCC.RX_PDUs.BMU_LIM_1.RX_time", "AEthernet.InfoT_Powertrain.CCC.RX_PDUs.BMU_STATS_1.IBMU_StatsPkHum", "AEthernet.InfoT_Powertrain.CCC.RX_PDUs.BMU_STATS_1.IBMU_StatsPkTempCellMaxBlk", "AEthernet.InfoT_Powertrain.CCC.RX_PDUs.BMU_STATS_1.IBMU_StatsPkTempCellMaxMod", "AEthernet.InfoT_Powertrain.CCC.RX_PDUs.BMU_STATS_1.IBMU_StatsPkTempCellMinBlk", "AEthernet.InfoT_Powertrain.CCC.RX_PDUs.BMU_STATS_1.IBMU_StatsPkTempCellMinMod", "AEthernet.InfoT_Powertrain.CCC.RX_PDUs.BMU_STATS_1.IBMU_StatsTempCellDelta", "AEthernet.InfoT_Powertrain.CCC.RX_PDUs.BMU_STATS_1.IBMU_StatsTempCoolIn", "AEthernet.InfoT_Powertrain.CCC.RX_PDUs.BMU_STATS_1.IBMU_StatsPkBlkVoltDelta", "AEthernet.InfoT_Powertrain.CCC.RX_PDUs.BMU_STATS_1.IBMU_StatsHvTemp1", "AEthernet.InfoT_Powertrain.CCC.RX_PDUs.BMU_STATS_1.IBMU_StatsHvTemp2", "AEthernet.InfoT_Powertrain.CCC.RX_PDUs.BMU_STATS_1.IBMU_StatsHvTemp3", "AEthernet.InfoT_Powertrain.CCC.RX_PDUs.BMU_STATS_1.IBMU_StatsHvTemp4", "AEthernet.InfoT_Powertrain.CCC.RX_PDUs.BMU_STATS_1.IBMU_StatsHvTemp5", "AEthernet.InfoT_Powertrain.CCC.RX_PDUs.BMU_STATS_1.IBMU_StatsHvTemp6", "AEthernet.InfoT_Powertrain.CCC.RX_PDUs.BMU_STATS_1.IBMU_StatsHvTemp7", "AEthernet.InfoT_Powertrain.CCC.RX_PDUs.BMU_STATS_1.IBMU_StatsHvTemp8", "AEthernet.InfoT_Powertrain.CCC.RX_PDUs.BMU_STATS_1.IBMU_StatsHvTemp9", "AEthernet.InfoT_Powertrain.CCC.RX_PDUs.BMU_STATS_1.IBMU_StatsHvTemp10", "AEthernet.InfoT_Powertrain.CCC.RX_PDUs.BMU_STATS_1.IBMU_StatsHvTemp11", "AEthernet.InfoT_Powertrain.CCC.RX_PDUs.BMU_STATS_1.IBMU_StatsHvTemp12", "AEthernet.InfoT_Powertrain.CCC.RX_PDUs.BMU_STATS_1.IBMU_StatsHvTemp13", "AEthernet.InfoT_Powertrain.CCC.RX_PDUs.BMU_STATS_1.IBMU_StatsHvTemp14", "AEthernet.InfoT_Powertrain.CCC.RX_PDUs.BMU_STATS_1.IBMU_StatsPkAmbTemp", "AEthernet.InfoT_Powertrain.CCC.RX_PDUs.BMU_STATS_1.IBMU_StatsPkDewPointTemp", "AEthernet.InfoT_Powertrain.CCC.RX_PDUs.BMU_STATS_1.IBMU_StatsPkTempInterconMax", "AEthernet.InfoT_Powertrain.CCC.RX_PDUs.BMU_STATS_1.IBMU_StatsPkTempInterconMin", "AEthernet.InfoT_Powertrain.CCC.RX_PDUs.BMU_STATS_1.IBMU_StatsPkTempCellMax", "AEthernet.InfoT_Powertrain.CCC.RX_PDUs.BMU_STATS_1.IBMU_StatsPkTempCellMin", "AEthernet.InfoT_Powertrain.CCC.RX_PDUs.BMU_STATS_1.IBMU_StatsTempCellMax", "AEthernet.InfoT_Powertrain.CCC.RX_PDUs.BMU_STATS_1.IBMU_StatsTempCellMin", "AEthernet.InfoT_Powertrain.CCC.RX_PDUs.BMU_STATS_1.IBMU_StatsPkBlkVoltMax0", "AEthernet.InfoT_Powertrain.CCC.RX_PDUs.BMU_STATS_1.IBMU_StatsPkBlkVoltMax0Blk", "AEthernet.InfoT_Powertrain.CCC.RX_PDUs.BMU_STATS_1.IBMU_StatsPkBlkVoltMax0Mod", "AEthernet.InfoT_Powertrain.CCC.RX_PDUs.BMU_STATS_1.IBMU_StatsPkBlkVoltMax1", "AEthernet.InfoT_Powertrain.CCC.RX_PDUs.BMU_STATS_1.IBMU_StatsPkBlkVoltMax1Blk", "AEthernet.InfoT_Powertrain.CCC.RX_PDUs.BMU_STATS_1.IBMU_StatsPkBlkVoltMax1Mod", "AEthernet.InfoT_Powertrain.CCC.RX_PDUs.BMU_STATS_1.IBMU_StatsPkBlkVoltMax2", "AEthernet.InfoT_Powertrain.CCC.RX_PDUs.BMU_STATS_1.IBMU_StatsPkBlkVoltMax2Blk", "AEthernet.InfoT_Powertrain.CCC.RX_PDUs.BMU_STATS_1.IBMU_StatsPkBlkVoltMax2Mod", "AEthernet.InfoT_Powertrain.CCC.RX_PDUs.BMU_STATS_1.IBMU_StatsPkBlkVoltMax3", "AEthernet.InfoT_Powertrain.CCC.RX_PDUs.BMU_STATS_1.IBMU_StatsPkBlkVoltMax3Blk", "AEthernet.InfoT_Powertrain.CCC.RX_PDUs.BMU_STATS_1.IBMU_StatsPkBlkVoltMax3Mod", "AEthernet.InfoT_Powertrain.CCC.RX_PDUs.BMU_STATS_1.IBMU_StatsPkBlkVoltMin0", "AEthernet.InfoT_Powertrain.CCC.RX_PDUs.BMU_STATS_1.IBMU_StatsPkBlkVoltMin0Blk", "AEthernet.InfoT_Powertrain.CCC.RX_PDUs.BMU_STATS_1.IBMU_StatsPkBlkVoltMin0Mod", "AEthernet.InfoT_Powertrain.CCC.RX_PDUs.BMU_STATS_1.IBMU_StatsPkBlkVoltMin1", "AEthernet.InfoT_Powertrain.CCC.RX_PDUs.BMU_STATS_1.IBMU_StatsPkBlkVoltMin1Blk", "AEthernet.InfoT_Powertrain.CCC.RX_PDUs.BMU_STATS_1.IBMU_StatsPkBlkVoltMin1Mod", "AEthernet.InfoT_Powertrain.CCC.RX_PDUs.BMU_STATS_1.IBMU_StatsPkBlkVoltMin2", "AEthernet.InfoT_Powertrain.CCC.RX_PDUs.BMU_STATS_1.IBMU_StatsPkBlkVoltMin2Blk", "AEthernet.InfoT_Powertrain.CCC.RX_PDUs.BMU_STATS_1.IBMU_StatsPkBlkVoltMin2Mod", "AEthernet.InfoT_Powertrain.CCC.RX_PDUs.BMU_STATS_1.IBMU_StatsPkBlkVoltMin3", "AEthernet.InfoT_Powertrain.CCC.RX_PDUs.BMU_STATS_1.IBMU_StatsPkBlkVoltMin3Blk", "AEthernet.InfoT_Powertrain.CCC.RX_PDUs.BMU_STATS_1.IBMU_StatsPkBlkVoltMin3Mod", "AEthernet.InfoT_Powertrain.CCC.RX_PDUs.BMU_STATS_1.IBMU_StatsPkP", "AEthernet.InfoT_Powertrain.CCC.RX_PDUs.BMU_STATS_1.RX_deltatime", "AEthernet.InfoT_Powertrain.CCC.RX_PDUs.BMU_STATS_1.RX_time", "AEthernet.InfoT_Powertrain.CCC.RX_PDUs.BMU_STATS_2.IBMU_StatsPkCurr", "AEthernet.InfoT_Powertrain.CCC.RX_PDUs.BMU_STATS_2.IBMU_StatsPkVbatt", "AEthernet.InfoT_Powertrain.CCC.RX_PDUs.BMU_STATS_2.IBMU_StatsPkVout", "AEthernet.InfoT_Powertrain.CCC.RX_PDUs.BMU_STATS_2.IBMU_StatsPkVbattsum", "AEthernet.InfoT_Powertrain.CCC.RX_PDUs.BMU_STATS_2.IBMU_StatsPkCurrUnsyncd", "AEthernet.InfoT_Powertrain.CCC.RX_PDUs.BMU_STATS_2.IBMU_StatsPkIso", "AEthernet.InfoT_Powertrain.CCC.RX_PDUs.BMU_STATS_2.IBMU_StatsPkPwr", "AEthernet.InfoT_Powertrain.CCC.RX_PDUs.BMU_STATS_2.RX_deltatime", "AEthernet.InfoT_Powertrain.CCC.RX_PDUs.BMU_STATS_2.RX_time", "AEthernet.Powertrain.TCU.RX_PDUs.BMU_CHRG_1.IBMU_ChrgProfEntryLen", "AEthernet.Powertrain.TCU.RX_PDUs.BMU_CHRG_1.IBMU_ChrgProfPwr0", "AEthernet.Powertrain.TCU.RX_PDUs.BMU_CHRG_1.IBMU_ChrgProfPwr1", "AEthernet.Powertrain.TCU.RX_PDUs.BMU_CHRG_1.IBMU_ChrgProfPwr2", "AEthernet.Powertrain.TCU.RX_PDUs.BMU_CHRG_1.IBMU_ChrgProfPwr3", "AEthernet.Powertrain.TCU.RX_PDUs.BMU_CHRG_1.IBMU_ChrgProfPwr4", "AEthernet.Powertrain.TCU.RX_PDUs.BMU_CHRG_1.IBMU_ChrgProfPwr5", "AEthernet.Powertrain.TCU.RX_PDUs.BMU_CHRG_1.IBMU_ChrgProfPwr6", "AEthernet.Powertrain.TCU.RX_PDUs.BMU_CHRG_1.IBMU_ChrgProfPwr7", "AEthernet.Powertrain.TCU.RX_PDUs.BMU_CHRG_1.IBMU_ChrgProfTi0", "AEthernet.Powertrain.TCU.RX_PDUs.BMU_CHRG_1.IBMU_ChrgProfTi1", "AEthernet.Powertrain.TCU.RX_PDUs.BMU_CHRG_1.IBMU_ChrgProfTi2", "AEthernet.Powertrain.TCU.RX_PDUs.BMU_CHRG_1.IBMU_ChrgProfTi3", "AEthernet.Powertrain.TCU.RX_PDUs.BMU_CHRG_1.IBMU_ChrgProfTi4", "AEthernet.Powertrain.TCU.RX_PDUs.BMU_CHRG_1.IBMU_ChrgProfTi5", "AEthernet.Powertrain.TCU.RX_PDUs.BMU_CHRG_1.IBMU_ChrgProfTi6", "AEthernet.Powertrain.TCU.RX_PDUs.BMU_CHRG_1.IBMU_ChrgProfTi7", "AEthernet.Powertrain.TCU.RX_PDUs.BMU_CHRG_1.IBMU_ChrgTarSoc", "AEthernet.Powertrain.TCU.RX_PDUs.BMU_CHRG_1.IBMU_ChrgTarSocBulk", "AEthernet.Powertrain.TCU.RX_PDUs.BMU_CHRG_1.IBMU_ChrgEgyReq", "AEthernet.Powertrain.TCU.RX_PDUs.BMU_CHRG_1.RX_deltatime", "AEthernet.Powertrain.TCU.RX_PDUs.BMU_CHRG_1.RX_time", "AEthernet.Powertrain.MPB.RX_PDUs.BMU_CHRG_1.IBMU_ChrgProfEntryLen", "AEthernet.Powertrain.MPB.RX_PDUs.BMU_CHRG_1.IBMU_ChrgProfPwr0", "AEthernet.Powertrain.MPB.RX_PDUs.BMU_CHRG_1.IBMU_ChrgProfPwr1", "AEthernet.Powertrain.MPB.RX_PDUs.BMU_CHRG_1.IBMU_ChrgProfPwr2", "AEthernet.Powertrain.MPB.RX_PDUs.BMU_CHRG_1.IBMU_ChrgProfPwr3", "AEthernet.Powertrain.MPB.RX_PDUs.BMU_CHRG_1.IBMU_ChrgProfPwr4", "AEthernet.Powertrain.MPB.RX_PDUs.BMU_CHRG_1.IBMU_ChrgProfPwr5", "AEthernet.Powertrain.MPB.RX_PDUs.BMU_CHRG_1.IBMU_ChrgProfPwr6", "AEthernet.Powertrain.MPB.RX_PDUs.BMU_CHRG_1.IBMU_ChrgProfPwr7", "AEthernet.Powertrain.MPB.RX_PDUs.BMU_CHRG_1.IBMU_ChrgProfTi0", "AEthernet.Powertrain.MPB.RX_PDUs.BMU_CHRG_1.IBMU_ChrgProfTi1", "AEthernet.Powertrain.MPB.RX_PDUs.BMU_CHRG_1.IBMU_ChrgProfTi2", "AEthernet.Powertrain.MPB.RX_PDUs.BMU_CHRG_1.IBMU_ChrgProfTi3", "AEthernet.Powertrain.MPB.RX_PDUs.BMU_CHRG_1.IBMU_ChrgProfTi4", "AEthernet.Powertrain.MPB.RX_PDUs.BMU_CHRG_1.IBMU_ChrgProfTi5", "AEthernet.Powertrain.MPB.RX_PDUs.BMU_CHRG_1.IBMU_ChrgProfTi6", "AEthernet.Powertrain.MPB.RX_PDUs.BMU_CHRG_1.IBMU_ChrgProfTi7", "AEthernet.Powertrain.MPB.RX_PDUs.BMU_CHRG_1.IBMU_ChrgTarSoc", "AEthernet.Powertrain.MPB.RX_PDUs.BMU_CHRG_1.IBMU_ChrgTarSocBulk", "AEthernet.Powertrain.MPB.RX_PDUs.BMU_CHRG_1.IBMU_ChrgEgyReq", "AEthernet.Powertrain.MPB.RX_PDUs.BMU_CHRG_1.RX_deltatime", "AEthernet.Powertrain.MPB.RX_PDUs.BMU_CHRG_1.RX_time", "AEthernet.Powertrain.BMU.RX_PDUs.MPB_STS_4.IMPB_BattCurr", "AEthernet.Powertrain.BMU.RX_PDUs.MPB_STS_4.IMPB_BattPortPower", "AEthernet.Powertrain.BMU.RX_PDUs.MPB_STS_4.IMPB_BattVoltgHiRes", "AEthernet.Powertrain.BMU.RX_PDUs.MPB_STS_4.IMPB_ChrgStMacSts", "AEthernet.Powertrain.BMU.RX_PDUs.MPB_STS_4.IMPB_DeratingFactor", "AEthernet.Powertrain.BMU.RX_PDUs.MPB_STS_4.IMPB_EVSESts", "AEthernet.Powertrain.BMU.RX_PDUs.MPB_STS_4.IMPB_EVSEType", "AEthernet.Powertrain.BMU.RX_PDUs.MPB_STS_4.IMPB_DCCurrLim", "AEthernet.Powertrain.BMU.RX_PDUs.MPB_STS_4.RX_deltatime", "AEthernet.Powertrain.BMU.RX_PDUs.MPB_STS_4.RX_time", "AEthernet.Powertrain.BMU.RX_PDUs.MPB_STS_5.IMPB_DCbusVoltg", "AEthernet.Powertrain.BMU.RX_PDUs.MPB_STS_5.IMPB_EVSEACCurrLimit", "AEthernet.Powertrain.BMU.RX_PDUs.MPB_STS_5.IMPB_EVSEACSwitchSts", "AEthernet.Powertrain.BMU.RX_PDUs.MPB_STS_5.IMPB_InletACportCurr", "AEthernet.Powertrain.BMU.RX_PDUs.MPB_STS_5.IMPB_InletACportVoltgHiRes", "AEthernet.Powertrain.BMU.RX_PDUs.MPB_STS_5.IMPB_InletJ1772Sts", "AEthernet.Powertrain.BMU.RX_PDUs.MPB_STS_5.RX_deltatime", "AEthernet.Powertrain.BMU.RX_PDUs.MPB_STS_5.RX_time", "AEthernet.Powertrain.BMU.RX_PDUs.PT_STATE_PDU.IPT_State", "AEthernet.Powertrain.BMU.RX_PDUs.PT_STATE_PDU.RX_deltatime", "AEthernet.Powertrain.BMU.RX_PDUs.PT_STATE_PDU.RX_time", "AEthernet.Powertrain.BMU.RX_PDUs.PT_UPDSAFEST.IPT_UpdSafeSt", "AEthernet.Powertrain.BMU.RX_PDUs.PT_UPDSAFEST.RX_deltatime", "AEthernet.Powertrain.BMU.RX_PDUs.PT_UPDSAFEST.RX_time"] ("names")
  n1 = local write "path not found"(FALSE ("path not found")) -> ()
  n2 = for {
    tunnel: w1 -> [w20] mode=indexing
    tunnel: "signal/tag name" -> [w19]
    tunnel: [w15] -> w12
    tunnel: [w14] -> w8
    i -> [w15]
    stop <- w16 stop-if-true
    n3 = Search and Replace String(input string=w20, search string=w19) -> (offset past replacement=w14:i32)  [unwired: 6 in, 3 out]
    n4 = Equal?(x=w14, y=-1) -> (x = y?=w17:bool)
    n5 = Not(x=w17) -> (.not. x?=w16:bool)
  }
  n6 = Index Array(array=w1, index=w12) -> (element=→"full path name":string)
  n7 = Array Size(array=w1) -> (size(s)=w13:i32)
  n8 = Decrement(x=w13) -> (x-1=w11:i32)
  n9 = Equal?(x=w8, y=-1) -> (x = y?=w6:bool)
  n10 = Equal?(x=w12, y=w11) -> (x = y?=w5:bool)
  n11 = And(x=w6, y=w5) -> (x .and. y?=w4:bool)
  n12 = case "path not found" shown="True" w4 {
    tunnel: "signal/tag name" -> [_ w26]
    tunnel: [FALSE TRUE] -> w3
    frame False {
    }
    frame True {
      n13 = local write "full path name"("") -> ()
      n14 = Concatenate Strings(w26, " path not found" ("string")) -> (w25:string)
      n15 = call "Display Message to User"("Message"=w25) -> ()  [unwired: 9 in, 2 out]
    }
  }
  "path not found" <- w3
